vi "TestMain2.vi"(8 "error in (no error)":errorcluster) -> (0 "error in (out)":errorcluster)   [LabVIEW 2024, in "Test_2.lvlib"]
doc: "This template is for the Queued Message Handler design pattern.\n\nThe Event Handling Loop generates messages based on user interface actions.\n\nThe Message Handling Loop processes messages generated by the Event Handling Loop, or by other messages. The messages are string values, so new messages can be added easily to the Message Cases case structure in the Message Handling Loop. Each message cluster can also provide an optional value for Message Data, which is a variant that can be converted to whatever message-specific data is required."
uses:
  Test_2.lvlib
  Launcher/SubVI/Controls/OEE_CTRL.ctl
  controls/Test UI Data.ctl
  Settings/controls/Setting_Screen UI Data.ctl
  Settings/support/ScriptDetails.ctl
  Settings/support/CurrentStep.ctl
  Settings/support/StepType.ctl
  Settings/support/PS_WRITE.ctl
  Settings/support/PS_set.ctl
  Settings/support/DMM_CONFIG.ctl
  Settings/support/READ_DATAS.ctl
  Settings/support/READ_EQP.ctl
  Settings/support/READ_PARA.ctl
  Settings/support/Relay_Channel_Array.ctl
  Settings/support/Common_plc_DOs.ctl
  Settings/support/DAQ_Config.ctl
  PCANusb_DTU/support/CAN_MSGs.ctl
  PCANusb_DTU/support/CAN_Frames_ctrl.ctl
  PCANusb_DTU/support/Framing datas.ctl
  PCANusb_DTU/support/CAN_Read.ctl
  Settings/support/Camera.ctl
  MCU_Flashing/support/MCU_ctrl.ctl
  Settings/support/Neoway ctl.ctl
  Settings/support/SSL.ctl
  ADAM_DI/support/Relay_enum_IN.ctl
  Relay_Module/support/Relay_Enum_OUT.ctl
  <vilib>/Utility/miscctls.llb/LVRowAndColumnTypeDef.ctl
  <vilib>/Utility/miscctls.llb/LVMinMaxIncTypeDef.ctl
  <vilib>/Utility/miscctls.llb/LVRangeTypeDef.ctl
  Relay_Module/support/Relay_Channel_Write.ctl
  PrivateControls/Test_FGV_Queue_Control.ctl
  <vilib>/Utility/file.llb/Write Delimited Spreadsheet (string).vi
  Launcher/SubVI/Global 1.vi
  <vilib>/Utility/error.llb/Error Cluster From Error Code.vi
  <vilib>/regexp/Match Regular Expression.xnode
  <vilib>/ErrorRing/Error Ring.xnode
  support/Message Queue/Test Message Queue.lvlib
  support/User Event - Stop/Test User Event - Stop.lvlib
  Settings/Setting_Screen.lvlib
  Launcher/Launcher_DTU.lvlib
  Relay_Module/Relay_Module.lvlib
  Barcode_Scanner/Barcode_Scanner.lvlib
  PCANusb_DTU/PCANusb_DTU.lvlib
  ADAM_DI/ADAM_DI.lvlib
  MCU_Flashing/MCU_Flashing.lvlib
  Keyence/Keyence_VS150.lvlib
  SSL_Certification/SSL_Certification.lvlib
  FTPClient/FTPS.lvlib
  AWSEXE/AWSEXE.lvlib
panel:
  out "Total Time(s)":i32
  out "RX/RY":string
  in  "New/Old_Slot":bool
  out "result":bool
  in  "Config":string
  out "Barcodetime":u32
  out "Test Started?":bool
  out "DTU Inspection Data":string
  out "Relay":refnum<queue>
  out "PP":bool
  out "EOL/FCT":bool
  out "element":string
  out "Part Count":T1
  in  "Operator":string
  in  "Start Button":bool
  out "STATUS":bool
  out "Test Progress...":u8(slide) max=0 step=1 scale=-1.0..1.0
  out "Barcode":string
  out "Configs":string
  in  "DUT":i32=1
  in  "Table":string[][](table)
  out "queue name 2":string
  out "queue name":string
  in  "Abort":bool
  in  "Exit":bool
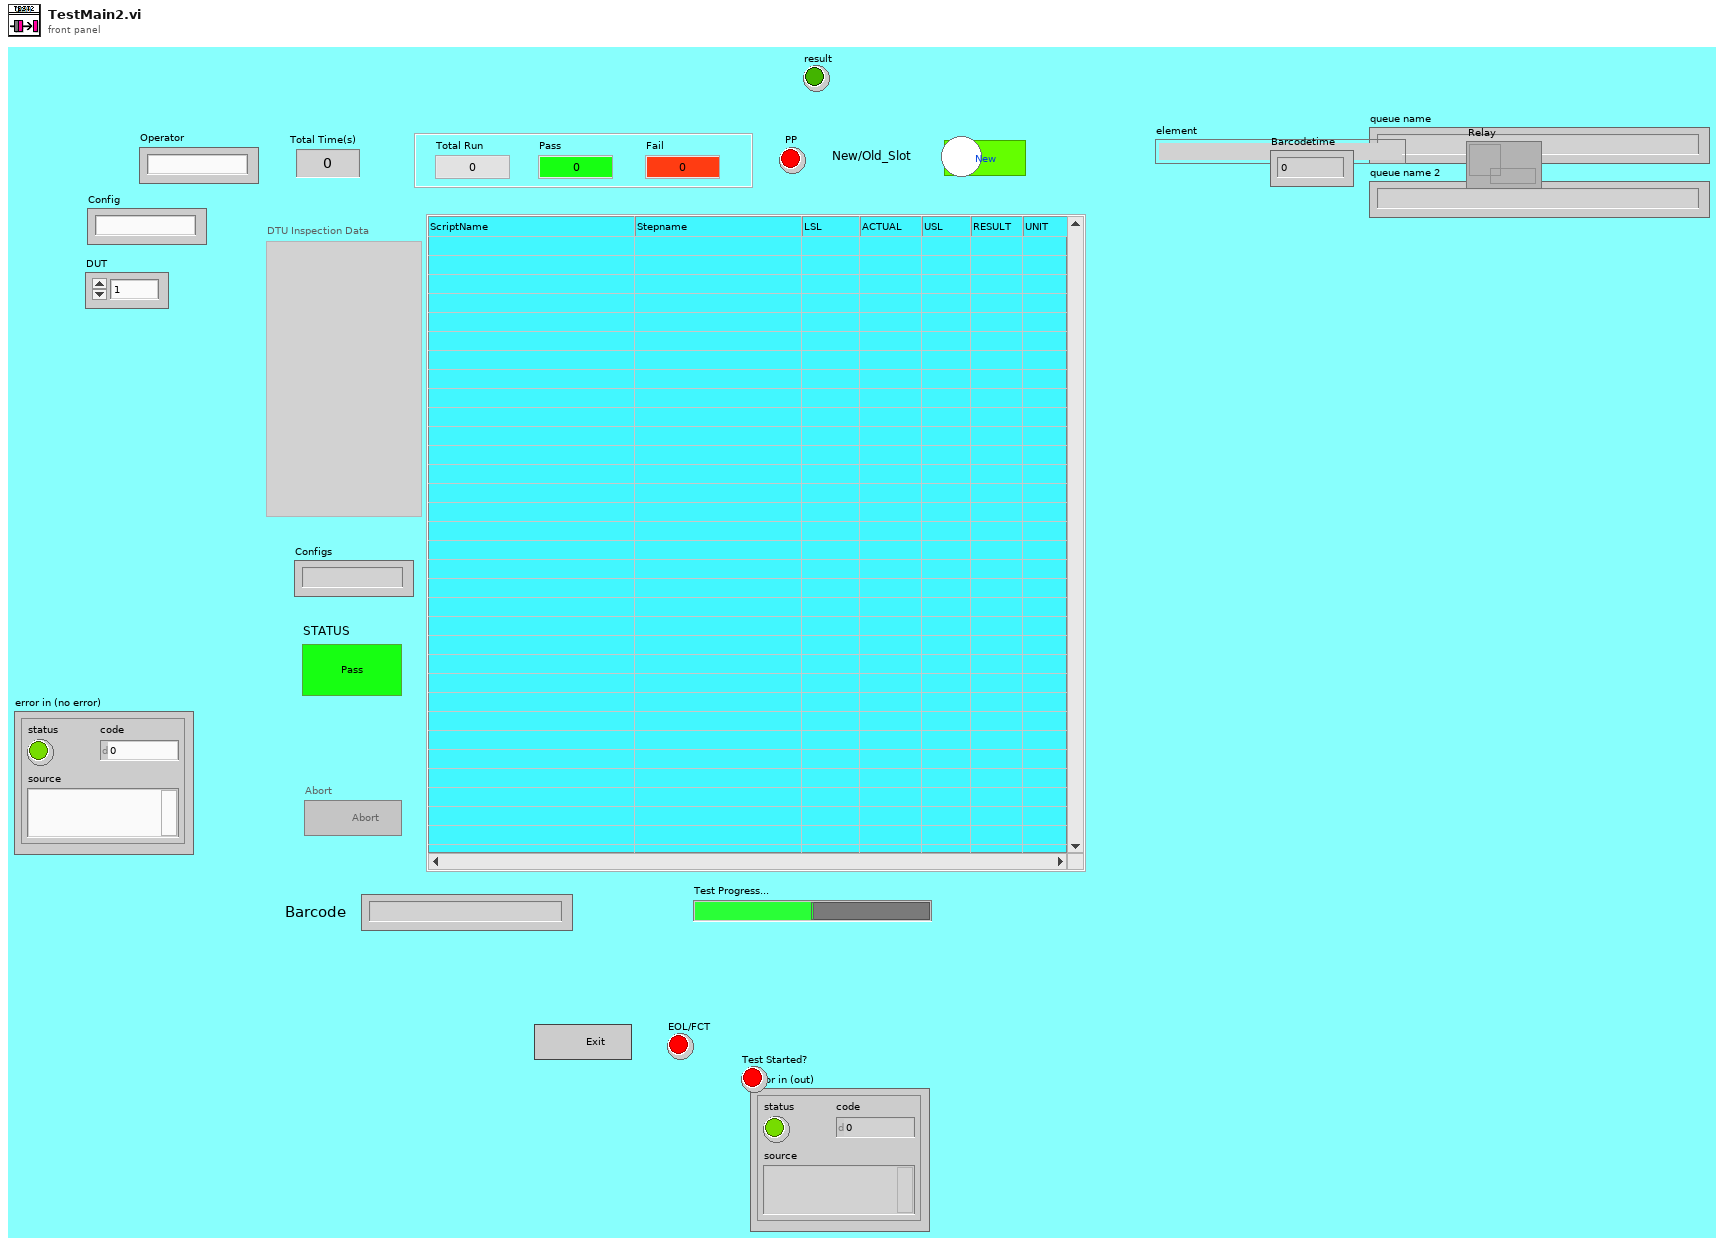
[diagram p1: front panel]
types:
  T1 = typedef "Launcher_DTU.lvlib/OEE_CTRL.ctl" = cluster{"Total Run":i32, "Pass":i32, "Fail":i32}
  T2 = typedef "Test_2.lvlib/Test UI Data.ctl" = cluster{"DUT":i32, "Pass/Fail":string, "Actual":string, "UI Data":T3, "Table":string[][], "Filename":string, "Test Started?":bool, "TotalScripts":u64, "Indexno.":u64, "Stepno.":u64, "TotalSteps":u64, "Scriptno.":u64, "Settings":path, "Data Path":path, "Configuration path":path, "Array_N":refnum<notifier>[], "Message Data":variant, "Stepname":string, "Scriptname":string, "Result":bool, "Header data":string[], "LaunchStep":bool, "Barcode":string, "LSL":string, "Delay":bool, "Delay time":dbl, "Operator":string, "Part Count ":T1, "InitPro":bool, "ResultS":string, "PMC path":path, "Test2_Q":refnum<queue>, "Array_Q":refnum<queue>[], "config":string, "EQUP LIST":string[], "EQUIP Config path":path, "Relay_Module_Q":refnum<queue>, "Barcode Scanned?":bool, "USL":string, "UNIT":string, "Expected_Value":string, "MACID":string, "ICCID":string, "IMEI":string, "Barcodetime":u32, "Seconds":u32, "RX/RY":string, "Selected_Scripts":T4[]}
  T3 = typedef "Setting_Screen.lvlib/Setting_Screen UI Data.ctl" = cluster{"Script_Tree":refnum<vi>, "Scripts":T4[], "ScriptDetails":T4, "Current Step":T5, "ScriptName":string, "StepName":string, "Children Symbols":i32[][], "Parrent Symbol":i32[], "Configurations:":string, "Config":string, "Scriptno.":i32, "PS_Write":T7, "DMM_CONFIG":T9, "READ_DATAS":T10, "Set_Channel_Relay":T13, "DAQ_Config":T15, "CAN_MSGs_Write":T16, "CAN_Read":T19, "Camera":T20, "Tab Control":refnum<vi>, "MCU Flashing":T21, "Noeway_Flashing":T22, "SSL":T23}
  T4 = typedef "Setting_Screen.lvlib/ScriptDetails.ctl" = cluster{"Script Name":string, "Steps":T5[]}
  T5 = typedef "Setting_Screen.lvlib/CurrentStep.ctl" = cluster{"StepName":string, "StepDetails":string, "Type":T6}
  T6 = typedef "Setting_Screen.lvlib/StepType.ctl" = enum16{"RELAY_CHANNEL_WRITE", "PS_WRITE", "READ_DATA", "DMM_CONFIG", "DAQ_CONFIG", "PCAN_Read", "PCAN_Write", "Camera", "MCU_Flashing", "Noeway_Flashing", "SSL_Certification"}
  T7 = typedef "Setting_Screen.lvlib/PS_WRITE.ctl" = cluster{"Set_parameter":T8, "VOLTAGE":string, "CURRENT":string, "OUTPUT":bool, "Delay":bool, "Delay time":dbl}
  T8 = typedef "Setting_Screen.lvlib/PS_set.ctl" = u16
  T9 = typedef "Setting_Screen.lvlib/DMM_CONFIG.ctl" = cluster{"CONFIG PARAMETER":u16, "AUTO RANGE":bool, "RANGE":string, "Delay":bool, "Delay time":dbl}
  T10 = typedef "Setting_Screen.lvlib/READ_DATAS.ctl" = cluster{"EQUIPMENT":T11, "PARAMETER":T12, "LSL":dbl, "USL":dbl, "RESULT":string, "UNIT":string, "Delay":bool, "Delay time":dbl}
  T11 = typedef "Setting_Screen.lvlib/READ_EQP.ctl" = u16
  T12 = typedef "Setting_Screen.lvlib/READ_PARA.ctl" = u16
  T13 = typedef "Setting_Screen.lvlib/Relay_Channel_Array.ctl" = cluster{"Relay_CH_Array":cluster{"OUTPUT_Relay_Channels":T14, "On/Off":bool}[]}
  T14 = typedef "Setting_Screen.lvlib/Common_plc_DOs.ctl" = u16
  T15 = typedef "Setting_Screen.lvlib/DAQ_Config.ctl" = cluster{"AUTO RANGE":bool, "CHANNEL LIST":string, "SELECT Card":u16, "SELECT SLOT":u16, "Function":i32}
  T16 = typedef "PCANusb_DTU.lvlib/CAN_MSGs.ctl" = cluster{"Scaling Factor":u16, "Physical value":dbl, "CAN_Frames":T17, "Offset value":dbl, "Framing datas":T18[], "CAN_Frame Enable":bool, "Add Signal":bool, "Delete Signal":bool, "Signal Values":dbl[], "Time(ms)":dbl, "Repetition":bool, "Delay":bool, "Delay time":dbl}
  T17 = typedef "PCANusb_DTU.lvlib/CAN_Frames_ctrl.ctl" = cluster{"CAN_ID":u32, "MSGTYPE":u8, "Payload":u8[], "Length":u8}
  T18 = typedef "PCANusb_DTU.lvlib/Framing datas.ctl" = cluster{"Signal name":string, "Start Bit":u8, "Length":u8, "Value":u16}
  T19 = typedef "PCANusb_DTU.lvlib/CAN_Read.ctl" = cluster{"Database":refnum<k21>, "Signal":refnum<k21>, "BYTES":u32[], "ReadPayload":u8[], "String_Data":string, "ReadValue":dbl, "CANID":u32, "SERVICE ID":u32, "SUB-SERVICE ID":u32, "DELAY ":bool, "Delay time(ms)":dbl}
  T20 = typedef "Setting_Screen.lvlib/Camera.ctl" = cluster{"Trigger":bool, "Prog No.":string, "Delay":bool, "Delay time":dbl, "Storage":string, "Col no.":string, "Row no.":string}
  T21 = typedef "MCU_Flashing.lvlib/MCU_ctrl.ctl" = cluster{"Result Path":path, "Result":string}
  T22 = typedef "Neoway ctl.ctl" = cluster{"Neoway_Firmware":path, "RESULT STRING":string, "Delay":bool, "Delay time":dbl}
  T23 = typedef "SSL.ctl" = cluster{"SSL_EXE":path, "RESULT STRING":string, "Delay":bool, "Delay time":dbl}
  T24 = typedef "Test_2.lvlib/Test_FGV_Queue_Control.ctl" = enum16{"Release", "Get", "Set", "Flush"}
  T25 = cluster{"Message":string, "Message Data":variant}
  T26 = typedef "Test_2.lvlib/Test Message Queue.lvlib/Test_All Message Queues.ctl" = cluster{"UI":refnum<queue>, "QSM":refnum<queue>}
  T27 = typedef "ADAM_DI.lvlib/Relay_enum_IN.ctl" = enum16{"EMERGENCY", "CONTROL ON", "START DUT 1", "START DUT 2", "STOP DUT 1", "STOP DUT 2", "PPS DUT 1", "PPS DUT 2", "REED CYL UP DUT 1", "REED CYL DOWN DUT 1", "REED CYL UP DUT 2", "REED CYL DOWN DUT 2", "LIGHT CURTAIN"}
  T28 = typedef "Relay_Module.lvlib/Relay_Enum_OUT.ctl" = enum16{"CONN_SUPPLY_%d_FCT", "HB_CONN_%d_FCT", "L_IND_CONN_%d_FCT", "R_IND_CONN_%d_FCT", "SW1_%d_FCT", "SW2_%d_FCT", "CAN_H_%d_FCT", "CAN_L_%d_FCT", "CYLINDER_ON/OFF_%d_FCT", "SPARE_1_%d_FCT", "SPARE_2_%d_FCT", "Tower Red", "Tower Amber", "Tower Green", "Tower Buzzer", "SLIMRELAY_DUT_%d_FCT", "GND_DMM_%d_EOL", "CAN_H_RES_%d_EOL", "CAN_L_RES_%d_EOL", "L_IND_RES_%d_EOL", "R_IND_RES_%d_EOL", "HB_CONN_DMM_%d_EOL", "14V_RES_%d_EOL", "CAN_L_(DMM-)_%d_EOL", "CAN_H_%d_EOL", "CAN_L_%d_EOL", "14V_%d_EOL", "GND_%d_EOL", "HB_CONN_%d_EOL", "L_IND_%d_EOL", "R_IND_%d_EOL", "CYLINDER_DUT_%d_EOL", "CYL_PB_1_%d_EOL", "CYL_PB_2_%d_EOL", "DUT_PASS_%d_EOL", "DUT_FAIL_%d_EOL", "SPARE1_%d_EOL", "Tower Red_EOL", "Tower Amber_EOL", "Tower Green_EOL", "Tower Buzzer_EOL"}
  T29 = enum16{"Read", "Write", "All_sections", "All_values", "Remove key&section"}
  T30 = typedef "LVRowAndColumnTypeDef.ctl" = cluster{"Row":i32, "Column":i32}
  T31 = enum8{"Enabled", "Disabled", "Disabled and Grayed Out"}
  T32 = typedef "LVRangeTypeDef.ctl" = cluster{"Minimum":dbl, "Maximum":dbl, "Increment":dbl, "Minor Increment":dbl, "Start":dbl}
  T33 = typedef "LVMinMaxIncTypeDef.ctl" = cluster{"Minimum":dbl, "Maximum":dbl, "Increment":dbl}
  T34 = cluster{"Status":string, "Free/inuse":bool, "Action":string}
  T35 = cluster{"On/Off":bool, "OUTPUT_Relay_Channels":T28}[]
  T36 = typedef "Relay_Module.lvlib/Relay_Channel_Write.ctl" = cluster{"Relay_CH_Array":cluster{"On/Off":bool, "OUTPUT_Relay_Channels":T28}[]}
  T37 = enum16{"open", "replace", "create", "open or create", "replace or create", "replace or create with confirmation"}
  T38 = cluster{"Result":bool, "DTU_Inspection_Data":string}
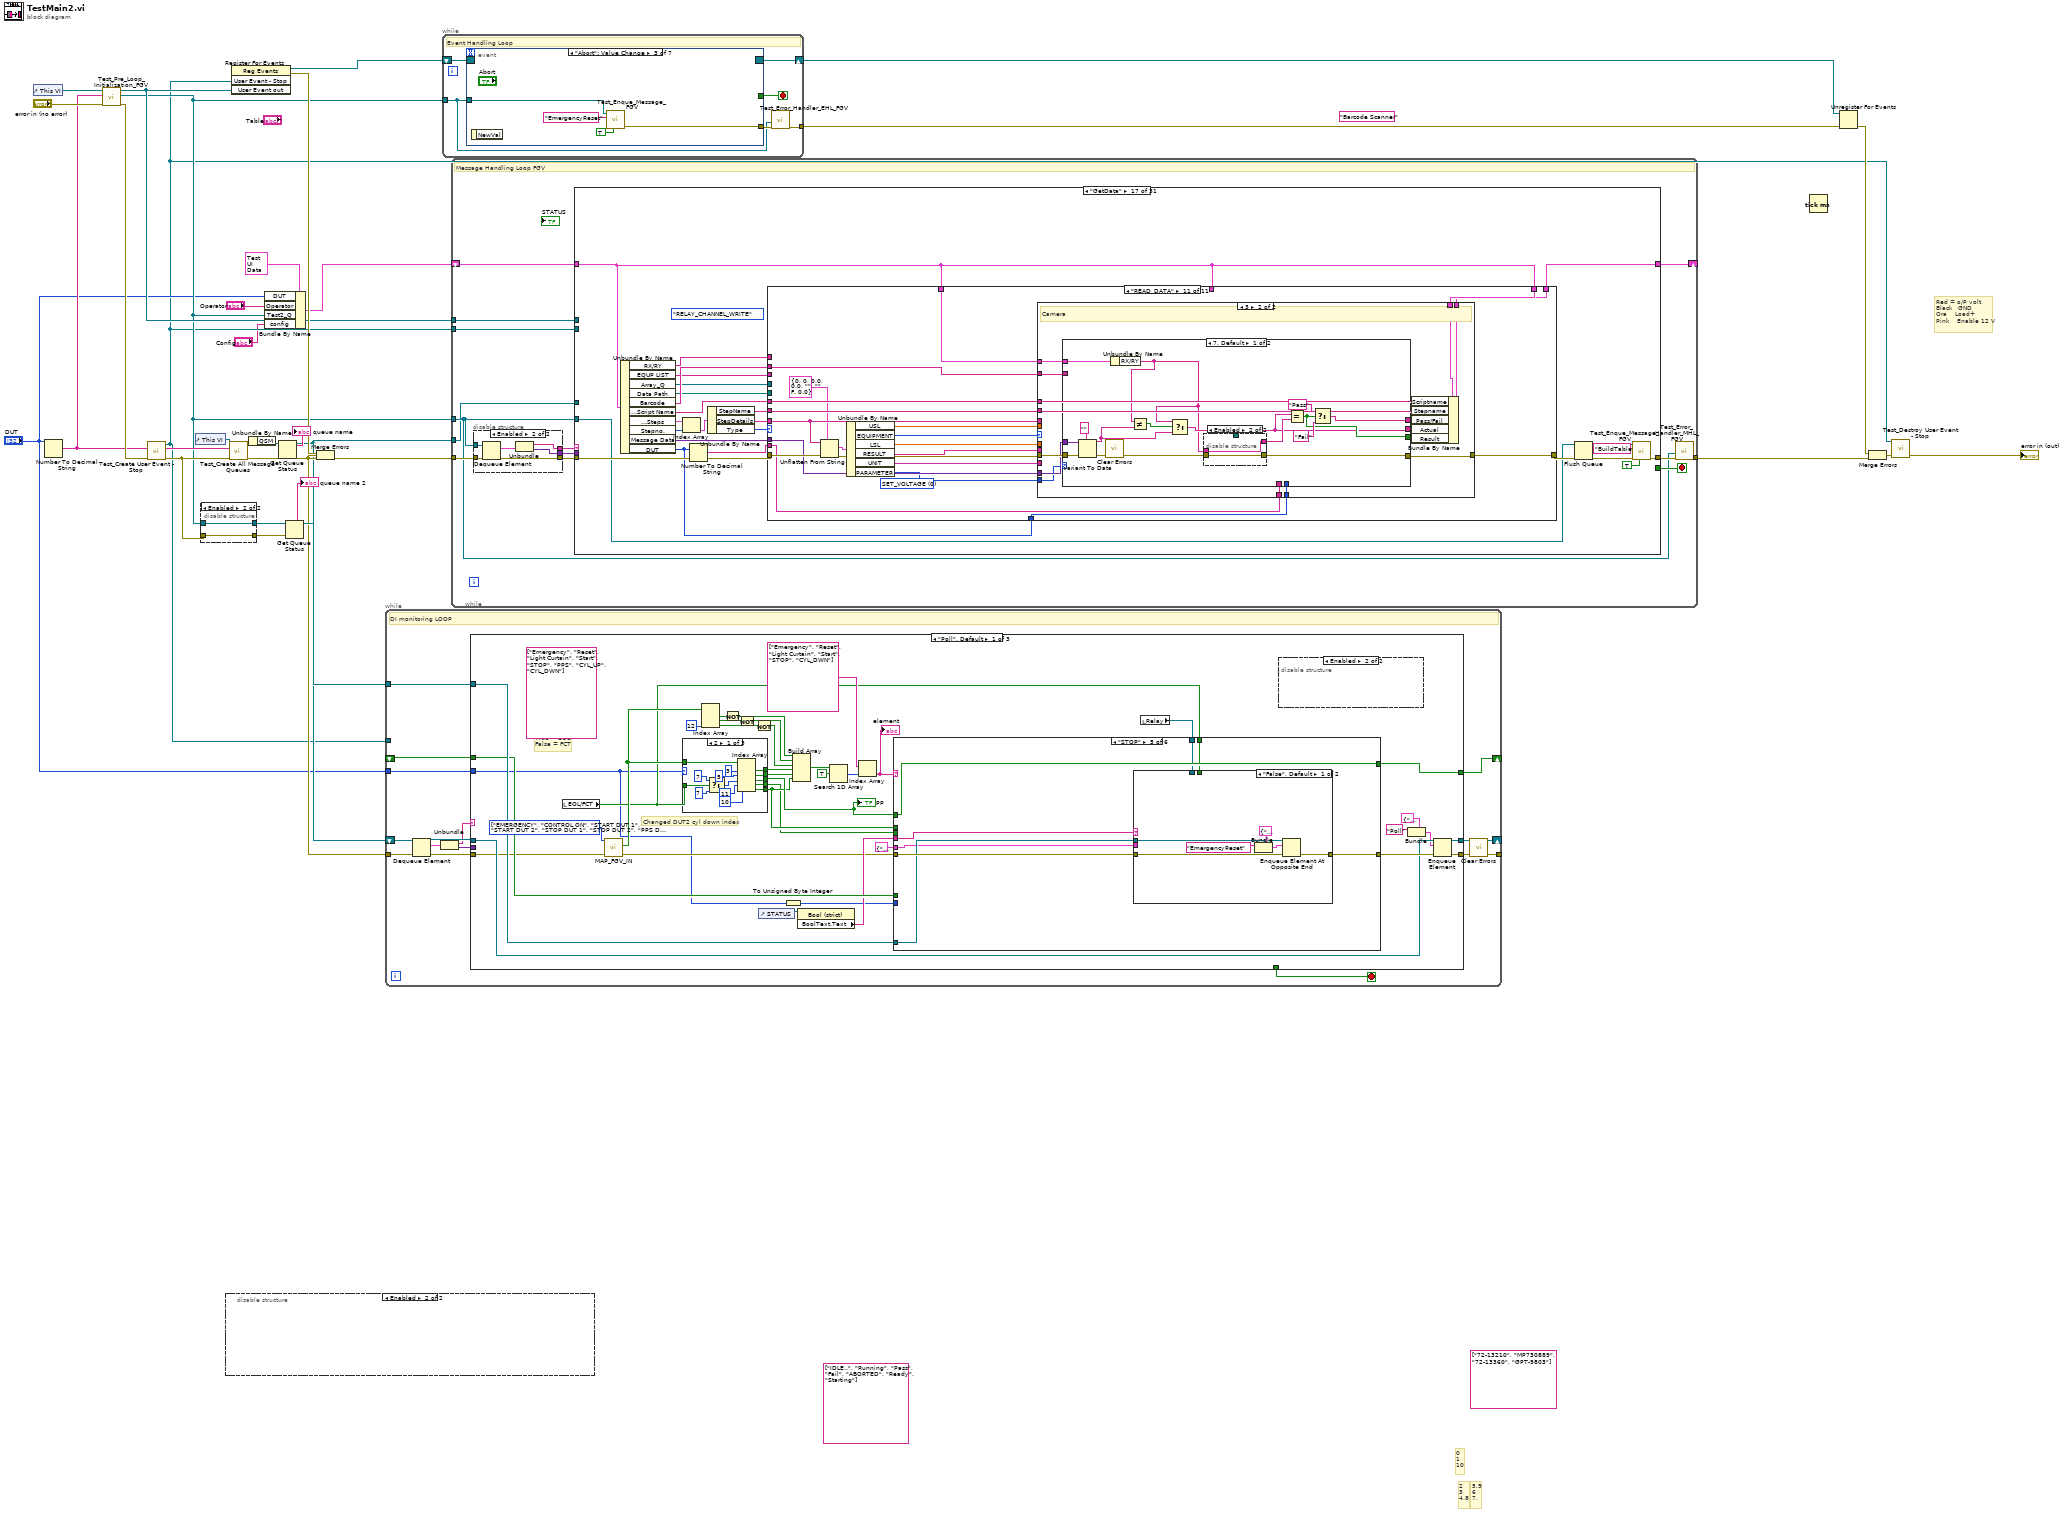
[diagram p0: block diagram]
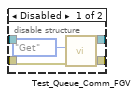
[diagram p2: hidden frame]
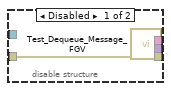
[diagram p3: hidden frame]
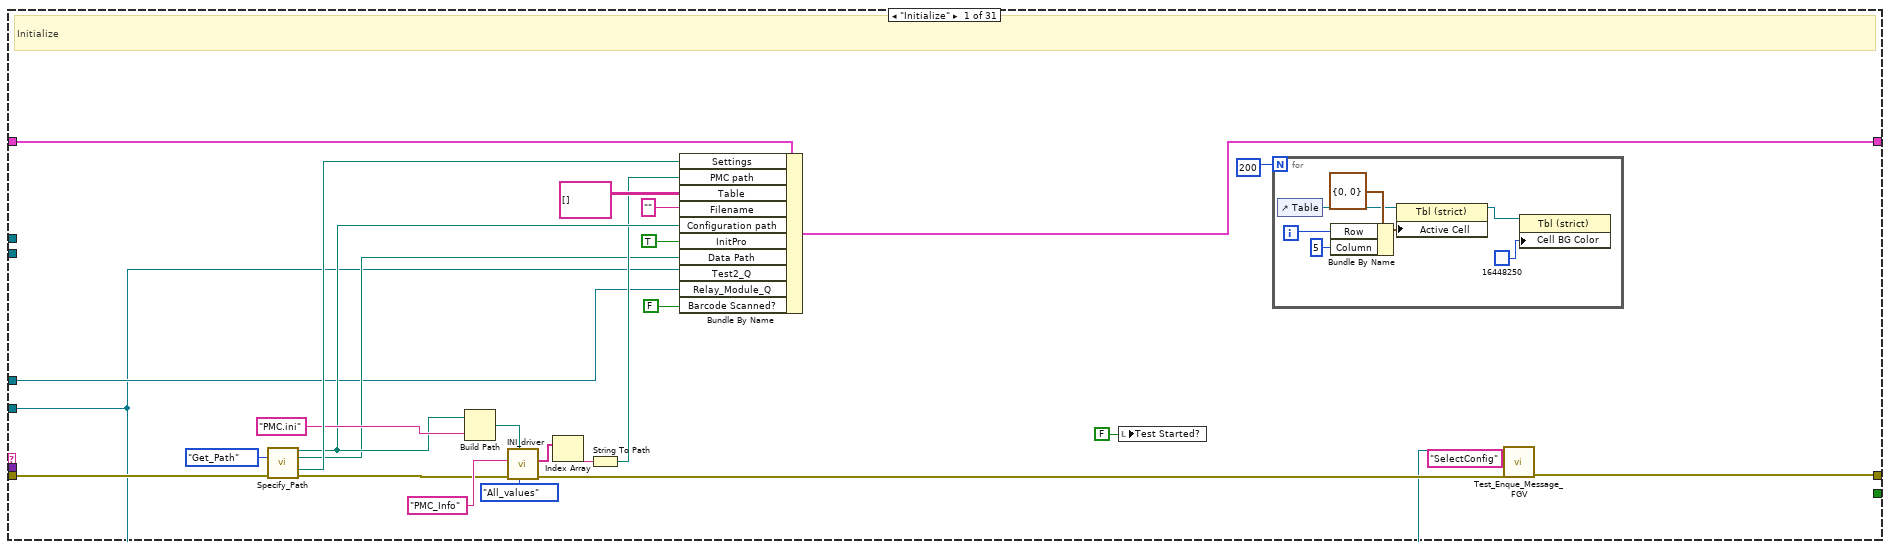
[diagram p4: hidden frame]
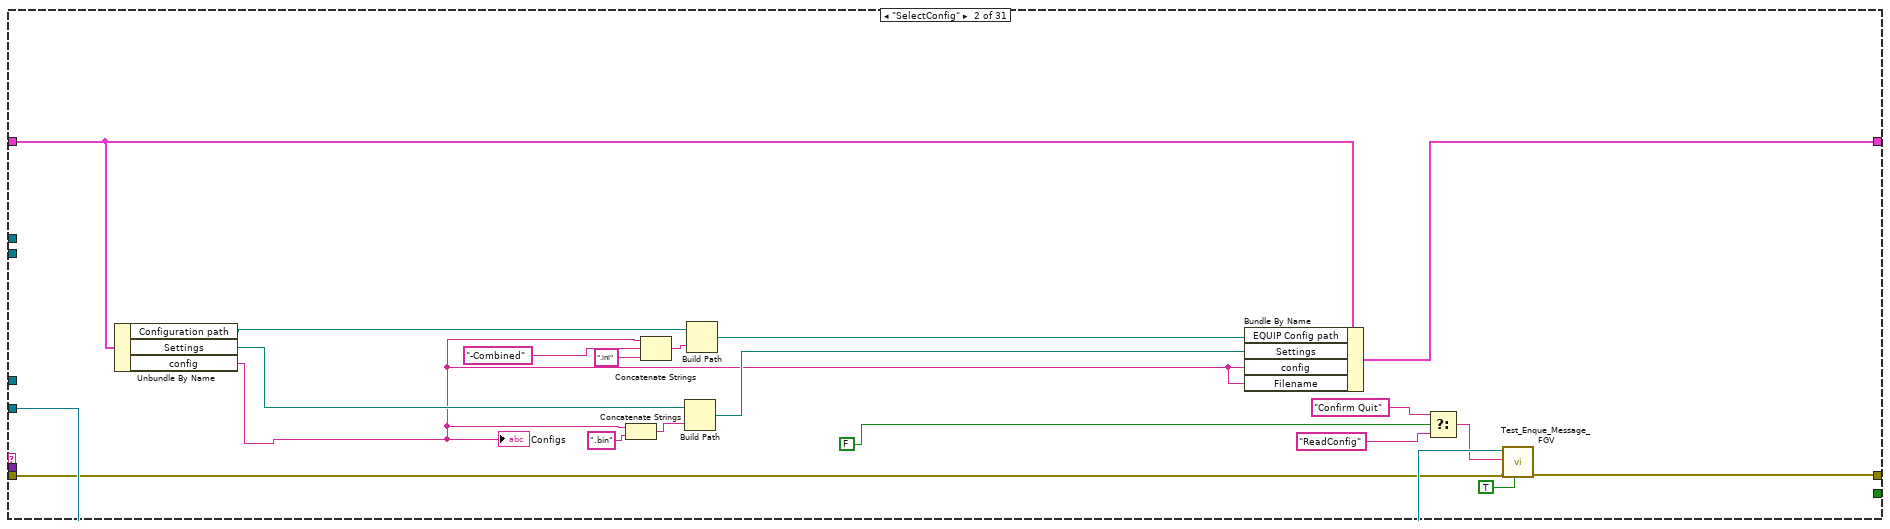
[diagram p5: hidden frame]
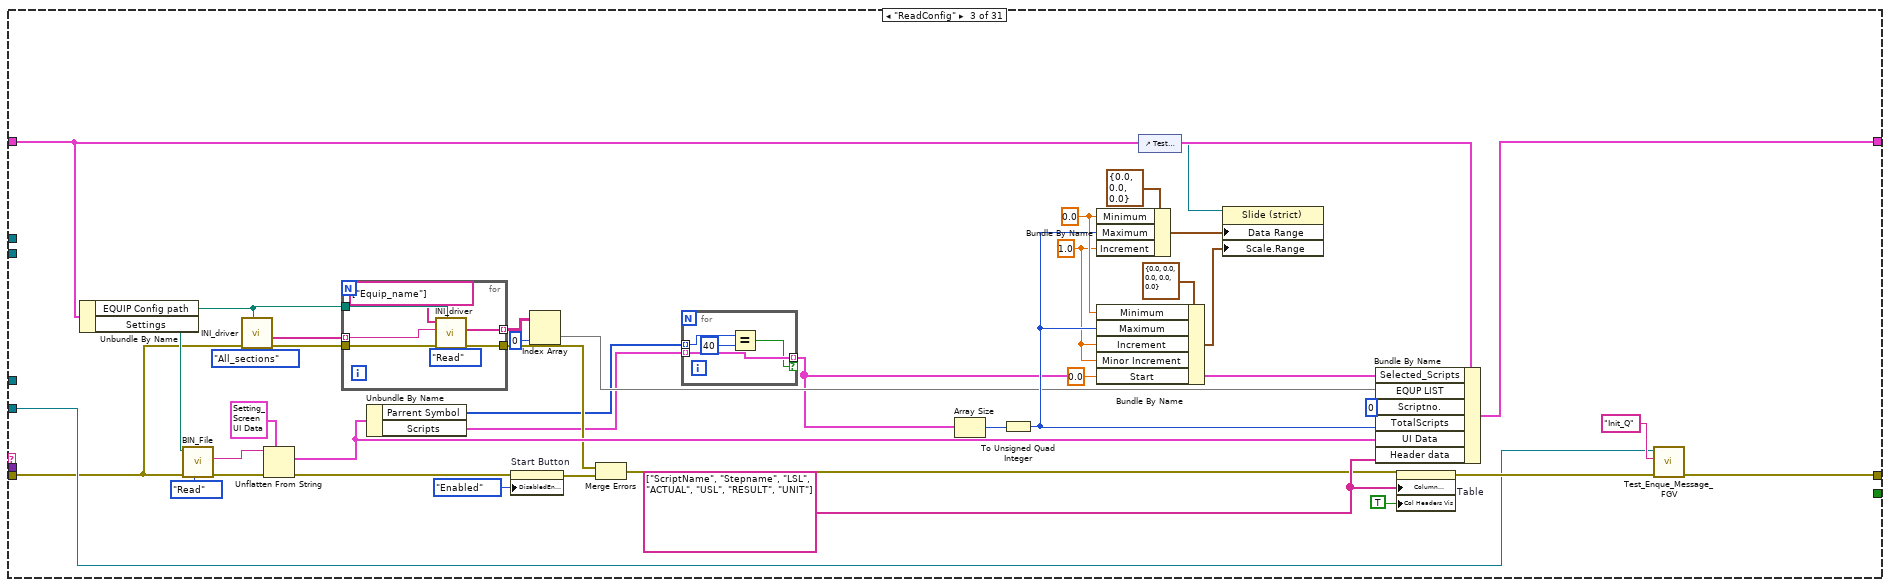
[diagram p6: hidden frame]
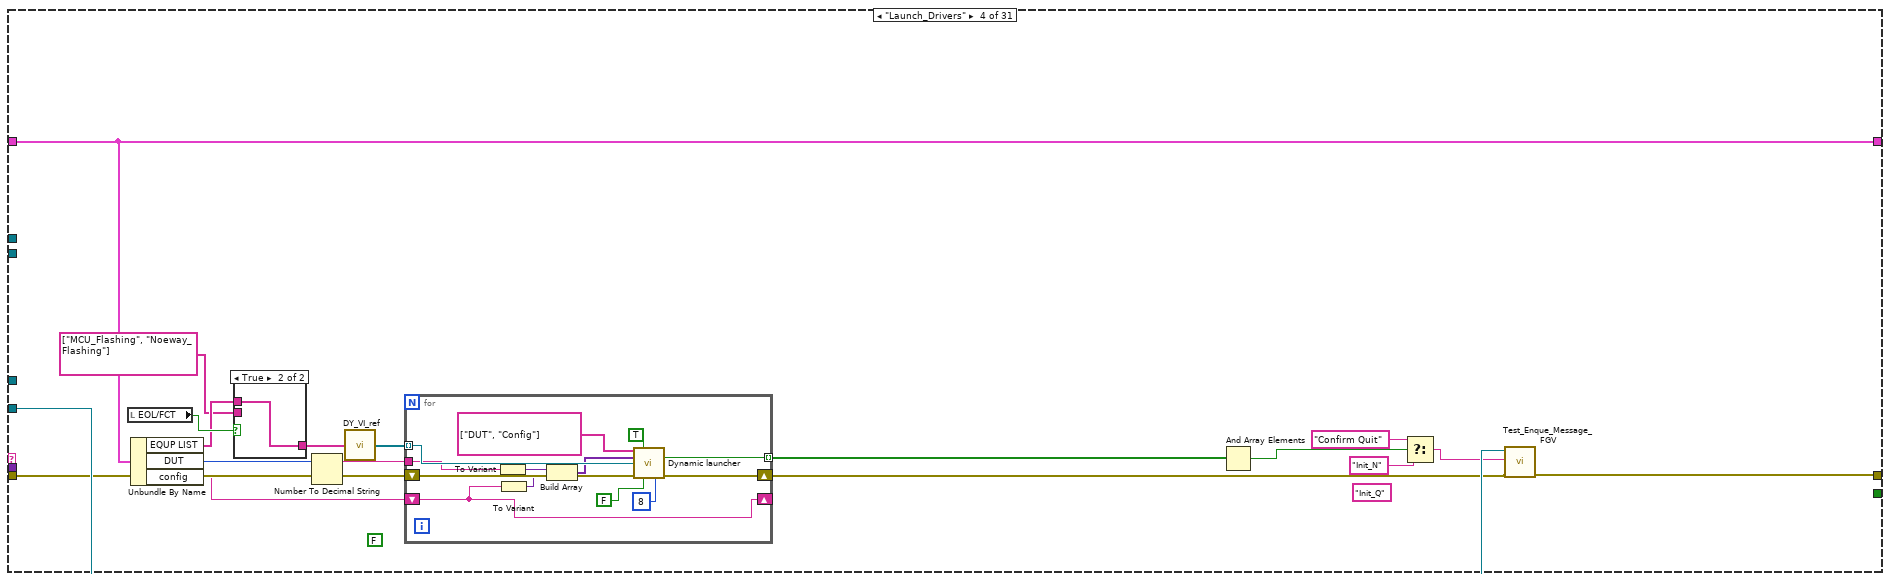
[diagram p7: hidden frame]
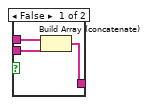
[diagram p8: hidden frame]
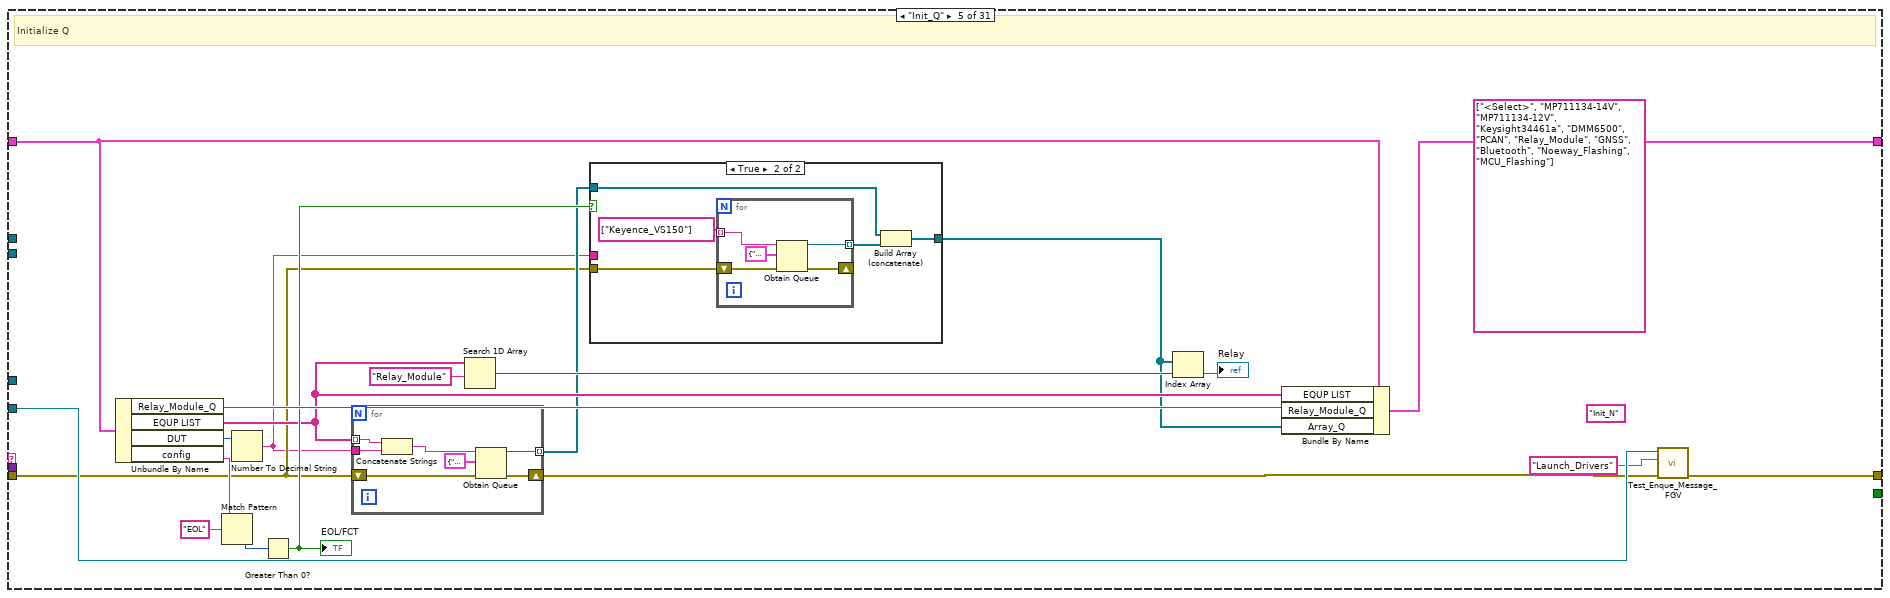
[diagram p9: hidden frame]
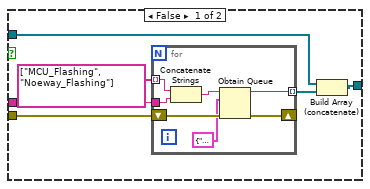
[diagram p10: hidden frame]
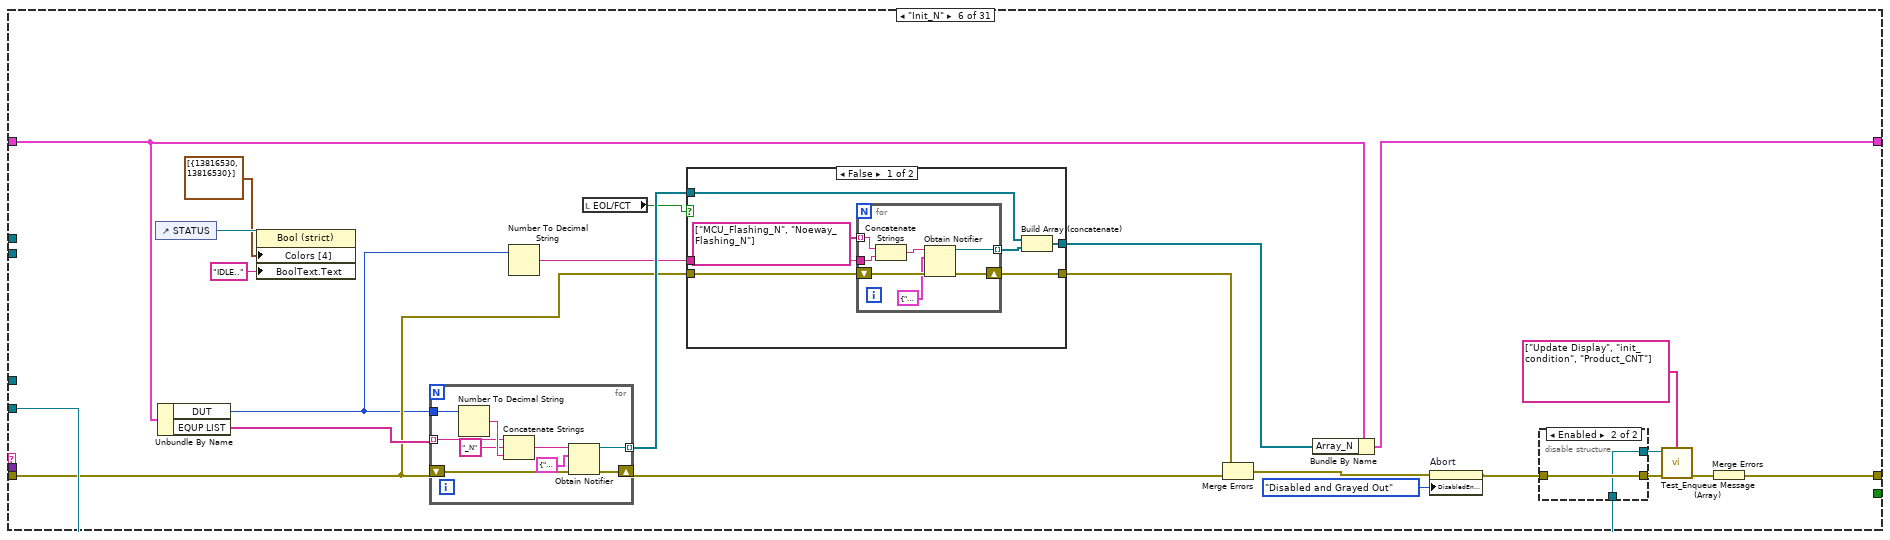
[diagram p11: hidden frame]
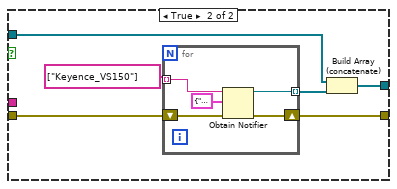
[diagram p12: hidden frame]
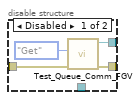
[diagram p13: hidden frame]
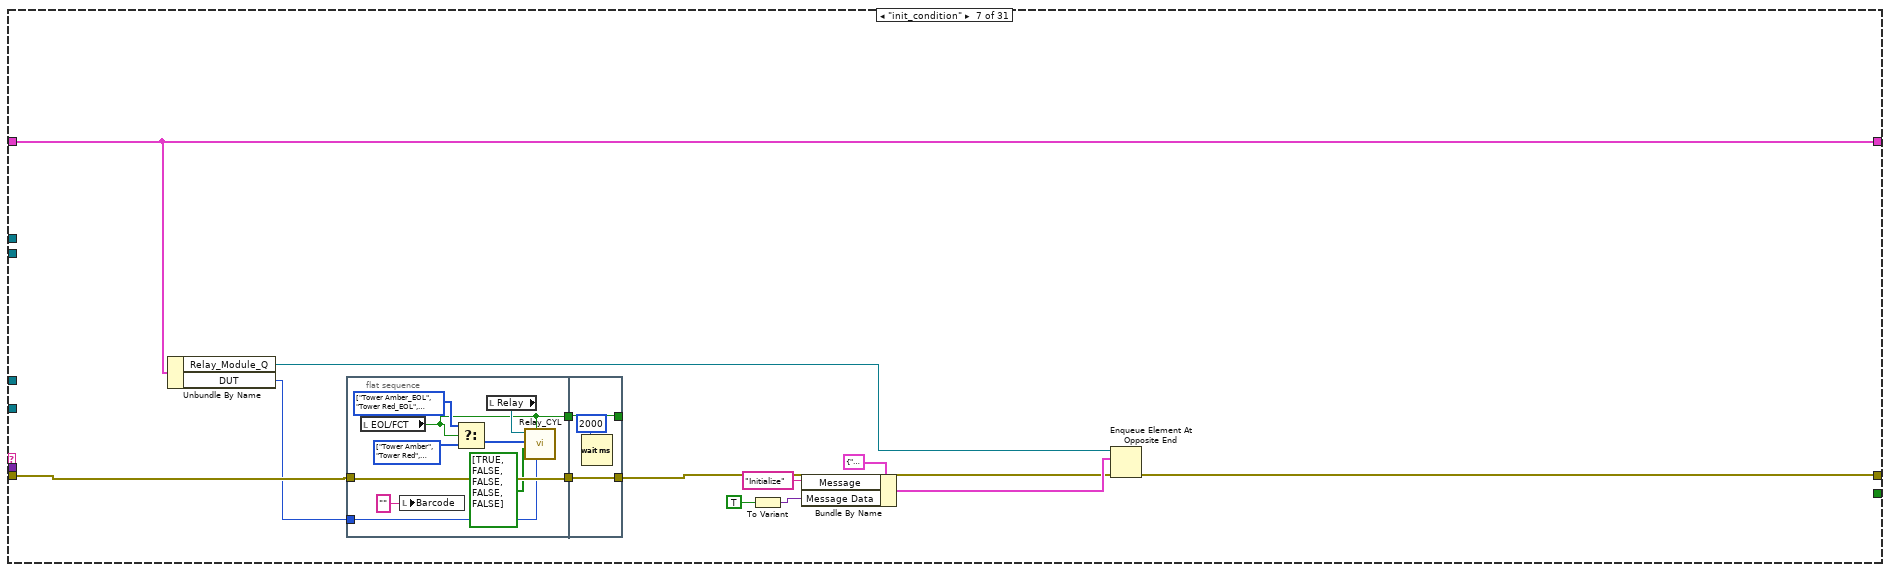
[diagram p14: hidden frame]
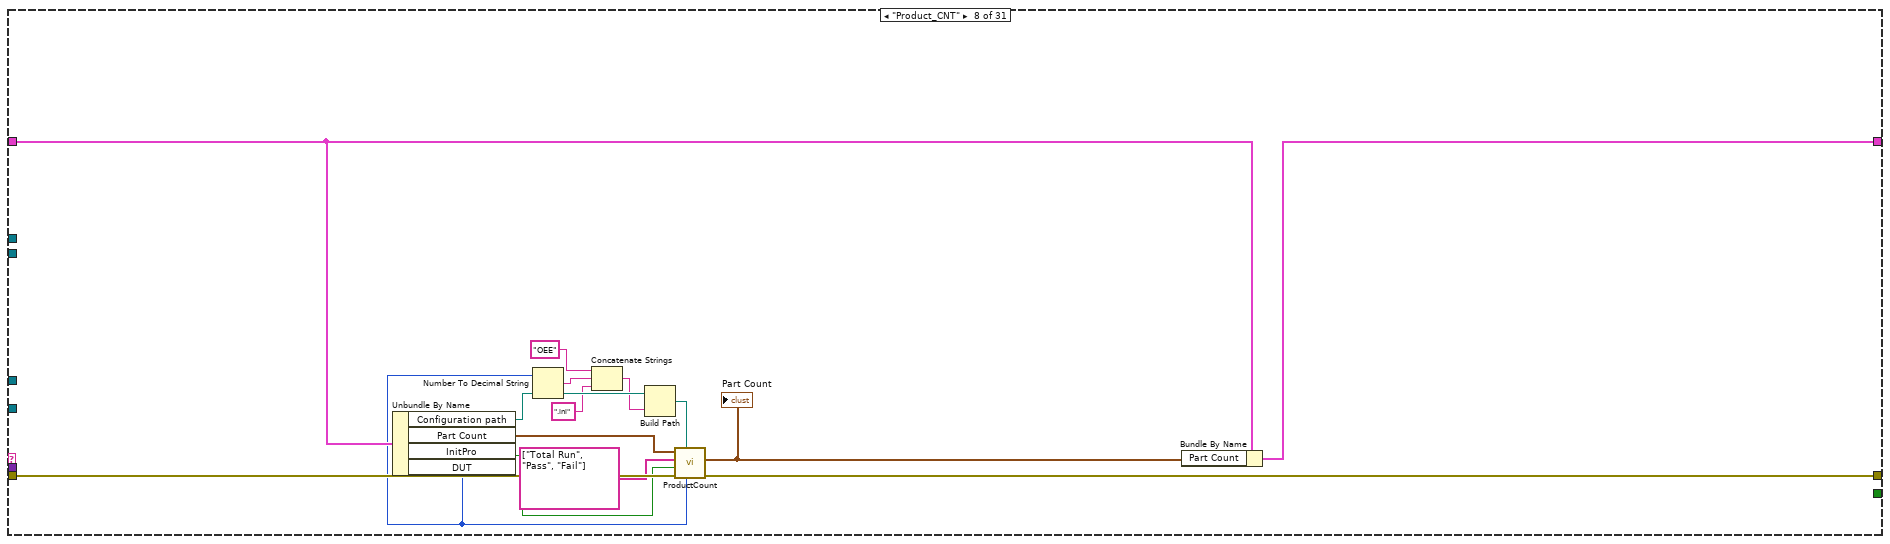
[diagram p15: hidden frame]
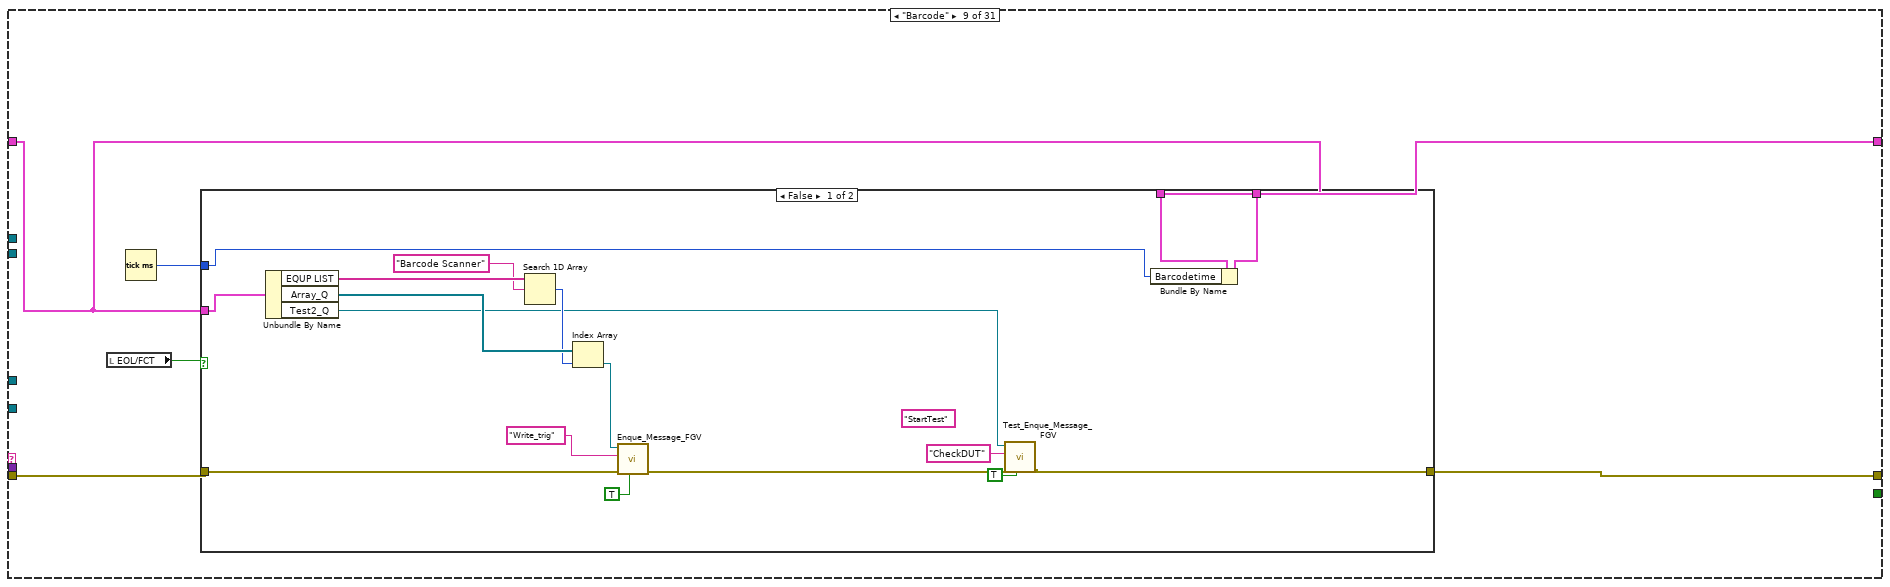
[diagram p16: hidden frame]
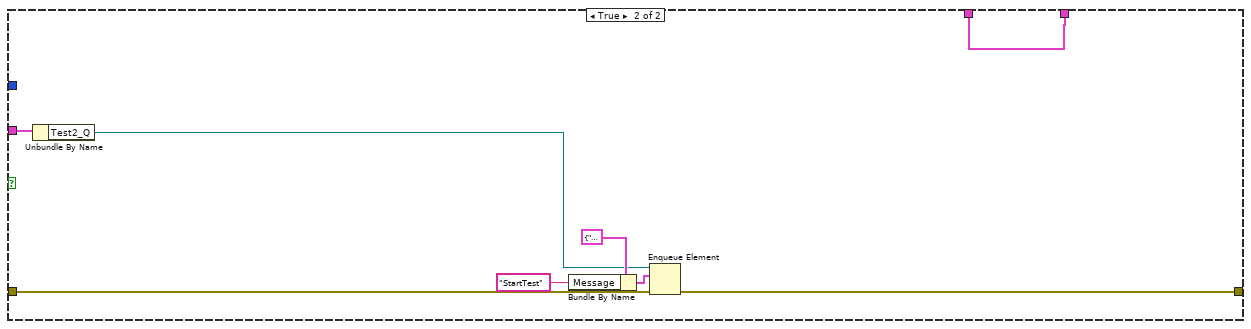
[diagram p17: hidden frame]
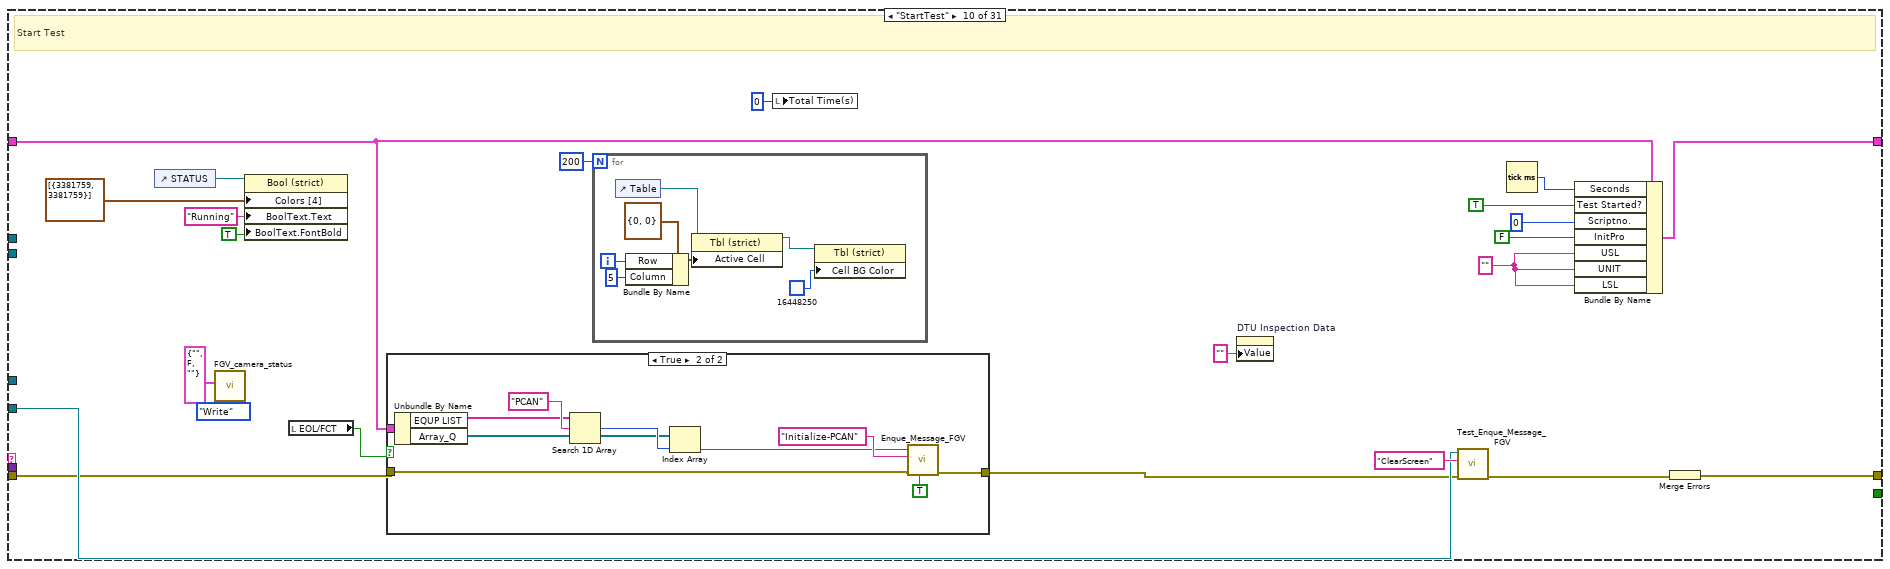
[diagram p18: hidden frame]
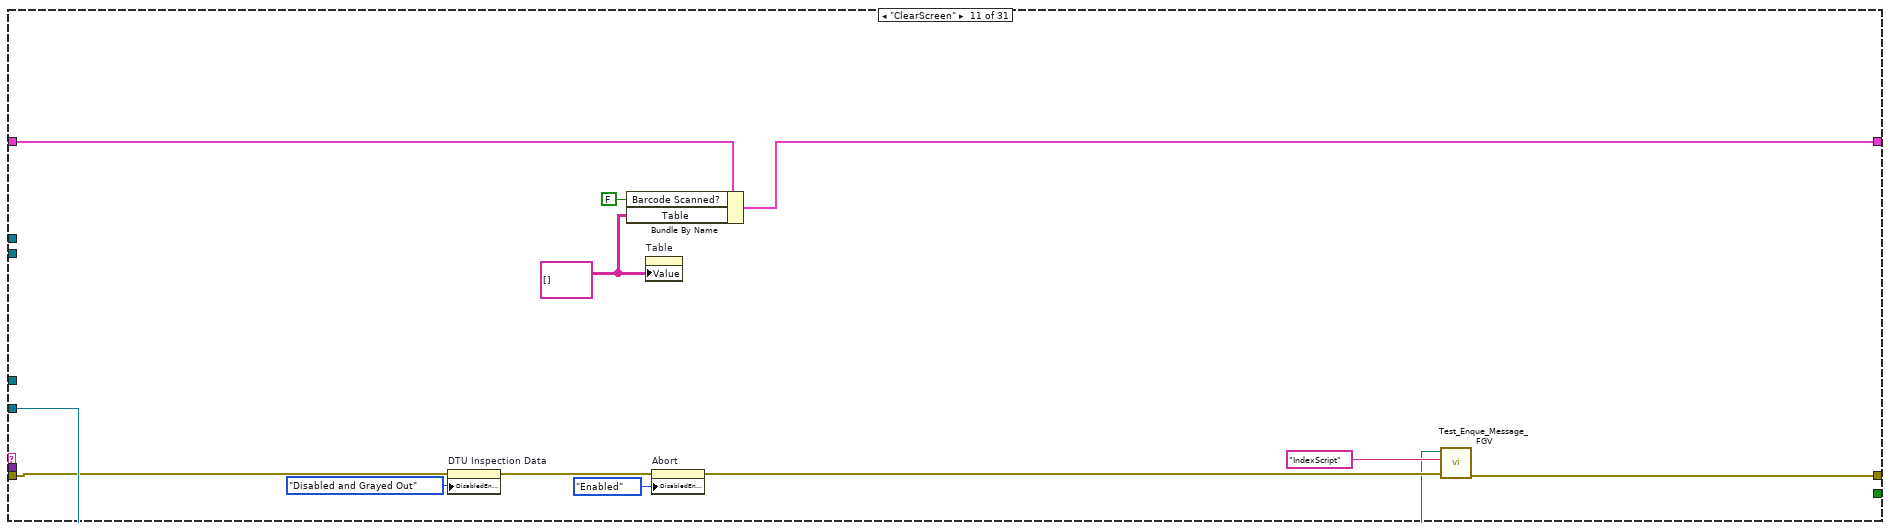
[diagram p20: hidden frame]
diagram:
  (unwired) "Barcode Scanner"
  (unwired) string[] ["IDLE..", "Running", "Pass", "Fail", "ABORTED", "Ready", "Starting"]
  (unwired) string[] ["72-13210", "MP730889", "72-13360", "GPT-9803"]
  # "Red = o/P volt\nBlack   GND\nOra    Load+\nPink    Enable 12 V"
  # "5,9\n6\n7,"
  # "2\n3\n4,8"
  # "0\n1\n10"
  n1 = control-ref of="This VI"() -> (w20:refnum<vi>)
  n2 = Number To Decimal String(number="DUT") -> (decimal integer string=w10:string)  [unwired: 1 in]
  n3 = call "Test_Pre_Loop_Initialization_FGV.vi"("error in (no error)"="error in (no error)", "DUT"=w10, "VI in"=w20) -> ("error out"=w18:errorcluster, "queue out"=w6:refnum<queue>, "User Event out"=w11:refnum<user-event>)  [unwired: 6 in]
  n4 = call "Test_Create User Event - Stop.vi"("error in (no error)"=w18) -> ("error out"=w14:errorcluster, "User Event - Stop"=w2:refnum<user-event>)  [unwired: 9 in]
  n5 = control-ref of="This VI"() -> (w16:refnum<vi>)
  n6 = disable-structure shown="Enabled" {
    disable-tunnel: w14 -> [w36 w38]
    disable-tunnel: [w34 w37] -> w13
    disable-tunnel: [w33 w38] -> w7
    disable-tunnel: w6 -> [_ w37]
    frame Disabled {
      n7 = call "Test_Queue_Comm_FGV.vi"("error in (no error)"=w36, "Enum"=Test_FGV_Queue_Control."Get") -> ("error Out"=w33:errorcluster, "queue Out"=w34:refnum<queue>)  [unwired: 8 in]
    }
    frame Enabled {
    }
  }
  n8 = disable-structure shown="Enabled" {
    frame Disabled {
      n9 = To Variant() -> (Variant=w46:variant)  [unwired: 1 in]
      n10 = Select(t="Error" ("f"), f="Read" ("Message")) -> (s? t:f=w41:string)  [unwired: 1 in]
      n11 = Bundle By Name(cluster=T25 {"Message"="", "Message Data"=variant} ("notification"), "Message"=w41, "Message Data"=w46) -> ()  [unwired: 1 out]
      n12 = Select(t="Error" ("f"), f="Step_Done" ("Message")) -> (s? t:f=w44:string)  [unwired: 1 in]
      n13 = Bundle By Name(cluster=T25 {"Message"="", "Message Data"=variant} ("notification"), "Message"=w44) -> ()  [unwired: 1 out]
    }
    frame Enabled {
    }
  }
  n14 = call "Test_Create All Message Queues.vi"("error in (no error)"=w14, "DUT"=w10, "This VI"=w16) -> ("error out"=w31:errorcluster, "Message Queues out"=w30:T26)  [unwired: 7 in]
  n15 = register-events(w2, w11) -> (reference out=w22:refnum<event-registration>, error out=w21:errorcluster)  [unwired: 2 in]
  n16 = Unbundle By Name(w30) -> ("QSM"=w28:refnum<queue>)
  n17 = Bundle By Name(cluster=T2 {"DUT"=1, "Pass/Fail"="", "Actual"="", "UI Data"={"Script_Tree"=refnum, "Scripts"=[], "ScriptDetails"={"Script Name"="", "Steps"=[]}, "Current Step"={"StepName"="", "StepDetails"="", "Type"=enum."RELAY_CHANNEL_WRITE"}, "ScriptName"="", "StepName"="", "Children Symbols"=[], "Parrent Symbol"=[], "Configurations:"="", "Config"="", "Scriptno."=0, "PS_Write"={"Set_parameter"=0, "VOLTAGE"="", "CURRENT"="", "OUTPUT"=FALSE, "Delay"=FALSE, "Delay time"=0.0}, "DMM_CONFIG"={"CONFIG PARAMETER"=0, "AUTO RANGE"=FALSE, "RANGE"="", "Delay"=FALSE, "Delay time"=0.0}, "READ_DATAS"={"EQUIPMENT"=0, "PARAMETER"=0, "LSL"=0.0, "USL"=0.0, "RESULT"="", "UNIT"="", "Delay"=FALSE, "Delay time"=0.0}, "Set_Channel_Relay"={"Relay_CH_Array"=[]}, "DAQ_Config"={"AUTO RANGE"=FALSE, "CHANNEL LIST"="", "SELECT Card"=0, "SELECT SLOT"=0, "Function"=0}, "CAN_MSGs_Write"={"Scaling Factor"=0, "Physical value"=0.0, "CAN_Frames"={"CAN_ID"=0, "MSGTYPE"=0, "Payload"=[], "Length"=0}, "Offset value"=0.0, "Framing datas"=[], "CAN_Frame Enable"=FALSE, "Add Signal"=FALSE, "Delete Signal"=FALSE, "Signal Values"=[], "Time(ms)"=0.0, "Repetition"=FALSE, "Delay"=FALSE, "Delay time"=0.0}, "CAN_Read"={"Database"="", "Signal"="", "BYTES"=[], "ReadPayload"=[], "String_Data"="", "ReadValue"=0.0, "CANID"=0, "SERVICE ID"=0, "SUB-SERVICE ID"=0, "DELAY "=FALSE, "Delay time(ms)"=0.0}, "Camera"={"Trigger"=FALSE, "Prog No."="", "Delay"=FALSE, "Delay time"=0.0, "Storage"="", "Col no."="", "Row no."=""}, "Tab Control"=refnum, "MCU Flashing"={"Result Path"=path "", "Result"=""}, "Noeway_Flashing"={"Neoway_Firmware"=path "", "RESULT STRING"="", "Delay"=FALSE, "Delay time"=0.0}, "SSL"={"SSL_EXE"=path "", "RESULT STRING"="", "Delay"=FALSE, "Delay time"=0.0}}, "Table"=[], "Filename"="", "Test Started?"=FALSE, "TotalScripts"=0, "Indexno."=0, "Stepno."=0, "TotalSteps"=0, "Scriptno."=0, "Settings"=path "", "Data Path"=path "", "Configuration path"=path "", "Array_N"=[], "Message Data"=variant, "Stepname"="", "Scriptname"="", "Result"=FALSE, "Header data"=[], "LaunchStep"=FALSE, "Barcode"="", "LSL"="", "Delay"=FALSE, "Delay time"=0.0, "Operator"="", "Part Count "={"Total Run"=0, "Pass"=0, "Fail"=0}, "InitPro"=FALSE, "ResultS"="", "PMC path"=path "", "Test2_Q"=refnum, "Array_Q"=[], "config"="", "EQUP LIST"=[], "EQUIP Config path"=path "", "Relay_Module_Q"=refnum, "Barcode Scanned?"=FALSE, "USL"="", "UNIT"="", "Expected_Value"="", "MACID"="", "ICCID"="", "IMEI"="", "Barcodetime"=0, "Seconds"=0, "RX/RY"="", "Selected_Scripts"=[]} ("Data Cluster"), "DUT"="DUT", "Operator"="Operator", "Test2_Q"=w6, "config"="Config") -> (w9:T2)
  n18 = Get Queue Status(queue=w28) -> (queue out=w4:refnum<queue>, queue name=→"queue name":string)  [unwired: 2 in, 6 out]
  n19 = Get Queue Status(queue=w13, error in (no error)=w7) -> (queue out=w32:refnum<queue>, queue name=→"queue name 2":string)  [unwired: 1 in, 6 out]
  n20 = Merge Errors(w21, w31) -> (w5:errorcluster)
  n21 = while {
    shift-right: [w53] -> _
    shift-left: w4 -> [w60]
    tunnel: w32 -> [w52]
    tunnel: "DUT" -> [w51]
    tunnel: w5 -> [w62]
    tunnel: [w50] -> _
    tunnel: w2 -> [_]
    shift-right: [w49] -> _
    shift-left: _ -> [w48]
    stop <- w54 stop-if-true
    # "DI monitoring LOOP"
    n22 = Dequeue Element(queue=w60, error in (no error)=w62) -> (queue out=w58:refnum<queue>, element=w59:T25, error out=w61:errorcluster)  [unwired: 1 in, 1 out]
    n23 = Unbundle(w59) -> ("Message"=w56:string, "Message Data"=w57:variant)
    n24 = case shown="\"Poll\", Default" w56 {
      tunnel: w61 -> [w72 w386 w395]
      tunnel: w58 -> [w84 w384 w393]
      tunnel: w57 -> [_ _ w389]
      tunnel: [w85 w385 w394] -> w55
      tunnel: [_ TRUE _] -> w54
      tunnel: [w83 refnum<queue> refnum ("QSM") w392] -> w53
      tunnel: w52 -> [w88 _ _]
      tunnel: w51 -> [w66 _ _]
      tunnel: [w76 FALSE ("Boolean") _] -> w49
      tunnel: w48 -> [w75 _ _]
      frame "Poll", Default {
        (unwired) string[] ["Emergency", "Reset", "Light Curtain", "Start", "STOP", "PPS", "CYL_UP", "CYL_DWN"]
        w69 = T27[] [enum."EMERGENCY", enum."CONTROL ON", enum."START DUT 1", enum."START DUT 2", enum."STOP DUT 1", enum."STOP DUT 2", enum."PPS DUT 1", enum."PPS DUT 2", enum."REED CYL UP DUT 1", enum."REED CYL DOWN DUT 1", enum."REED CYL UP DUT 2", enum."REED CYL DOWN DUT 2", enum."LIGHT CURTAIN"] items=["EMERGENCY", "CONTROL ON", "START DUT 1", "START DUT 2", "STOP DUT 1", "STOP DUT 2", "PPS DUT 1", "PPS DUT 2", "REED CYL UP DUT 1", "REED CYL DOWN DUT 1", "REED CYL UP DUT 2", "REED CYL DOWN DUT 2", "LIGHT CURTAIN"] ("PLC_BOOL_IN")
        # "Changed DUT2 cyl down index"
        # "True = EOL\nFalse = FCT"
        n25 = local read "EOL/FCT"() -> (w67:bool)
        n26 = call "MAP_FGV_IN.vi"("error in (no error)"=w72, "Relay_ENUM_IN"=w69) -> ("error out"=w71:errorcluster, "DOs_out"=w70:bool[])  [unwired: 7 in, 1 out]
        n27 = case shown="2" w66 {
          tunnel: w70 -> [w366 _ w381]
          tunnel: w67 -> [w363 _ w380]
          tunnel: [w360 w367 w375] -> w96
          tunnel: [w359 w367 w374] -> w95
          tunnel: [w358 w367 w373] -> w74
          tunnel: [w356 w367 w369] -> w63
          tunnel: [w355 w367 w368] -> w64
          frame 2 {
            n28 = Select(t=7 ("index"), s=w363, f=7 ("index")) -> (s? t:f=w357:i32)
            n29 = Index Array(array=w366, index #1=3 ("index"), index #2=5 ("index"), index #3=w357, index #4=11 ("index"), index #5=10 ("index")) -> (element #1=w360:bool, element #2=w359:bool, element #3=w358:bool, element #4=w356:bool, element #5=w355:bool)
          }
          frame Default {
            w367 = FALSE ("Boolean")
          }
          frame 1 {
            n30 = Select(t=6 ("index"), s=w380, f=6 ("index")) -> (s? t:f=w372:i32)
            n31 = Index Array(array=w381, index #1=2 ("index"), index #2=4 ("index"), index #3=w372, index #4=8 ("index"), index #5=9 ("index")) -> (element #1=w375:bool, element #2=w374:bool, element #3=w373:bool, element #4=w369:bool, element #5=w368:bool)
          }
        }
        "PP" <- w74
        n32 = Index Array(array=w70, index #3=12 ("index")) -> (element #1=w99:bool, element #2=w98:bool, element #3=w97:bool)  [unwired: 2 in]
        n33 = Not(x=w99) -> (.not. x?=w94:bool)
        n34 = Not(x=w98) -> (.not. x?=w78:bool)
        n35 = Not(x=w97) -> (.not. x?=w77:bool)
        n36 = control-ref of="STATUS"() -> (w79:refnum<vi>)
        n37 = To Unsigned Byte Integer(number=w66) -> (unsigned 8bit integer=w65:u8)
        n38 = Build Array(w94, w78, w77, w96, w95, w64) -> (w90:bool[])
        n39 = property class="Bool (strict)"(reference=w79) -> ("BoolText.Text"=w73:string)  [unwired: 1 in, 2 out]
        n40 = Search 1D Array(1D array=w90, element=TRUE) -> (index of element=w91:i32)  [unwired: 1 in]
        n41 = Index Array(array=string[] ["Emergency", "Reset", "Light Curtain", "Start", "STOP", "CYL_DWN"], index=w91) -> (element=w87:string)
        "element" <- w87
        n42 = local read "Relay"() -> (w68:refnum<queue>)
        n43 = case shown="\"STOP\"" w87 {
          tunnel: w71 -> [w113 w168 w205 w244 w271 w300]
          tunnel: [w112 w167 w204 w243 w270 w299] -> w89
          tunnel: w88 -> [w111 w166 w203 w242 w269 w298]
          tunnel: T25 {"Message"="", "Message Data"=variant} ("element") -> [w110 w165 w202 w241 w268 w295]
          tunnel: w74 -> [w109 w164 w199 w238 w266 w296]
          tunnel: w73 -> [w108 w163 w201 w240 w267 w297]
          tunnel: [w107 w162 w199 w238 w266 w294] -> w76
          tunnel: w75 -> [_ _ w200 w239 _ _]
          tunnel: w68 -> [w106 w161 w198 w237 w265 w291]
          tunnel: w67 -> [w104 w159 w197 w236 w264 w290]
          tunnel: w64 -> [w105 w160 _ _ _ _]
          tunnel: w65 -> [w103 _ _ _ _ w293]
          tunnel: w63 -> [_ _ _ _ _ w292]
          frame "Start" {
            n44 = case shown="True" w109 {
              selector: w109 -> [w114 w119]
              tunnel: w113 -> [w115 w124]
              tunnel: [w115 w123] -> w112
              tunnel: w111 -> [_ w122]
              tunnel: w110 -> [_ w121]
              tunnel: w108 -> [_ w120]
              tunnel: [w114 w119] -> w107
              tunnel: w106 -> [_ w118]
              tunnel: w105 -> [_ _]
              tunnel: w104 -> [_ w117]
              tunnel: w103 -> [_ w116]
              frame False {
              }
              frame True {
                n45 = case shown="\"IDLE..\", \"Ready\"" w120 {
                  tunnel: w124 -> [w125 w131]
                  tunnel: [w125 w138] -> w123
                  tunnel: w122 -> [_ w127]
                  tunnel: w121 -> [_ _]
                  tunnel: w118 -> [_ w137]
                  tunnel: w117 -> [_ w129]
                  tunnel: w116 -> [_ w136]
                  frame Default {
                  }
                  frame "IDLE..", "Ready" {
                    w133 = T28[] [enum."CYLINDER_ON/OFF_%d_FCT", enum."SPARE_1_%d_FCT", enum."SPARE_2_%d_FCT"] items=["CONN_SUPPLY_%d_FCT", "HB_CONN_%d_FCT", "L_IND_CONN_%d_FCT", "R_IND_CONN_%d_FCT", "SW1_%d_FCT", "SW2_%d_FCT", "CAN_H_%d_FCT", "CAN_L_%d_FCT", "CYLINDER_ON/OFF_%d_FCT", "SPARE_1_%d_FCT", "SPARE_2_%d_FCT", "Tower Red", "Tower Amber", "Tower Green", "Tower Buzzer", "SLIMRELAY_DUT_%d_FCT", "GND_DMM_%d_EOL", "CAN_H_RES_%d_EOL", "CAN_L_RES_%d_EOL", "L_IND_RES_%d_EOL", "R_IND_RES_%d_EOL", "HB_CONN_DMM_%d_EOL", "14V_RES_%d_EOL", "CAN_L_(DMM-)_%d_EOL", "CAN_H_%d_EOL", "CAN_L_%d_EOL", "14V_%d_EOL", "GND_%d_EOL", "HB_CONN_%d_EOL", "L_IND_%d_EOL", "R_IND_%d_EOL", "CYLINDER_DUT_%d_EOL", "CYL_PB_1_%d_EOL", "CYL_PB_2_%d_EOL", "DUT_PASS_%d_EOL", "DUT_FAIL_%d_EOL", "SPARE1_%d_EOL", "Tower Red_EOL", "Tower Amber_EOL", "Tower Green_EOL", "Tower Buzzer_EOL"] ("Relay_Channel_Out")
                    w135 = T28[] [enum."CYLINDER_DUT_%d_EOL", enum."CYL_PB_1_%d_EOL", enum."CYL_PB_2_%d_EOL"] items=["CONN_SUPPLY_%d_FCT", "HB_CONN_%d_FCT", "L_IND_CONN_%d_FCT", "R_IND_CONN_%d_FCT", "SW1_%d_FCT", "SW2_%d_FCT", "CAN_H_%d_FCT", "CAN_L_%d_FCT", "CYLINDER_ON/OFF_%d_FCT", "SPARE_1_%d_FCT", "SPARE_2_%d_FCT", "Tower Red", "Tower Amber", "Tower Green", "Tower Buzzer", "SLIMRELAY_DUT_%d_FCT", "GND_DMM_%d_EOL", "CAN_H_RES_%d_EOL", "CAN_L_RES_%d_EOL", "L_IND_RES_%d_EOL", "R_IND_RES_%d_EOL", "HB_CONN_DMM_%d_EOL", "14V_RES_%d_EOL", "CAN_L_(DMM-)_%d_EOL", "CAN_H_%d_EOL", "CAN_L_%d_EOL", "14V_%d_EOL", "GND_%d_EOL", "HB_CONN_%d_EOL", "L_IND_%d_EOL", "R_IND_%d_EOL", "CYLINDER_DUT_%d_EOL", "CYL_PB_1_%d_EOL", "CYL_PB_2_%d_EOL", "DUT_PASS_%d_EOL", "DUT_FAIL_%d_EOL", "SPARE1_%d_EOL", "Tower Red_EOL", "Tower Amber_EOL", "Tower Green_EOL", "Tower Buzzer_EOL"] ("Relay_Channel_Out")
                    n46 = case shown="False" w129 {
                      selector: w129 -> [w141 w156]
                      tunnel: w131 -> [w145 w157]
                      tunnel: [w144 w157] -> w130
                      tunnel: [w140 w156] -> w128
                      tunnel: w127 -> [w139 _]
                      frame False {
                        n47 = flat-sequence {
                          tunnel: w145 -> [w149]
                          tunnel: [w148] -> w143
                          tunnel: [w147] -> w142
                          tunnel: w141 -> [w147]
                          tunnel: w139 -> [w146]
                          tunnel: [w155] -> w144
                          tunnel: w143 -> [w155]
                          tunnel: w142 -> [w154]
                          tunnel: [w154] -> w140
                          frame #0 {
                            n48 = Bundle(cluster=T25 {"Message"="", "Message Data"=variant} ("element"), "Message"="Barcode") -> (w152:T25)  [unwired: 1 in]
                            n49 = Enqueue Element At Opposite End(queue=w146, element=w152, error in (no error)=w149) -> (error out=w148:errorcluster)  [unwired: 1 in, 2 out]
                          }
                          frame #1 {
                            n50 = Wait (ms)(milliseconds to wait=u32 1000) -> ()  [unwired: 1 out]
                          }
                        }
                      }
                      frame True {
                      }
                    }
                    n51 = Select(t=w135, s=w128, f=w133) -> (s? t:f=w134:T28[])
                    n52 = call "Relay_CYL.vi"("DUT"=w136, "EOL/FCT"=w128, "error out"=w130, "DOs"=bool[] [TRUE, FALSE, FALSE], "Relay_Channel_Out"=w134, "Relay"=w137) -> ("error out 2"=w138:errorcluster)  [unwired: 5 in]
                    "Test Started?" <- TRUE ("Test Started?")
                  }
                }
              }
            }
          }
          frame "CYL_DWN" {
            n53 = local read "Test Started?"() -> (w158:bool)
            n54 = case shown="True" w164 {
              selector: w164 -> [w169 w173]
              tunnel: w168 -> [w170 w178]
              tunnel: [w170 w177] -> w167
              tunnel: w166 -> [_ w176]
              tunnel: w165 -> [_ w175]
              tunnel: w163 -> [_ w174]
              tunnel: [w169 w173] -> w162
              tunnel: w161 -> [_ _]
              tunnel: w160 -> [_ _]
              tunnel: w159 -> [_ w172]
              tunnel: w158 -> [_ w171]
              frame False {
              }
              frame True {
                n55 = case shown="\"IDLE..\", \"Ready\"" w174 {
                  tunnel: w178 -> [w179 w184]
                  tunnel: [w179 w183] -> w177
                  tunnel: w176 -> [_ w182]
                  tunnel: w175 -> [_ _]
                  tunnel: w172 -> [_ w181]
                  tunnel: w171 -> [_ w180]
                  frame Default {
                  }
                  frame "IDLE..", "Ready" {
                    n56 = case shown="True" w180 {
                      tunnel: w184 -> [w185 w196]
                      tunnel: [w185 w195] -> w183
                      tunnel: w182 -> [_ w194]
                      tunnel: w181 -> [_ w186]
                      frame False {
                      }
                      frame True {
                        n57 = control-ref of="STATUS"() -> (w190:refnum<vi>)
                        n58 = Select(t="Barcode" ("Message"), s=w186, f="CheckDUT" ("Message")) -> (s? t:f=w188:string)
                        n59 = property class="Bool (strict)"(reference=w190, "BoolText.Text"="Starting" ("Boolean Text.Text")) -> ()  [unwired: 1 in, 2 out]
                        n60 = Bundle(cluster=T25 {"Message"="", "Message Data"=variant} ("element"), "Message"=w188) -> (w193:T25)  [unwired: 1 in]
                        n61 = Enqueue Element At Opposite End(queue=w194, element=w193, error in (no error)=w196) -> (error out=w195:errorcluster)  [unwired: 1 in, 2 out]
                      }
                    }
                  }
                }
              }
            }
          }
          frame "Emergency" {
            n62 = case shown="\"ABORTED\", \"Fail\", \"Pass\", Default" w201 {
              tunnel: w205 -> [w210 w235]
              tunnel: [w208 w234] -> w204
              tunnel: w203 -> [w207 w233]
              tunnel: w202 -> [_ _]
              tunnel: w200 -> [w209 _]
              tunnel: w199 -> [w206 _]
              tunnel: w198 -> [_ w228]
              tunnel: w197 -> [_ w227]
              frame "ABORTED", "Fail", "Pass", Default {
                n63 = Not Equal?(x=w206, y=w209) -> (x != y?=w211:bool)
                n64 = case shown="True" w211 {
                  tunnel: w210 -> [w212 w216]
                  tunnel: [w212 w215] -> w208
                  tunnel: w207 -> [_ w214]
                  tunnel: w206 -> [_ w213]
                  frame False {
                  }
                  frame True {
                    n65 = case shown="False" w213 {
                      tunnel: w216 -> [w222 w223]
                      tunnel: [w221 w223] -> w215
                      tunnel: w214 -> [w217 _]
                      frame False {
                        n66 = Bundle(cluster=T25 {"Message"="", "Message Data"=variant} ("element"), "Message"="Reset") -> (w218:T25)  [unwired: 1 in]
                        n67 = Enqueue Element At Opposite End(queue=w217, element=w218, error in (no error)=w222) -> (error out=w221:errorcluster)  [unwired: 1 in, 2 out]
                      }
                      frame True {
                      }
                    }
                  }
                }
              }
              frame "Running" {
                w224 = T28[] [enum."Tower Red", enum."Tower Amber", enum."Tower Green", enum."Tower Buzzer"] items=["CONN_SUPPLY_%d_FCT", "HB_CONN_%d_FCT", "L_IND_CONN_%d_FCT", "R_IND_CONN_%d_FCT", "SW1_%d_FCT", "SW2_%d_FCT", "CAN_H_%d_FCT", "CAN_L_%d_FCT", "CYLINDER_ON/OFF_%d_FCT", "SPARE_1_%d_FCT", "SPARE_2_%d_FCT", "Tower Red", "Tower Amber", "Tower Green", "Tower Buzzer", "SLIMRELAY_DUT_%d_FCT", "GND_DMM_%d_EOL", "CAN_H_RES_%d_EOL", "CAN_L_RES_%d_EOL", "L_IND_RES_%d_EOL", "R_IND_RES_%d_EOL", "HB_CONN_DMM_%d_EOL", "14V_RES_%d_EOL", "CAN_L_(DMM-)_%d_EOL", "CAN_H_%d_EOL", "CAN_L_%d_EOL", "14V_%d_EOL", "GND_%d_EOL", "HB_CONN_%d_EOL", "L_IND_%d_EOL", "R_IND_%d_EOL", "CYLINDER_DUT_%d_EOL", "CYL_PB_1_%d_EOL", "CYL_PB_2_%d_EOL", "DUT_PASS_%d_EOL", "DUT_FAIL_%d_EOL", "SPARE1_%d_EOL", "Tower Red_EOL", "Tower Amber_EOL", "Tower Green_EOL", "Tower Buzzer_EOL"] ("Relay_Channel_OUT")
                w226 = T28[] [enum."Tower Red_EOL", enum."Tower Amber_EOL", enum."Tower Green_EOL", enum."Tower Buzzer_EOL"] items=["CONN_SUPPLY_%d_FCT", "HB_CONN_%d_FCT", "L_IND_CONN_%d_FCT", "R_IND_CONN_%d_FCT", "SW1_%d_FCT", "SW2_%d_FCT", "CAN_H_%d_FCT", "CAN_L_%d_FCT", "CYLINDER_ON/OFF_%d_FCT", "SPARE_1_%d_FCT", "SPARE_2_%d_FCT", "Tower Red", "Tower Amber", "Tower Green", "Tower Buzzer", "SLIMRELAY_DUT_%d_FCT", "GND_DMM_%d_EOL", "CAN_H_RES_%d_EOL", "CAN_L_RES_%d_EOL", "L_IND_RES_%d_EOL", "R_IND_RES_%d_EOL", "HB_CONN_DMM_%d_EOL", "14V_RES_%d_EOL", "CAN_L_(DMM-)_%d_EOL", "CAN_H_%d_EOL", "CAN_L_%d_EOL", "14V_%d_EOL", "GND_%d_EOL", "HB_CONN_%d_EOL", "L_IND_%d_EOL", "R_IND_%d_EOL", "CYLINDER_DUT_%d_EOL", "CYL_PB_1_%d_EOL", "CYL_PB_2_%d_EOL", "DUT_PASS_%d_EOL", "DUT_FAIL_%d_EOL", "SPARE1_%d_EOL", "Tower Red_EOL", "Tower Amber_EOL", "Tower Green_EOL", "Tower Buzzer_EOL"] ("Relay_Channel_OUT")
                n68 = Bundle(cluster=T25 {"Message"="", "Message Data"=variant} ("element"), "Message"="Emergency") -> (w231:T25)  [unwired: 1 in]
                n69 = Select(t=w226, s=w227, f=w224) -> (s? t:f=w225:T28[])
                n70 = Enqueue Element At Opposite End(queue=w233, element=w231, error in (no error)=w235) -> (error out=w234:errorcluster)  [unwired: 1 in, 2 out]
                n71 = call "Tower_lamp.vi"("FCT/EOL"=w227, "queue IN"=w228, "DOs"=bool[] [TRUE, FALSE, FALSE, FALSE], "Relay_Channel_OUT"=w225) -> ()  [unwired: 8 in]
              }
            }
          }
          frame "Light Curtain" {
            n72 = case shown="\"ABORTED\", \"Fail\", \"Pass\", \"Starting\"" w240 {
              tunnel: w244 -> [w249 w263]
              tunnel: [w247 w263] -> w243
              tunnel: w242 -> [w246 _]
              tunnel: w241 -> [_ _]
              tunnel: w239 -> [w248 _]
              tunnel: w238 -> [w245 _]
              tunnel: w237 -> [_ _]
              tunnel: w236 -> [_ _]
              frame "ABORTED", "Fail", "Pass", "Starting" {
                n73 = Not Equal?(x=w245, y=w248) -> (x != y?=w250:bool)
                n74 = case shown="True" w250 {
                  tunnel: w249 -> [w251 w255]
                  tunnel: [w251 w254] -> w247
                  tunnel: w246 -> [_ w253]
                  tunnel: w245 -> [_ w252]
                  frame False {
                  }
                  frame True {
                    n75 = case shown="False" w252 {
                      tunnel: w255 -> [w261 w262]
                      tunnel: [w260 w262] -> w254
                      tunnel: w253 -> [w256 _]
                      frame False {
                        n76 = Bundle(cluster=T25 {"Message"="", "Message Data"=variant} ("element"), "Message"="Reset") -> (w257:T25)  [unwired: 1 in]
                        n77 = Enqueue Element At Opposite End(queue=w256, element=w257, error in (no error)=w261) -> (error out=w260:errorcluster)  [unwired: 1 in, 2 out]
                      }
                      frame True {
                      }
                    }
                  }
                }
              }
              frame "Running", Default {
              }
            }
          }
          frame "STOP" {
            n78 = case shown="\"False\", Default" w267 {
              tunnel: w271 -> [w274 w289]
              tunnel: [w273 w288] -> w270
              tunnel: w269 -> [w272 w287]
              tunnel: w268 -> [_ _]
              tunnel: w265 -> [_ w282]
              tunnel: w264 -> [_ w278]
              frame "False", Default {
                n79 = Bundle(cluster=T25 {"Message"="", "Message Data"=variant} ("element"), "Message"="EmergencyReset") -> (w276:T25)  [unwired: 1 in]
                n80 = Enqueue Element At Opposite End(queue=w272, element=w276, error in (no error)=w274) -> (error out=w273:errorcluster)  [unwired: 1 in, 2 out]
              }
              frame "Running", "Starting" {
                w279 = T28[] [enum."Tower Red", enum."Tower Amber", enum."Tower Green", enum."Tower Buzzer"] items=["CONN_SUPPLY_%d_FCT", "HB_CONN_%d_FCT", "L_IND_CONN_%d_FCT", "R_IND_CONN_%d_FCT", "SW1_%d_FCT", "SW2_%d_FCT", "CAN_H_%d_FCT", "CAN_L_%d_FCT", "CYLINDER_ON/OFF_%d_FCT", "SPARE_1_%d_FCT", "SPARE_2_%d_FCT", "Tower Red", "Tower Amber", "Tower Green", "Tower Buzzer", "SLIMRELAY_DUT_%d_FCT", "GND_DMM_%d_EOL", "CAN_H_RES_%d_EOL", "CAN_L_RES_%d_EOL", "L_IND_RES_%d_EOL", "R_IND_RES_%d_EOL", "HB_CONN_DMM_%d_EOL", "14V_RES_%d_EOL", "CAN_L_(DMM-)_%d_EOL", "CAN_H_%d_EOL", "CAN_L_%d_EOL", "14V_%d_EOL", "GND_%d_EOL", "HB_CONN_%d_EOL", "L_IND_%d_EOL", "R_IND_%d_EOL", "CYLINDER_DUT_%d_EOL", "CYL_PB_1_%d_EOL", "CYL_PB_2_%d_EOL", "DUT_PASS_%d_EOL", "DUT_FAIL_%d_EOL", "SPARE1_%d_EOL", "Tower Red_EOL", "Tower Amber_EOL", "Tower Green_EOL", "Tower Buzzer_EOL"] ("Relay_Channel_OUT")
                w280 = T28[] [enum."Tower Red_EOL", enum."Tower Amber_EOL", enum."Tower Green_EOL", enum."Tower Buzzer_EOL"] items=["CONN_SUPPLY_%d_FCT", "HB_CONN_%d_FCT", "L_IND_CONN_%d_FCT", "R_IND_CONN_%d_FCT", "SW1_%d_FCT", "SW2_%d_FCT", "CAN_H_%d_FCT", "CAN_L_%d_FCT", "CYLINDER_ON/OFF_%d_FCT", "SPARE_1_%d_FCT", "SPARE_2_%d_FCT", "Tower Red", "Tower Amber", "Tower Green", "Tower Buzzer", "SLIMRELAY_DUT_%d_FCT", "GND_DMM_%d_EOL", "CAN_H_RES_%d_EOL", "CAN_L_RES_%d_EOL", "L_IND_RES_%d_EOL", "R_IND_RES_%d_EOL", "HB_CONN_DMM_%d_EOL", "14V_RES_%d_EOL", "CAN_L_(DMM-)_%d_EOL", "CAN_H_%d_EOL", "CAN_L_%d_EOL", "14V_%d_EOL", "GND_%d_EOL", "HB_CONN_%d_EOL", "L_IND_%d_EOL", "R_IND_%d_EOL", "CYLINDER_DUT_%d_EOL", "CYL_PB_1_%d_EOL", "CYL_PB_2_%d_EOL", "DUT_PASS_%d_EOL", "DUT_FAIL_%d_EOL", "SPARE1_%d_EOL", "Tower Red_EOL", "Tower Amber_EOL", "Tower Green_EOL", "Tower Buzzer_EOL"] ("Relay_Channel_OUT")
                n81 = Bundle(cluster=T25 {"Message"="", "Message Data"=variant} ("element"), "Message"="EmergencyReset") -> (w285:T25)  [unwired: 1 in]
                n82 = Select(t=w280, s=w278, f=w279) -> (s? t:f=w281:T28[])
                n83 = call "Tower_lamp.vi"("FCT/EOL"=w278, "queue IN"=w282, "DOs"=bool[] [TRUE, FALSE, FALSE, FALSE], "Relay_Channel_OUT"=w281) -> ()  [unwired: 8 in]
                n84 = Enqueue Element At Opposite End(queue=w287, element=w285, error in (no error)=w289) -> (error out=w288:errorcluster)  [unwired: 1 in, 2 out]
              }
            }
          }
          frame Default {
            n85 = case shown="True" w296 {
              selector: w296 -> [w308 w330]
              tunnel: w300 -> [w307 w335]
              tunnel: [w306 w334] -> w299
              tunnel: w298 -> [_ w333]
              tunnel: w297 -> [w301 w332]
              tunnel: w295 -> [_ w331]
              tunnel: [w308 w330] -> w294
              tunnel: w293 -> [w303 w329]
              tunnel: w292 -> [w302 w328]
              tunnel: w291 -> [w305 w327]
              tunnel: w290 -> [w304 w326]
              frame False {
                n86 = case shown="False" w302 {
                  tunnel: w307 -> [w314 w325]
                  tunnel: [w313 w325] -> w306
                  tunnel: w305 -> [w312 _]
                  tunnel: w304 -> [w311 _]
                  tunnel: w303 -> [w310 _]
                  tunnel: w301 -> [w309 _]
                  frame False {
                    n87 = case shown="Default" w309 {
                      tunnel: w314 -> [w319 w324]
                      tunnel: [w318 w324] -> w313
                      tunnel: w312 -> [w317 _]
                      tunnel: w311 -> [w316 _]
                      tunnel: w310 -> [w315 _]
                      frame Default {
                        w321 = T28[] [enum."CYLINDER_ON/OFF_%d_FCT"] items=["CONN_SUPPLY_%d_FCT", "HB_CONN_%d_FCT", "L_IND_CONN_%d_FCT", "R_IND_CONN_%d_FCT", "SW1_%d_FCT", "SW2_%d_FCT", "CAN_H_%d_FCT", "CAN_L_%d_FCT", "CYLINDER_ON/OFF_%d_FCT", "SPARE_1_%d_FCT", "SPARE_2_%d_FCT", "Tower Red", "Tower Amber", "Tower Green", "Tower Buzzer", "SLIMRELAY_DUT_%d_FCT", "GND_DMM_%d_EOL", "CAN_H_RES_%d_EOL", "CAN_L_RES_%d_EOL", "L_IND_RES_%d_EOL", "R_IND_RES_%d_EOL", "HB_CONN_DMM_%d_EOL", "14V_RES_%d_EOL", "CAN_L_(DMM-)_%d_EOL", "CAN_H_%d_EOL", "CAN_L_%d_EOL", "14V_%d_EOL", "GND_%d_EOL", "HB_CONN_%d_EOL", "L_IND_%d_EOL", "R_IND_%d_EOL", "CYLINDER_DUT_%d_EOL", "CYL_PB_1_%d_EOL", "CYL_PB_2_%d_EOL", "DUT_PASS_%d_EOL", "DUT_FAIL_%d_EOL", "SPARE1_%d_EOL", "Tower Red_EOL", "Tower Amber_EOL", "Tower Green_EOL", "Tower Buzzer_EOL"] ("Relay_Channel_Out")
                        w323 = T28[] [enum."CYLINDER_DUT_%d_EOL"] items=["CONN_SUPPLY_%d_FCT", "HB_CONN_%d_FCT", "L_IND_CONN_%d_FCT", "R_IND_CONN_%d_FCT", "SW1_%d_FCT", "SW2_%d_FCT", "CAN_H_%d_FCT", "CAN_L_%d_FCT", "CYLINDER_ON/OFF_%d_FCT", "SPARE_1_%d_FCT", "SPARE_2_%d_FCT", "Tower Red", "Tower Amber", "Tower Green", "Tower Buzzer", "SLIMRELAY_DUT_%d_FCT", "GND_DMM_%d_EOL", "CAN_H_RES_%d_EOL", "CAN_L_RES_%d_EOL", "L_IND_RES_%d_EOL", "R_IND_RES_%d_EOL", "HB_CONN_DMM_%d_EOL", "14V_RES_%d_EOL", "CAN_L_(DMM-)_%d_EOL", "CAN_H_%d_EOL", "CAN_L_%d_EOL", "14V_%d_EOL", "GND_%d_EOL", "HB_CONN_%d_EOL", "L_IND_%d_EOL", "R_IND_%d_EOL", "CYLINDER_DUT_%d_EOL", "CYL_PB_1_%d_EOL", "CYL_PB_2_%d_EOL", "DUT_PASS_%d_EOL", "DUT_FAIL_%d_EOL", "SPARE1_%d_EOL", "Tower Red_EOL", "Tower Amber_EOL", "Tower Green_EOL", "Tower Buzzer_EOL"] ("Relay_Channel_Out")
                        n88 = Select(t=w323, s=w316, f=w321) -> (s? t:f=w322:T28[])
                        n89 = call "Relay_CYL.vi"("DUT"=w315, "EOL/FCT"=w316, "error out"=w319, "DOs"=bool[] [FALSE], "Relay_Channel_Out"=w322, "Relay"=w317) -> ("error out 2"=w318:errorcluster)  [unwired: 5 in]
                      }
                      frame "Running" {
                      }
                    }
                  }
                  frame True {
                  }
                }
              }
              frame True {
                n90 = case shown="\"IDLE..\"" w332 {
                  tunnel: w335 -> [w336 w342]
                  tunnel: [w336 w341] -> w334
                  tunnel: w333 -> [_ _]
                  tunnel: w331 -> [_ _]
                  tunnel: w329 -> [_ w338]
                  tunnel: w328 -> [_ w337]
                  tunnel: w327 -> [_ w340]
                  tunnel: w326 -> [_ w339]
                  frame "Running", Default {
                  }
                  frame "IDLE.." {
                    n91 = case shown="False" w337 {
                      tunnel: w342 -> [w347 w352]
                      tunnel: [w346 w352] -> w341
                      tunnel: w340 -> [w345 _]
                      tunnel: w339 -> [w344 _]
                      tunnel: w338 -> [w343 _]
                      frame False {
                        w349 = T28[] [enum."Tower Amber"] items=["CONN_SUPPLY_%d_FCT", "HB_CONN_%d_FCT", "L_IND_CONN_%d_FCT", "R_IND_CONN_%d_FCT", "SW1_%d_FCT", "SW2_%d_FCT", "CAN_H_%d_FCT", "CAN_L_%d_FCT", "CYLINDER_ON/OFF_%d_FCT", "SPARE_1_%d_FCT", "SPARE_2_%d_FCT", "Tower Red", "Tower Amber", "Tower Green", "Tower Buzzer", "SLIMRELAY_DUT_%d_FCT", "GND_DMM_%d_EOL", "CAN_H_RES_%d_EOL", "CAN_L_RES_%d_EOL", "L_IND_RES_%d_EOL", "R_IND_RES_%d_EOL", "HB_CONN_DMM_%d_EOL", "14V_RES_%d_EOL", "CAN_L_(DMM-)_%d_EOL", "CAN_H_%d_EOL", "CAN_L_%d_EOL", "14V_%d_EOL", "GND_%d_EOL", "HB_CONN_%d_EOL", "L_IND_%d_EOL", "R_IND_%d_EOL", "CYLINDER_DUT_%d_EOL", "CYL_PB_1_%d_EOL", "CYL_PB_2_%d_EOL", "DUT_PASS_%d_EOL", "DUT_FAIL_%d_EOL", "SPARE1_%d_EOL", "Tower Red_EOL", "Tower Amber_EOL", "Tower Green_EOL", "Tower Buzzer_EOL"] ("Relay_Channel_Out")
                        w351 = T28[] [enum."Tower Amber_EOL"] items=["CONN_SUPPLY_%d_FCT", "HB_CONN_%d_FCT", "L_IND_CONN_%d_FCT", "R_IND_CONN_%d_FCT", "SW1_%d_FCT", "SW2_%d_FCT", "CAN_H_%d_FCT", "CAN_L_%d_FCT", "CYLINDER_ON/OFF_%d_FCT", "SPARE_1_%d_FCT", "SPARE_2_%d_FCT", "Tower Red", "Tower Amber", "Tower Green", "Tower Buzzer", "SLIMRELAY_DUT_%d_FCT", "GND_DMM_%d_EOL", "CAN_H_RES_%d_EOL", "CAN_L_RES_%d_EOL", "L_IND_RES_%d_EOL", "R_IND_RES_%d_EOL", "HB_CONN_DMM_%d_EOL", "14V_RES_%d_EOL", "CAN_L_(DMM-)_%d_EOL", "CAN_H_%d_EOL", "CAN_L_%d_EOL", "14V_%d_EOL", "GND_%d_EOL", "HB_CONN_%d_EOL", "L_IND_%d_EOL", "R_IND_%d_EOL", "CYLINDER_DUT_%d_EOL", "CYL_PB_1_%d_EOL", "CYL_PB_2_%d_EOL", "DUT_PASS_%d_EOL", "DUT_FAIL_%d_EOL", "SPARE1_%d_EOL", "Tower Red_EOL", "Tower Amber_EOL", "Tower Green_EOL", "Tower Buzzer_EOL"] ("Relay_Channel_Out")
                        n92 = Select(t=w351, s=w344, f=w349) -> (s? t:f=w350:T28[])
                        n93 = call "Relay_CYL.vi"("DUT"=w343, "EOL/FCT"=w344, "error out"=w347, "DOs"=bool[] [TRUE], "Relay_Channel_Out"=w350, "Relay"=w345) -> ("error out 2"=w346:errorcluster)  [unwired: 5 in]
                      }
                      frame True {
                      }
                    }
                  }
                }
              }
            }
          }
        }
        n94 = disable-structure shown="Enabled" {
          frame Disabled {
            n95 = control-ref of="STATUS"() -> (w102:refnum<vi>)
            n96 = property class="Bool (strict)"(reference=w102, "BoolText.Text"="Starting" ("Boolean Text.Text")) -> ()  [unwired: 1 in, 2 out]
          }
          frame Enabled {
          }
        }
        n97 = Bundle(cluster=T25 {"Message"="", "Message Data"=variant} ("element"), "Message"="Poll") -> (w81:T25)  [unwired: 1 in]
        n98 = Enqueue Element(queue=w84, element=w81, error in (no error)=w89) -> (queue out=w83:refnum<queue>, error out=w85:errorcluster)  [unwired: 1 in, 1 out]
      }
      frame "Exit" {
        n99 = Release Queue(queue=w384, error in (no error)=w386) -> (error out=w385:errorcluster)  [unwired: 1 in, 2 out]
      }
      frame "Initialize" {
        n100 = Variant To Data(error in=w395, type=FALSE, Variant=w389) -> (data=w388:bool, error out=w391:errorcluster)
        n101 = case shown="True" w388 {
          tunnel: w391 -> [w396 w403]
          tunnel: [w396 w402] -> w394
          tunnel: w393 -> [w397 w401]
          tunnel: [w397 w400] -> w392
          frame False {
          }
          frame True {
            n102 = flat-sequence {
              tunnel: w403 -> [w407]
              tunnel: w401 -> [w405]
              tunnel: [w406] -> w399
              tunnel: [w404] -> w398
              tunnel: [w412] -> w400
              tunnel: [w413] -> w402
              tunnel: w399 -> [w413]
              tunnel: w398 -> [w412]
              frame #0 {
                n103 = Bundle By Name(cluster=T25 {"Message"="", "Message Data"=variant} ("element"), "Message"="Poll") -> (w410:T25)
                n104 = Enqueue Element At Opposite End(queue=w405, element=w410, error in (no error)=w407) -> (queue out=w404:refnum<queue>, error out=w406:errorcluster)  [unwired: 1 in, 1 out]
              }
              frame #1 {
                n105 = Wait (ms)(milliseconds to wait=u32 2000) -> ()  [unwired: 1 out]
              }
            }
          }
        }
      }
    }
    n106 = call <vilib>:"Clear Errors.vi"("error in (no error)"=w55) -> ("error out"=w50:errorcluster)  [unwired: 5 in, 1 out]
  }
  n107 = while {
    shift-right: [w418] -> w25
    shift-left: w22 -> [w419]
    tunnel: [w415] -> w23
    tunnel: w6 -> [w414]
    stop <- w417 stop-if-true
    # "Event Handling Loop"
    n108 = event shown="[2] \"Abort\": Value Change" {
      selector: w419 -> [_ _ _ _ _ _ _]
      dyn-events: [_ _ _ _ _ _ _] -> w418
      timeout: _ -> [_ _ _ _ _ _ _]
      tunnel: [_ _ _ _ _ _ TRUE ("Discard?")] -> w417
      tunnel: [w422 w429 w432 w438 _ w443 _] -> w416
      tunnel: w414 -> [w420 w428 w431 w435 _ w440 _]
      event "Start Button": Value Change {
        n109 = event-data() -> ()  [unwired: 1 in, 1 out]
        n110 = call "Test_Enque_Message_FGV.vi"("Priority"=TRUE ("Priority Message? (F)"), "Message"="StartTest", "queue in"=w420) -> ("error out"=w422:errorcluster)  [unwired: 8 in]
      }
      event "PP": Value Change {
        n111 = event-data() -> ("NewVal"=w426:bool)  [unwired: 1 in]
        n112 = Select(t="CheckDUT", s=w426, f="Reset" ("Message")) -> (s? t:f=w425:string)
        n113 = call "Test_Enque_Message_FGV.vi"("Priority"=TRUE ("Priority Message? (F)"), "Message"=w425, "queue in"=w428) -> ("error out"=w429:errorcluster)  [unwired: 8 in]
      }
      event "Abort": Value Change {
        n114 = event-data() -> ()  [unwired: 1 in, 1 out]
        n115 = call "Test_Enque_Message_FGV.vi"("Priority"=TRUE ("Priority Message? (F)"), "Message"="EmergencyReset", "queue in"=w431) -> ("error out"=w432:errorcluster)  [unwired: 8 in]
      }
      event Panel Close? {
        n116 = event-data() -> ()  [unwired: 1 in, 1 out]
        n117 = call "Test_Enque_Message_FGV.vi"("Priority"=TRUE ("Priority Message? (F)"), "Message"="Confirm Quit", "queue in"=w435) -> ("error out"=w438:errorcluster)  [unwired: 8 in]
        n118 = event-data("Discard?"=TRUE) -> ()  [unwired: 1 in, 1 out]
      }
      event Application Instance Close {
        n119 = event-data() -> ()  [unwired: 1 in, 1 out]
      }
      event "Exit": Value Change {
        n120 = event-data() -> ()  [unwired: 1 in, 1 out]
        n121 = call "Test_Enque_Message_FGV.vi"("Priority"=TRUE ("Priority Message? (F)"), "Message"="Confirm Quit", "queue in"=w440) -> ("error out"=w443:errorcluster)  [unwired: 8 in]
      }
      event User Event {
        (unwired) "\"Exit\" button pressed" ("VI Stopped")
        n122 = event-data() -> ()  [unwired: 1 in, 1 out]
      }
    }
    n123 = call "Test_Error_Handler_EHL_FGV.vi"("error in (no error)"=w416, "queue in"=w414) -> ("error Out"=w415:errorcluster)  [unwired: 9 in]
  }
  n124 = while {
    tunnel: w4 -> [w445]
    shift-right: [w456] -> _
    shift-left: w9 -> [w457]
    tunnel: w11 -> [w454]
    tunnel: w5 -> [w453]
    tunnel: [w448] -> w29
    tunnel: w2 -> [w447]
    tunnel: w6 -> [w446]
    stop <- w455 stop-if-true
    # "Message Handling Loop FGV"
    n125 = disable-structure shown="Enabled" {
      disable-tunnel: w453 -> [w461 w467]
      disable-tunnel: [w460 w465] -> w452
      disable-tunnel: [w459 w462] -> w451
      disable-tunnel: [w458 w463] -> w450
      disable-tunnel: w446 -> [_ w466]
      frame Disabled {
        n126 = call "Test_Dequeue_Message_FGV.vi"("error in (no error)"=w461) -> ("error out"=w460:errorcluster, "Message Data"=w459:variant, "Message"=w458:string)  [unwired: 8 in]
      }
      frame Enabled {
        n127 = Dequeue Element(queue=w466, error in (no error)=w467) -> (element=w464:T25, error out=w465:errorcluster)  [unwired: 1 in, 2 out]
        n128 = Unbundle(w464) -> ("Message"=w463:string, "Message Data"=w462:variant)
      }
    }
    n129 = case "Message Cases" shown="\"GetData\"" w450 {
      selector: w450 -> [_ _ _ _ _ _ _ _ _ _ _ _ _ _ _ _ _ _ _ _ _ _ _ _ _ _ _ _ _ _ w3345]
      tunnel: w452 -> [w491 w502 w532 w589 w610 w663 w723 w760 w764 w796 w834 w850 w963 w998 w1043 w1610 w1645 w2443 w2932 w2977 w2994 w3126 w3156 w3169 w3209 w3258 w3287 w3305 w3321 w3334 _]
      tunnel: [w492 w519 w550 w588 w624 w666 w727 w759 w766 w814 w842 w849 w970 w998 w1042 w1609 w1636 w2440 w2924 w2979 w2993 w3053 w3155 w3175 w3219 w3267 w3288 w3300 w3323 w3331 w3346] -> w449
      tunnel: w457 -> [w493 w513 w561 w587 w627 w680 w728 w758 w762 w805 w844 w857 w977 w1002 w1040 w1608 w1627 w2437 w2931 w2973 w3014 w3071 w3154 w3167 w3202 w3249 w3286 w3295 w3311 w3332 w3347]
      tunnel: [w488 w508 w555 w587 w625 w667 w728 w753 w765 w811 w841 w856 w975 w999 w1039 w1608 w1635 w2436 w2926 w2981 w2999 w3071 w3154 w3173 w3206 w3255 w3286 w3291 w3311 w3332 w3347] -> w456
      tunnel: [_ _ _ _ _ _ _ _ _ _ _ _ _ _ _ _ _ _ _ _ _ _ _ _ _ _ _ _ _ TRUE _] -> w455
      tunnel: w451 -> [_ _ _ _ _ _ _ _ _ _ _ _ _ _ _ _ _ _ _ _ _ _ _ _ _ _ _ w3304 _ _ _]
      tunnel: w454 -> [_ _ _ _ _ _ _ _ _ _ _ _ _ _ _ _ _ _ _ _ _ _ _ _ _ _ _ _ _ _ _]
      tunnel: w447 -> [_ _ _ _ _ _ _ _ _ _ _ _ _ _ _ _ _ _ _ _ _ _ _ _ _ _ _ _ _ w3337 _]
      tunnel: w446 -> [w469 w518 w534 w590 w623 w670 _ _ _ w803 w837 w848 w960 w995 _ _ w1630 w2435 w2911 _ _ _ _ w3176 w3204 w3252 _ _ w3318 w3335 _]
      tunnel: w445 -> [w471 _ _ _ _ _ _ _ _ _ _ _ _ _ _ _ _ _ _ _ _ _ _ _ _ _ _ _ _ _ _]
      frame "Initialize" {
        # "Initialize"
        n130 = call "Specify_Path.vi"("Path_Enum"=enum16{"Find_Path", "Get_Path"}."Get_Path", "error in (no error)"=w491) -> ("Configurations"=w475:path, "DATA"=w473:path, "Settings"=w486:path, "error out"=w477:errorcluster)  [unwired: 6 in, 4 out]
        n131 = Build Path(base path=w475, name or relative path="PMC.ini") -> (appended path=w482:path)
        n132 = call "INI_driver.vi"("Enum"=T29."All_values", "instrument file path"=w482, "error in (no error)"=w477, "Section"="PMC_Info") -> ("error out"=w476:errorcluster, "Values out"=w480:string[])  [unwired: 4 in, 2 out]
        n133 = Index Array(array=w480) -> (element=w479:string)  [unwired: 1 in]
        n134 = String To Path(string=w479) -> (path=w474:path)
        n135 = Bundle By Name(cluster=w493, "Settings"=w486, "PMC path"=w474, "Table"=string[][] [], "Filename"="", "Configuration path"=w475, "InitPro"=TRUE, "Data Path"=w473, "Test2_Q"=w469, "Relay_Module_Q"=w471, "Barcode Scanned?"=FALSE) -> (w488:T2)
        n136 = local write "Test Started?"(FALSE ("Test Started?")) -> ()
        n137 = for {
          N: 200 -> [_]
          i -> [w495]
          n138 = control-ref of="Table"() -> (w494:refnum<vi>)
          n139 = Bundle By Name(cluster=T30 {"Row"=0, "Column"=0} ("Active Cell:Active Cell"), "Row"=w495, "Column"=5) -> (w500:T30)
          n140 = property class="Tbl (strict)"(reference=w494, "Active Cell"=w500) -> (reference out=w497:refnum<vi>)  [unwired: 1 in, 1 out]
          n141 = property class="Tbl (strict)"(reference=w497, "Cell BG Color"=u32 16448250 ("Active Cell:Cell Background Color")) -> ()  [unwired: 1 in, 2 out]
        }
        n142 = call "Test_Enque_Message_FGV.vi"("error in (no error)"=w476, "Message"="SelectConfig", "queue in"=w469) -> ("error out"=w492:errorcluster)  [unwired: 8 in]
      }
      frame "SelectConfig" {
        n143 = Unbundle By Name(w513) -> ("Configuration path"=w509:path, "Settings"=w510:path, "config"=w501:string)
        "Configs" <- w501
        n144 = Concatenate Strings(w501, ".bin" ("string")) -> (w512:string)
        n145 = Concatenate Strings(w501, "-Combined" ("string"), ".ini" ("string")) -> (w511:string)
        n146 = Build Path(base path=w510, name or relative path=w512) -> (appended path=w506:path)
        n147 = Build Path(base path=w509, name or relative path=w511) -> (appended path=w507:path)
        n148 = Bundle By Name(cluster=w513, "EQUIP Config path"=w507, "Settings"=w506, "config"=w501, "Filename"=w501) -> (w508:T2)
        n149 = Select(t="Confirm Quit", s=FALSE, f="ReadConfig" ("Message")) -> (s? t:f=w515:string)
        n150 = call "Test_Enque_Message_FGV.vi"("Priority"=TRUE, "error in (no error)"=w502, "Message"=w515, "queue in"=w518) -> ("error out"=w519:errorcluster)  [unwired: 7 in]
      }
      frame "ReadConfig" {
        w539 = 1.0 ("Increment")
        w541 = 0.0 ("Minimum")
        w547 = string[] ["ScriptName", "Stepname", "LSL", "ACTUAL", "USL", "RESULT", "UNIT"] ("Column Header Strings[]")
        n151 = Unbundle By Name(w561) -> ("EQUIP Config path"=w531:path, "Settings"=w559:path)
        n152 = call "BIN_File.vi"("Enum"=enum16{"Read", "Write"}."Read", "error in"=w532, "Path"=w559) -> ("error out"=w560:errorcluster, "data out"=w557:string)  [unwired: 7 in]
        n153 = call "INI_driver.vi"("Enum"=T29."All_sections", "instrument file path"=w531, "error in (no error)"=w532) -> ("error out"=w530:errorcluster, "section names"=w527:string[])  [unwired: 5 in, 2 out]
        n154 = Unflatten From String(type=T3 {"Script_Tree"=refnum, "Scripts"=[], "ScriptDetails"={"Script Name"="", "Steps"=[]}, "Current Step"={"StepName"="", "StepDetails"="", "Type"=enum."RELAY_CHANNEL_WRITE"}, "ScriptName"="", "StepName"="", "Children Symbols"=[], "Parrent Symbol"=[], "Configurations:"="", "Config"="", "Scriptno."=0, "PS_Write"={"Set_parameter"=0, "VOLTAGE"="", "CURRENT"="", "OUTPUT"=FALSE, "Delay"=FALSE, "Delay time"=0.0}, "DMM_CONFIG"={"CONFIG PARAMETER"=0, "AUTO RANGE"=FALSE, "RANGE"="", "Delay"=FALSE, "Delay time"=0.0}, "READ_DATAS"={"EQUIPMENT"=0, "PARAMETER"=0, "LSL"=0.0, "USL"=0.0, "RESULT"="", "UNIT"="", "Delay"=FALSE, "Delay time"=0.0}, "Set_Channel_Relay"={"Relay_CH_Array"=[]}, "DAQ_Config"={"AUTO RANGE"=FALSE, "CHANNEL LIST"="", "SELECT Card"=0, "SELECT SLOT"=0, "Function"=0}, "CAN_MSGs_Write"={"Scaling Factor"=0, "Physical value"=0.0, "CAN_Frames"={"CAN_ID"=0, "MSGTYPE"=0, "Payload"=[], "Length"=0}, "Offset value"=0.0, "Framing datas"=[], "CAN_Frame Enable"=FALSE, "Add Signal"=FALSE, "Delete Signal"=FALSE, "Signal Values"=[], "Time(ms)"=0.0, "Repetition"=FALSE, "Delay"=FALSE, "Delay time"=0.0}, "CAN_Read"={"Database"="", "Signal"="", "BYTES"=[], "ReadPayload"=[], "String_Data"="", "ReadValue"=0.0, "CANID"=0, "SERVICE ID"=0, "SUB-SERVICE ID"=0, "DELAY "=FALSE, "Delay time(ms)"=0.0}, "Camera"={"Trigger"=FALSE, "Prog No."="", "Delay"=FALSE, "Delay time"=0.0, "Storage"="", "Col no."="", "Row no."=""}, "Tab Control"=refnum, "MCU Flashing"={"Result Path"=path "", "Result"=""}, "Noeway_Flashing"={"Neoway_Firmware"=path "", "RESULT STRING"="", "Delay"=FALSE, "Delay time"=0.0}, "SSL"={"SSL_EXE"=path "", "RESULT STRING"="", "Delay"=FALSE, "Delay time"=0.0}} ("UI Data"), binary string=w557, error in (no error)=w560) -> (value=w554:T3, error out=w537:errorcluster)  [unwired: 2 in, 1 out]
        n155 = for {
          tunnel: w531 -> [w572]
          tunnel: w530 -> [w571]
          tunnel: [w569] -> w528
          tunnel: w527 -> [w567] mode=indexing
          tunnel: [w566] -> w526 mode=indexing
          n156 = call "INI_driver.vi"("Enum"=T29."Read", "instrument file path"=w572, "error in (no error)"=w571, "Section"=w567, "Key_name"=string[] ["Equip_name"]) -> ("error out"=w569:errorcluster, "Values out"=w566:string[])  [unwired: 3 in, 2 out]
        }
        n157 = Unbundle By Name(w554) -> ("Parrent Symbol"=w522:i32[], "Scripts"=w523:T4[])
        n158 = property on="Start Button" class="Bool"(error in=w537, "DisabledEnum"=T31."Enabled" ("Disabled")) -> (error out=w536:errorcluster)  [unwired: 1 in, 1 out]
        n159 = Index Array(array=w526, index (col)=0 ("disabled index (col)")) -> (element=w524:string[])  [unwired: 1 in]
        n160 = Merge Errors(w528, w536) -> (w529:errorcluster)
        n161 = for {
          tunnel: w523 -> [w563] mode=indexing
          tunnel: w522 -> [w565] mode=indexing
          tunnel: [w563] -> w521 mode=indexing if=w562
          n162 = Equal?(x=w565, y=40) -> (x = y?=w562:bool)
        }
        n163 = Array Size(array=w521) -> (size(s)=w553:i32)
        n164 = To Unsigned Quad Integer(1:w553) -> (0:w540:u64)
        n165 = Bundle By Name(cluster=T33 {"Minimum"=0.0, "Maximum"=0.0, "Increment"=0.0} ("Data Entry Limits"), "Minimum"=w541, "Maximum"=w540, "Increment"=w539) -> (w545:T33)
        n166 = Bundle By Name(cluster=T32 {"Minimum"=0.0, "Maximum"=0.0, "Increment"=0.0, "Minor Increment"=0.0, "Start"=0.0} ("Scale.Range"), "Minimum"=w541, "Maximum"=w540, "Increment"=w539, "Minor Increment"=w539, "Start"=0.0) -> (w542:T32)
        n167 = control-ref of="Test Progress..."() -> (w546:refnum<vi>)
        n168 = property class="Slide (strict)"(reference=w546, "Data Range"=w545, "Scale.Range"=w542) -> ()  [unwired: 1 in, 2 out]
        n169 = Bundle By Name(cluster=w561, "Selected_Scripts"=w521, "EQUP LIST"=w524, "Scriptno."=u64 0, "TotalScripts"=w540, "UI Data"=w554, "Header data"=w547) -> (w555:T2)
        n170 = property on="Table" class="Tbl (strict)"(error in=w529, "Column Headers[]"=w547, "Col Headers Vis"=TRUE ("Visible Items:Column Headers Visible")) -> (error out=w549:errorcluster)  [unwired: 1 in, 1 out]
        n171 = call "Test_Enque_Message_FGV.vi"("error in (no error)"=w549, "Message"="Init_Q", "queue in"=w534) -> ("error out"=w550:errorcluster)  [unwired: 8 in]
      }
      frame "Launch_Drivers" {
        (unwired) "Init_Q" ("Message")
        (unwired) FALSE
        n172 = local read "EOL/FCT"() -> (w576:bool)
        n173 = Unbundle By Name(w587) -> ("EQUP LIST"=w575:string[], "DUT"=w584:i32, "config"=w579:string)
        n174 = case shown="True" w576 {
          tunnel: w575 -> [w593 w594]
          tunnel: string[] ["MCU_Flashing", "Noeway_Flashing"] -> [w592 _]
          tunnel: [w591 w594] -> w573
          frame False {
            n175 = Build Array (concatenate)(w593, w592) -> (w591:string[])
          }
          frame True {
          }
        }
        n176 = Number To Decimal String(number=w584) -> (decimal integer string=w577:string)  [unwired: 1 in]
        n177 = call "DY_VI_ref.vi"("EQUIP LIST"=w573) -> ("VI_ref"=w585:refnum<vi>[])
        n178 = for {
          shift-right: [w606] -> w586
          shift-left: w589 -> [w607]
          tunnel: w585 -> [w604] mode=indexing
          tunnel: [w603] -> w583 mode=indexing
          tunnel: w577 -> [w596]
          shift-right: [w597] -> _
          shift-left: w579 -> [w597]
          n179 = To Variant(anything=w596) -> (Variant=w601:variant)
          n180 = To Variant(anything=w597) -> (Variant=w598:variant)
          n181 = Build Array(w601, w598) -> (w600:variant[])
          n182 = call "Dynamic launcher.vi"("element"=string[] ["DUT", "Config"], "Clone ?"=TRUE, "Value"=w600, "VI Refnum"=w604, "error in (no error)"=w607, "Open FP"=FALSE, "options"=8) -> ("Failed"=w603:bool, "error out"=w606:errorcluster)  [unwired: 6 in, 1 out]
        }
        n183 = And Array Elements(Boolean array=w583) -> (logical AND=w578:bool)
        n184 = Select(t="Confirm Quit", s=w578, f="Init_N" ("Message")) -> (s? t:f=w580:string)
        n185 = call "Test_Enque_Message_FGV.vi"("error in (no error)"=w586, "Message"=w580, "queue in"=w590) -> ("error out"=w588:errorcluster)  [unwired: 8 in]
      }
      frame "Init_Q" {
        (unwired) "Init_N" ("Message")
        (unwired) string[] ["<Select>", "MP711134-14V", "MP711134-12V", "Keysight34461a", "DMM6500", "PCAN", "Relay_Module", "GNSS", "Bluetooth", "Noeway_Flashing", "MCU_Flashing"] ("Strings []")
        # "Initialize Q"
        n186 = Unbundle By Name(w627) -> ("Relay_Module_Q"=w615:refnum<queue>, "EQUP LIST"=w612:string[], "DUT"=w626:i32, "config"=w621:string)
        n187 = Match Pattern(string=w621, regular expression="EOL") -> (offset past match=w619:i32)  [unwired: 1 in, 3 out]
        n188 = Number To Decimal String(number=w626) -> (decimal integer string=w608:string)  [unwired: 1 in]
        n189 = Greater Than 0?(x=w619) -> (x > 0?=w613:bool)
        "EOL/FCT" <- w613
        n190 = for {
          shift-right: [w656] -> w614
          shift-left: w610 -> [w657]
          tunnel: w608 -> [w654]
          tunnel: w612 -> [w652] mode=indexing
          tunnel: [w651] -> w611 mode=indexing
          n191 = Concatenate Strings(w652, w654) -> (w653:string)
          n192 = Obtain Queue(name (unnamed)=w653, element data type=T25 {"Message"="", "Message Data"=variant} ("element"), error in (no error)=w657) -> (queue out=w651:refnum<queue>, error out=w656:errorcluster)  [unwired: 2 in, 1 out]
        }
        n193 = Search 1D Array(1D array=w612, element="Relay_Module") -> (index of element=w617:i32)  [unwired: 1 in]
        n194 = case shown="True" w613 {
          tunnel: w611 -> [w631 w643]
          tunnel: w610 -> [w633 w645]
          tunnel: [w629 w641] -> w609
          tunnel: w608 -> [w628 _]
          frame False {
            n195 = for {
              shift-right: [w639] -> _
              shift-left: w633 -> [w640]
              tunnel: string[] ["MCU_Flashing", "Noeway_Flashing"] -> [w637] mode=indexing
              tunnel: [w636] -> w630 mode=indexing
              tunnel: w628 -> [w634]
              n196 = Concatenate Strings(w637, w634) -> (w635:string)
              n197 = Obtain Queue(name (unnamed)=w635, element data type=T25 {"Message"="", "Message Data"=variant} ("element"), error in (no error)=w640) -> (queue out=w636:refnum<queue>, error out=w639:errorcluster)  [unwired: 2 in, 1 out]
            }
            n198 = Build Array (concatenate)(w631, w630) -> (w629:refnum<queue>[])
          }
          frame True {
            n199 = for {
              shift-right: [w649] -> _
              shift-left: w645 -> [w650]
              tunnel: string[] ["Keyence_VS150"] -> [w647] mode=indexing
              tunnel: [w646] -> w642 mode=indexing
              n200 = Obtain Queue(name (unnamed)=w647, element data type=T25 {"Message"="", "Message Data"=variant} ("element"), error in (no error)=w650) -> (queue out=w646:refnum<queue>, error out=w649:errorcluster)  [unwired: 2 in, 1 out]
            }
            n201 = Build Array (concatenate)(w643, w642) -> (w641:refnum<queue>[])
          }
        }
        n202 = Index Array(array=w609, index=w617) -> (element=→"Relay":refnum<queue>)
        n203 = Bundle By Name(cluster=w627, "EQUP LIST"=w612, "Relay_Module_Q"=w615, "Array_Q"=w609) -> (w625:T2)
        n204 = call "Test_Enque_Message_FGV.vi"("error in (no error)"=w614, "Message"="Launch_Drivers", "queue in"=w623) -> ("error out"=w624:errorcluster)  [unwired: 8 in]
      }
      frame "Init_N" {
        n205 = control-ref of="STATUS"() -> (w678:refnum<vi>)
        n206 = Unbundle By Name(w680) -> ("DUT"=w662:i32, "EQUP LIST"=w668:string[])
        n207 = property class="Bool (strict)"(reference=w678, "Colors [4]"=cluster{u32, u32}[] [{13816530, 13816530}], "BoolText.Text"="IDLE.." ("Boolean Text.Text")) -> ()  [unwired: 1 in, 2 out]
        n208 = for {
          shift-right: [w719] -> w658
          shift-left: w663 -> [w720]
          tunnel: w668 -> [w713] mode=indexing
          tunnel: w662 -> [w718]
          tunnel: [w715] -> w665 mode=indexing
          n209 = Number To Decimal String(number=w718) -> (decimal integer string=w716:string)  [unwired: 1 in]
          n210 = Concatenate Strings(w713, "_N" ("string"), w716) -> (w717:string)
          n211 = Obtain Notifier(name (unnamed)=w717, notification data type=T25 {"Message"="", "Message Data"=variant} ("notification"), error in (no error)=w720) -> (notifier out=w715:refnum<notifier>, error out=w719:errorcluster)  [unwired: 1 in, 1 out]
        }
        n212 = Number To Decimal String(number=w662) -> (decimal integer string=w661:string)  [unwired: 1 in]
        n213 = local read "EOL/FCT"() -> (w659:bool)
        n214 = case shown="False" w659 {
          tunnel: w665 -> [w685 w698]
          tunnel: w663 -> [w687 w700]
          tunnel: [w683 w696] -> w664
          tunnel: w661 -> [w682 _]
          tunnel: [w681 w695] -> w660
          frame False {
            n215 = for {
              shift-right: [w693] -> w681
              shift-left: w687 -> [w694]
              tunnel: string[] ["MCU_Flashing_N", "Noeway_Flashing_N"] -> [w691] mode=indexing
              tunnel: [w690] -> w684 mode=indexing
              tunnel: w682 -> [w688]
              n216 = Concatenate Strings(w691, w688) -> (w689:string)
              n217 = Obtain Notifier(name (unnamed)=w689, notification data type=T25 {"Message"="", "Message Data"=variant} ("element"), error in (no error)=w694) -> (notifier out=w690:refnum<notifier>, error out=w693:errorcluster)  [unwired: 1 in, 1 out]
            }
            n218 = Build Array (concatenate)(w685, w684) -> (w683:refnum<notifier>[])
          }
          frame True {
            n219 = for {
              shift-right: [w704] -> w695
              shift-left: w700 -> [w705]
              tunnel: string[] ["Keyence_VS150"] -> [w702] mode=indexing
              tunnel: [w701] -> w697 mode=indexing
              n220 = Obtain Notifier(name (unnamed)=w702, notification data type=T25 {"Message"="", "Message Data"=variant} ("element"), error in (no error)=w705) -> (notifier out=w701:refnum<notifier>, error out=w704:errorcluster)  [unwired: 1 in, 1 out]
            }
            n221 = Build Array (concatenate)(w698, w697) -> (w696:refnum<notifier>[])
          }
        }
        n222 = Merge Errors(w660, w658) -> (w669:errorcluster)
        n223 = Bundle By Name(cluster=w680, "Array_N"=w664) -> (w667:T2)
        n224 = property on="Abort" class="Bool"(error in=w669, "DisabledEnum"=T31."Disabled and Grayed Out" ("Disabled")) -> (error out=w672:errorcluster)  [unwired: 1 in, 1 out]
        n225 = disable-structure shown="Enabled" {
          disable-tunnel: [w709 w711] -> w675
          disable-tunnel: [w707 w710] -> w674
          disable-tunnel: w672 -> [w706 w711]
          disable-tunnel: w670 -> [_ w710]
          frame Disabled {
            n226 = call "Test_Queue_Comm_FGV.vi"("error in (no error)"=w706, "Enum"=Test_FGV_Queue_Control."Get") -> ("error Out"=w709:errorcluster, "queue Out"=w707:refnum<queue>)  [unwired: 8 in]
          }
          frame Enabled {
          }
        }
        n227 = call "Test_Enqueue Message (Array).vi"("error in (no error)"=w675, "Message Array"=string[] ["Update Display", "init_condition", "Product_CNT"] ("f"), "Message Queue"=w674) -> ("error out"=w671:errorcluster)  [unwired: 7 in, 1 out]
        n228 = Merge Errors(w671) -> (w666:errorcluster)
      }
      frame "init_condition" {
        n229 = Unbundle By Name(w728) -> ("Relay_Module_Q"=w730:refnum<queue>, "DUT"=w721:i32)
        n230 = flat-sequence {
          tunnel: w723 -> [w742]
          tunnel: [w742] -> w725
          tunnel: [w736] -> w724
          tunnel: w721 -> [w734]
          tunnel: [w744] -> _
          tunnel: [w745] -> w722
          tunnel: w725 -> [w745]
          tunnel: w724 -> [w744]
          frame #0 {
            w737 = T28[] [enum."Tower Amber", enum."Tower Red", enum."Tower Green", enum."Tower Buzzer", enum."CYLINDER_ON/OFF_%d_FCT"] items=["CONN_SUPPLY_%d_FCT", "HB_CONN_%d_FCT", "L_IND_CONN_%d_FCT", "R_IND_CONN_%d_FCT", "SW1_%d_FCT", "SW2_%d_FCT", "CAN_H_%d_FCT", "CAN_L_%d_FCT", "CYLINDER_ON/OFF_%d_FCT", "SPARE_1_%d_FCT", "SPARE_2_%d_FCT", "Tower Red", "Tower Amber", "Tower Green", "Tower Buzzer", "SLIMRELAY_DUT_%d_FCT", "GND_DMM_%d_EOL", "CAN_H_RES_%d_EOL", "CAN_L_RES_%d_EOL", "L_IND_RES_%d_EOL", "R_IND_RES_%d_EOL", "HB_CONN_DMM_%d_EOL", "14V_RES_%d_EOL", "CAN_L_(DMM-)_%d_EOL", "CAN_H_%d_EOL", "CAN_L_%d_EOL", "14V_%d_EOL", "GND_%d_EOL", "HB_CONN_%d_EOL", "L_IND_%d_EOL", "R_IND_%d_EOL", "CYLINDER_DUT_%d_EOL", "CYL_PB_1_%d_EOL", "CYL_PB_2_%d_EOL", "DUT_PASS_%d_EOL", "DUT_FAIL_%d_EOL", "SPARE1_%d_EOL", "Tower Red_EOL", "Tower Amber_EOL", "Tower Green_EOL", "Tower Buzzer_EOL"] ("f")
            w738 = T28[] [enum."Tower Amber_EOL", enum."Tower Red_EOL", enum."Tower Green_EOL", enum."Tower Buzzer_EOL", enum."CYLINDER_DUT_%d_EOL"] items=["CONN_SUPPLY_%d_FCT", "HB_CONN_%d_FCT", "L_IND_CONN_%d_FCT", "R_IND_CONN_%d_FCT", "SW1_%d_FCT", "SW2_%d_FCT", "CAN_H_%d_FCT", "CAN_L_%d_FCT", "CYLINDER_ON/OFF_%d_FCT", "SPARE_1_%d_FCT", "SPARE_2_%d_FCT", "Tower Red", "Tower Amber", "Tower Green", "Tower Buzzer", "SLIMRELAY_DUT_%d_FCT", "GND_DMM_%d_EOL", "CAN_H_RES_%d_EOL", "CAN_L_RES_%d_EOL", "L_IND_RES_%d_EOL", "R_IND_RES_%d_EOL", "HB_CONN_DMM_%d_EOL", "14V_RES_%d_EOL", "CAN_L_(DMM-)_%d_EOL", "CAN_H_%d_EOL", "CAN_L_%d_EOL", "14V_%d_EOL", "GND_%d_EOL", "HB_CONN_%d_EOL", "L_IND_%d_EOL", "R_IND_%d_EOL", "CYLINDER_DUT_%d_EOL", "CYL_PB_1_%d_EOL", "CYL_PB_2_%d_EOL", "DUT_PASS_%d_EOL", "DUT_FAIL_%d_EOL", "SPARE1_%d_EOL", "Tower Red_EOL", "Tower Amber_EOL", "Tower Green_EOL", "Tower Buzzer_EOL"] ("Relay_Channel_OUT")
            n231 = local read "EOL/FCT"() -> (w736:bool)
            n232 = local write "Barcode"("" ("Barcode")) -> ()
            n233 = Select(t=w738, s=w736, f=w737) -> (s? t:f=w739:T28[])
            n234 = local read "Relay"() -> (w740:refnum<queue>)
            n235 = call "Relay_CYL.vi"("DUT"=w734, "EOL/FCT"=w736, "DOs"=bool[] [TRUE, FALSE, FALSE, FALSE, FALSE], "Relay_Channel_Out"=w739, "Relay"=w740) -> ()  [unwired: 6 in, 1 out]
          }
          frame #1 {
            n236 = Wait (ms)(milliseconds to wait=u32 2000) -> ()  [unwired: 1 out]
          }
        }
        n237 = To Variant(anything=TRUE ("EOL/FCT")) -> (Variant=w729:variant)
        n238 = Bundle By Name(cluster=T25 {"Message"="", "Message Data"=variant} ("element"), "Message"="Initialize", "Message Data"=w729) -> (w733:T25)
        n239 = Enqueue Element At Opposite End(queue=w730, element=w733, error in (no error)=w722) -> (error out=w727:errorcluster)  [unwired: 1 in, 2 out]
      }
      frame "Product_CNT" {
        n240 = Unbundle By Name(w758) -> ("Configuration path"=w756:path, "Part Count"=w757:T1, "InitPro"=w751:bool, "DUT"=w748:i32)
        n241 = Number To Decimal String(number=w748) -> (decimal integer string=w749:string)  [unwired: 1 in]
        n242 = Concatenate Strings("OEE", w749, ".ini") -> (w746:string)
        n243 = Build Path(base path=w756, name or relative path=w746) -> (appended path=w755:path)
        n244 = call "ProductCount.vi"("DUT"=w748, "instrument file path"=w755, "error in (no error)"=w760, "Init"=w751, "Key_name"=string[] ["Total Run", "Pass", "Fail"], "Part Count"=w757) -> ("error out"=w759:errorcluster, "Part Count  2"=w752:T1)  [unwired: 4 in]
        "Part Count" <- w752
        n245 = Bundle By Name(cluster=w758, "Part Count"=w752) -> (w753:T2)
      }
      frame "Barcode" {
        n246 = local read "EOL/FCT"() -> (w763:bool)
        n247 = Tick Count (ms)() -> (millisecond timer value=w761:u32)
        n248 = case shown="False" w763 {
          tunnel: [w771 w786] -> w766
          tunnel: w762 -> [w783 w785]
          tunnel: [w768 w791] -> w765
          tunnel: w764 -> [w781 w787]
          tunnel: w762 -> [w770 w791]
          tunnel: w761 -> [w767 _]
          frame False {
            (unwired) "StartTest" ("Message")
            n249 = Unbundle By Name(w783) -> ("EQUP LIST"=w779:string[], "Array_Q"=w780:refnum<queue>[], "Test2_Q"=w769:refnum<queue>)
            n250 = Search 1D Array(1D array=w779, element="Barcode Scanner") -> (index of element=w775:i32)  [unwired: 1 in]
            n251 = Index Array(array=w780, index=w775) -> (element=w778:refnum<queue>)
            n252 = call "Enque_Message_FGV.vi"("Priority"=TRUE ("Priority Message? (F)"), "error in (no error)"=w781, "Message"="Write_trig", "queue Out"=w778) -> ("error out"=w772:errorcluster)  [unwired: 7 in]
            n253 = call "Test_Enque_Message_FGV.vi"("Priority"=TRUE ("Priority Message? (F)"), "error in (no error)"=w772, "Message"="CheckDUT", "queue in"=w769) -> ("error out"=w771:errorcluster)  [unwired: 7 in]
            n254 = Bundle By Name(cluster=w770, "Barcodetime"=w767) -> (w768:T2)
          }
          frame True {
            n255 = Unbundle By Name(w785) -> ("Test2_Q"=w784:refnum<queue>)
            n256 = Bundle By Name(cluster=T25 {"Message"="", "Message Data"=variant} ("element"), "Message"="StartTest") -> (w789:T25)
            n257 = Enqueue Element(queue=w784, element=w789, error in (no error)=w787) -> (error out=w786:errorcluster)  [unwired: 1 in, 2 out]
          }
        }
      }
      frame "StartTest" {
        w802 = ""
        # "Start Test"
        n258 = control-ref of="STATUS"() -> (w809:refnum<vi>)
        n259 = call "FGV_camera_status.vi"("Enum"=enum16{"Init", "Read", "Write"}."Write", "Write"=T34 {"Status"="", "Free/inuse"=FALSE, "Action"=""}) -> ()  [unwired: 9 in, 1 out]
        n260 = property class="Bool (strict)"(reference=w809, "Colors [4]"=cluster{u32, u32}[] [{3381759, 3381759}], "BoolText.Text"="Running" ("Boolean Text.Text"), "BoolText.FontBold"=TRUE ("Boolean Text.Font:Bold")) -> ()  [unwired: 1 in, 2 out]
        n261 = local read "EOL/FCT"() -> (w794:bool)
        n262 = case shown="True" w794 {
          tunnel: w805 -> [_ w825]
          tunnel: w796 -> [w815 w818]
          tunnel: [w815 w817] -> w795
          frame False {
          }
          frame True {
            n263 = Unbundle By Name(w825) -> ("EQUP LIST"=w821:string[], "Array_Q"=w819:refnum<queue>[])
            n264 = Search 1D Array(1D array=w821, element="PCAN") -> (index of element=w820:i32)  [unwired: 1 in]
            n265 = Index Array(array=w819, index=w820) -> (element=w816:refnum<queue>)
            n266 = call "Enque_Message_FGV.vi"("Priority"=TRUE, "error in (no error)"=w818, "Message"="Initialize-PCAN", "queue IN"=w816) -> ("error out"=w817:errorcluster)  [unwired: 7 in]
          }
        }
        n267 = for {
          N: 200 -> [_]
          i -> [w829]
          n268 = control-ref of="Table"() -> (w832:refnum<vi>)
          n269 = Bundle By Name(cluster=T30 {"Row"=0, "Column"=0} ("Active Cell:Active Cell"), "Row"=w829, "Column"=5) -> (w831:T30)
          n270 = property class="Tbl (strict)"(reference=w832, "Active Cell"=w831) -> (reference out=w827:refnum<vi>)  [unwired: 1 in, 1 out]
          n271 = property class="Tbl (strict)"(reference=w827, "Cell BG Color"=u32 16448250 ("Active Cell:Cell Background Color")) -> ()  [unwired: 1 in, 2 out]
        }
        n272 = local write "Total Time(s)"(0 ("Total Time(s)")) -> ()
        n273 = property on="DTU Inspection Data" class="Str"("Value"="" ("Inspection Failed Segments")) -> ()  [unwired: 2 in, 2 out]
        n274 = call "Test_Enque_Message_FGV.vi"("error in (no error)"=w795, "Message"="ClearScreen", "queue in"=w803) -> ("error out"=w813:errorcluster)  [unwired: 8 in]
        n275 = Tick Count (ms)() -> (millisecond timer value=w793:u32)
        n276 = Bundle By Name(cluster=w805, "Seconds"=w793, "Test Started?"=TRUE, "Scriptno."=u64 0, "InitPro"=FALSE, "USL"=w802, "UNIT"=w802, "LSL"=w802) -> (w811:T2)
        n277 = Merge Errors(w813) -> (w814:errorcluster)
      }
      frame "ClearScreen" {
        w840 = string[][] [] ("Table")
        n278 = property on="DTU Inspection Data" class="Str"(error in=w834, "DisabledEnum"=T31."Disabled and Grayed Out" ("Disabled")) -> (error out=w833:errorcluster)  [unwired: 1 in, 1 out]
        n279 = Bundle By Name(cluster=w844, "Barcode Scanned?"=FALSE, "Table"=w840) -> (w841:T2)
        n280 = property on="Table" class="Tbl (strict)"("Value"=w840) -> ()  [unwired: 2 in, 2 out]
        n281 = property on="Abort" class="Bool"(error in=w833, "DisabledEnum"=T31."Enabled" ("Disabled")) -> (error out=w839:errorcluster)  [unwired: 1 in, 1 out]
        n282 = call "Test_Enque_Message_FGV.vi"("error in (no error)"=w839, "Message"="IndexScript", "queue in"=w837) -> ("error out"=w842:errorcluster)  [unwired: 8 in]
      }
      frame "CheckDUT" {
        n283 = Unbundle By Name(w857) -> ("Barcodetime"=w858:u32, "Barcode Scanned?"=w846:bool, "Array_N"=w852:refnum<notifier>[], "EQUP LIST"=w854:string[], "DUT"=w847:i32)
        n284 = Tick Count (ms)() -> (millisecond timer value=w864:u32)
        n285 = Search 1D Array(1D array=w854, element="Barcode Scanner") -> (index of element=w853:i32)  [unwired: 1 in]
        n286 = Subtract(x=w864, y=w858) -> (x-y=w863:u32)
        n287 = Divide(x=w863, y=u32 1000) -> (x/y=w861:dbl)
        n288 = Index Array(array=w852, index=w853) -> (element=w851:refnum<notifier>)
        n289 = To Unsigned Long Integer(number=w861) -> (unsigned 32bit integer=w860:u32)
        "Barcodetime" <- w860
        n290 = Greater Or Equal?(x=w860, y=u32 21) -> (x >= y?=w845:bool)
        n291 = case shown="False" w846 {
          tunnel: w857 -> [w873 w959]
          tunnel: [w872 w959] -> w856
          tunnel: w851 -> [w871 _]
          tunnel: w850 -> [w870 w956]
          tunnel: [w869 w955] -> w849
          tunnel: w848 -> [w868 w954]
          tunnel: w847 -> [w867 _]
          tunnel: w846 -> [w866 _]
          tunnel: w845 -> [w865 _]
          frame False {
            n292 = case shown="False" w865 {
              tunnel: w870 -> [w888 w903]
              tunnel: [w875 w902] -> w869
              tunnel: w871 -> [w886 w898]
              tunnel: w873 -> [w883 w905]
              tunnel: [w882 w904] -> w872
              tunnel: w868 -> [w874 w901]
              tunnel: w866 -> [_ w900]
              tunnel: w867 -> [_ w899]
              frame False {
                n293 = Wait on Notification(notifier=w886, timeout in ms (-1)=200, error in (no error)=w888) -> (notification=w884:T25, error out=w887:errorcluster)  [unwired: 1 in, 2 out]
                n294 = Unbundle(w884) -> ("Message"=w881:string)  [unwired: 1 out]
                n295 = call <vilib>:"Clear Errors.vi"("error in (no error)"=w887) -> ("error out"=w876:errorcluster)  [unwired: 5 in, 1 out]
                n296 = Not Equal?(x=w881, y="") -> (x != y?=w879:bool)
                n297 = case shown="False" w879 {
                  tunnel: w883 -> [w892 w897]
                  tunnel: [w891 w896] -> w882
                  tunnel: w881 -> [w893 w894]
                  frame False {
                    n298 = local write "Barcode"(w893) -> ()
                    n299 = Bundle By Name(cluster=w892, "Barcode"="", "Barcode Scanned?"=FALSE) -> (w891:T2)
                  }
                  frame True {
                    n300 = Bundle By Name(cluster=w897, "Barcode"=w894, "Barcode Scanned?"=TRUE) -> (w896:T2)
                    "Barcode" <- w894
                  }
                }
                n301 = call "Test_Enque_Message_FGV.vi"("Priority"=FALSE ("Priority Message? (F)"), "error in (no error)"=w876, "Message"="CheckDUT", "queue in"=w874) -> ("error out"=w875:errorcluster)  [unwired: 7 in]
              }
              frame True {
                n302 = case shown="False" w900 {
                  tunnel: w903 -> [w916 w947]
                  tunnel: [w915 w946] -> w902
                  tunnel: w901 -> [_ w945]
                  tunnel: w899 -> [w911 _]
                  tunnel: w898 -> [_ _]
                  frame False {
                    n303 = local read "EOL/FCT"() -> (w917:bool)
                    n304 = Select(t=T35 [{"On/Off"=FALSE, "OUTPUT_Relay_Channels"=enum."CYLINDER_DUT_%d_EOL"}] ("Relay_CH_Array"), s=w917, f=T35 [{"On/Off"=FALSE, "OUTPUT_Relay_Channels"=enum."CYLINDER_ON/OFF_%d_FCT"}] ("Relay_CH_Array")) -> (s? t:f=w920:T35)
                    n305 = Bundle(cluster=T36 {"Relay_CH_Array"=[]} ("output cluster"), "Relay_CH_Array"=w920) -> (w922:T36)
                    n306 = case shown="False" w917 {
                      tunnel: [w925 w938] -> w913
                      tunnel: w922 -> [w924 w937]
                      tunnel: w911 -> [w923 w934]
                      frame False {
                        # "FCT"
                        n307 = call "Sep_Bool.vi"("output cluster"=w924) -> ("DO_Bool"=w926:bool[], "Array"=w927:T28[])  [unwired: 1 in]
                        n308 = case shown="1" w923 {
                          tunnel: w927 -> [w930 w933]
                          tunnel: w926 -> [w929 w932]
                          tunnel: ["Digital_Write_FCT_2" ("Message") "Digital_Write_FCT_1" ("Message")] -> w925
                          frame 2, Default {
                            n309 = call "MAP_FGV_2.vi"("DOs"=w929, "Relay_Channel_Out"=w930) -> ()  [unwired: 7 in, 3 out]
                          }
                          frame 1 {
                            n310 = call "MAP_FGV.vi"("DOs"=w932, "Relay_Channel_Out"=w933) -> ()  [unwired: 7 in, 3 out]
                          }
                        }
                      }
                      frame True {
                        # "EOL"
                        n311 = call "Sep_Bool_EOL.vi"("output cluster"=w937) -> ("DO_Bool"=w936:bool[], "Array"=w935:T28[])  [unwired: 1 in]
                        n312 = case shown="1" w934 {
                          tunnel: w935 -> [w941 w944]
                          tunnel: w936 -> [w940 w943]
                          tunnel: ["Digital_Write_EOL_2" ("Message") "Digital_Write_EOL_1" ("Message")] -> w938
                          frame 2, Default {
                            n313 = call "MAP_FGV_EOL_2.vi"("DOs"=w940, "Relay_Channel_Out"=w941) -> ()  [unwired: 7 in, 3 out]
                          }
                          frame 1 {
                            n314 = call "MAP_FGV_EOL_1.vi"("DOs"=w943, "Relay_Channel_Out"=w944) -> ()  [unwired: 7 in, 3 out]
                          }
                        }
                      }
                    }
                    n315 = local read "Relay"() -> (w914:refnum<queue>)
                    n316 = Number To Decimal String(number=w911) -> (decimal integer string=w908:string)  [unwired: 1 in]
                    n317 = call "Enque_Message_FGV.vi"("Priority"=TRUE, "error in (no error)"=w916, "Message"=w913, "queue IN"=w914) -> ("error out"=w915:errorcluster)  [unwired: 7 in]
                    n318 = Concatenate Strings("Barcode not scanned at DUT" ("message"), w908, "Press CYCLE START to Scan again and start" ("string")) -> (w910:string)
                    n319 = One Button Dialog(message=w910, button name ("OK")="OK") -> ()  [unwired: 1 out]
                  }
                  frame True {
                    n320 = call "Test_Enque_Message_FGV.vi"("Priority"=TRUE ("Priority Message? (F)"), "error in (no error)"=w947, "Message"="StartTest", "queue in"=w945) -> ("error out"=w946:errorcluster)  [unwired: 7 in]
                    n321 = control-ref of="STATUS"() -> (w953:refnum<vi>)
                    n322 = property class="Bool (strict)"(reference=w953, "BoolText.Text"="Ready" ("Boolean Text.Text"), "Colors [4]"=cluster{u32, u32}[] [{16777238, 16777238}], "BoolText.FontBold"=TRUE ("Boolean Text.Font:Bold")) -> ()  [unwired: 1 in, 2 out]
                  }
                }
                n323 = Bundle By Name(cluster=w905, "Barcode Scanned?"=w900) -> (w904:T2)
              }
            }
          }
          frame True {
            n324 = call "Test_Enque_Message_FGV.vi"("Priority"=TRUE ("Priority Message? (F)"), "error in (no error)"=w956, "Message"="StartTest", "queue in"=w954) -> ("error out"=w955:errorcluster)  [unwired: 7 in]
          }
        }
      }
      frame "IndexScript" {
        # "Index Script"
        n325 = Unbundle By Name(w977) -> ("Selected_Scripts"=w976:T4[], "Scriptno."=w965:u64, "TotalScripts"=w966:u64)
        n326 = Index Array(array=w976, index=w965) -> (element=w967:T4)
        n327 = To Unsigned Byte Integer(number=w965) -> (unsigned 8bit integer=→"Test Progress...":u8)
        n328 = property on="Start Button" class="Bool"(error in=w963, "DisabledEnum"=T31."Disabled and Grayed Out" ("Disabled")) -> (error out=w962:errorcluster)  [unwired: 1 in, 1 out]
        n329 = Unbundle By Name(w967) -> ("Steps"=w974:T5[])
        n330 = Greater Or Equal?(x=w965, y=w966) -> (x >= y?=w972:bool)
        n331 = Array Size(array=w974) -> (size(s)=w973:i32)
        n332 = case shown="True" w972 {
          tunnel: w977 -> [w990 w993]
          tunnel: [w989 w992] -> w975
          tunnel: w973 -> [w987 _]
          tunnel: [string[] ["IndexStep"] ("Message Array") string[] ["StopTest", "Update Display", "Pass/Fail", "Product_CNT", "Save", "Print"] ("Message Array")] -> w968
          tunnel: w967 -> [w984 w991]
          frame False {
            n333 = To Unsigned Quad Integer(1:w987) -> (0:w985:u64)
            n334 = Bundle By Name(cluster=w990, "UI Data.ScriptDetails"=w984, "Stepno."=u64 0, "TotalSteps"=w985) -> (w989:T2)
          }
          frame True {
            n335 = Bundle By Name(cluster=w993, "UI Data.ScriptDetails"=w991) -> (w992:T2)
          }
        }
        n336 = disable-structure shown="Enabled" {
          disable-tunnel: [w980 w983] -> w971
          disable-tunnel: [w979 w982] -> w969
          disable-tunnel: w962 -> [w978 w983]
          disable-tunnel: w960 -> [_ w982]
          frame Disabled {
            n337 = call "Test_Queue_Comm_FGV.vi"("error in (no error)"=w978, "Enum"=Test_FGV_Queue_Control."Get") -> ("error Out"=w980:errorcluster, "queue Out"=w979:refnum<queue>)  [unwired: 8 in]
          }
          frame Enabled {
          }
        }
        n338 = call "Test_Enqueue Message (Array).vi"("error in (no error)"=w971, "Message Array"=w968, "Message Queue"=w969) -> ("error out"=w970:errorcluster)  [unwired: 7 in, 1 out]
      }
      frame "IndexStep" {
        # "Waittime"
        n339 = Unbundle By Name(w1002) -> ("Scriptno."=w996:u64, "Stepno."=w1001:u64, "TotalSteps"=w1000:u64)
        n340 = Greater Or Equal?(x=w1001, y=w1000) -> (x >= y?=w997:bool)
        n341 = case shown="True" w997 {
          tunnel: w1002 -> [w1012 w1027]
          tunnel: [w1007 w1026] -> w999
          tunnel: w998 -> [w1009 w1022]
          tunnel: [w1008 w1020] -> _
          tunnel: w996 -> [_ w1025]
          tunnel: w995 -> [w1005 w1019]
          frame False {
            (unwired) string[] ["LaunchStep", "Waittime", "StepFeedback"] ("Message")
            n342 = disable-structure shown="Enabled" {
              disable-tunnel: [w1015 w1018] -> w1011
              disable-tunnel: [w1014 w1017] -> w1010
              disable-tunnel: w1009 -> [w1013 w1018]
              disable-tunnel: w1005 -> [_ w1017]
              frame Disabled {
                n343 = call "Test_Queue_Comm_FGV.vi"("error in (no error)"=w1013, "Enum"=Test_FGV_Queue_Control."Get") -> ("error Out"=w1015:errorcluster, "queue Out"=w1014:refnum<queue>)  [unwired: 8 in]
              }
              frame Enabled {
              }
            }
            n344 = Bundle By Name(cluster=w1012, "LaunchStep"=TRUE) -> (w1007:T2)
            n345 = call "Test_Enqueue Message (Array).vi"("Priority Message? Array"=bool[] [TRUE, TRUE, TRUE], "error in (no error)"=w1011, "Message Array"=string[] ["Waittime", "LaunchStep", "StepFeedback"] ("Message"), "Message Queue"=w1010) -> ("error out"=w1008:errorcluster)  [unwired: 6 in, 1 out]
          }
          frame True {
            n346 = Increment(x=w1025) -> (x+1=w1024:u64)
            n347 = call "Test_Enque_Message_FGV.vi"("error in (no error)"=w1022, "Message"="IndexScript", "queue in"=w1019) -> ("error out"=w1021:errorcluster)  [unwired: 8 in]
            n348 = Bundle By Name(cluster=w1027, "Scriptno."=w1024) -> (w1026:T2)
            n349 = flat-sequence {
              tunnel: w1021 -> [w1030]
              tunnel: [w1029] -> w1020
              frame #0 {
                n350 = call "Time Delay"("error in (no error)"=w1030, "Delay Time (s)"=0.7) -> ("error out"=w1029:errorcluster)  [unwired: 9 in]
              }
            }
          }
        }
      }
      frame "LaunchStep" {
        (unwired) T11 0 items=["POWER SUPPLY", "DMM", "DAQ", "CAMERA"] ("EQUIPMENT")
        (unwired) string[] ["<Select>", "MP711134-14V", "MP711134-12V", "Keysight34461a", "DMM6500", "PCAN", "Relay_Module", "GNSS", "Bluetooth", "Noeway_Flashing", "MCU_Flashing"] ("Strings []")
        (unwired) StepType."RELAY_CHANNEL_WRITE" ("Type")
        # "Perform tests"
        n351 = Unbundle By Name(w1040) -> ("Barcode"=w1032:string, "Test2_Q"=w1033:refnum<queue>, "EQUP LIST"=w1034:string[], "config"=w1036:string, "Array_Q"=w1037:refnum<queue>[], "DUT"=w1038:i32, "UI Data.ScriptDetails.Steps"=w1047:T5[], "Stepno."=w1046:u64)
        n352 = Index Array(array=w1047, index=w1046) -> (element=w1045:T5)
        n353 = call "Conf_select.vi"("Config"=w1036) -> ("index of element"=w1035:i32)
        n354 = Unbundle By Name(w1045) -> ("StepDetails"=w1041:string, "Type"=w1044:T6, "StepName"=w1031:string)
        n355 = case shown="\"Camera\"" w1044 {
          tunnel: w1043 -> [w1068 w1112 w1156 w1344 w1394 w1436 w1459 w1494 w1558 w1577 w1590]
          tunnel: [w1061 w1108 w1153 w1343 w1393 w1442 w1460 w1491 w1553 w1569 w1581] -> w1042
          tunnel: w1041 -> [w1067 w1111 w1155 w1342 w1391 w1435 w1453 w1492 w1555 w1574 w1587]
          tunnel: w1040 -> [w1066 w1110 w1150 w1338 w1399 w1443 w1457 w1493 w1557 w1576 w1589]
          tunnel: [w1057 w1100 w1149 w1336 w1387 w1433 w1454 w1490 w1546 w1572 w1585] -> w1039
          tunnel: w1038 -> [w1058 _ _ _ _ _ _ w1484 _ _ _]
          tunnel: w1037 -> [w1050 w1102 w1148 w1341 w1390 w1426 w1448 w1489 w1544 w1561 w1582]
          tunnel: w1035 -> [w1059 _ _ _ _ _ _ _ _ _ _]
          tunnel: w1034 -> [w1051 w1096 w1141 w1334 w1383 w1429 w1449 _ _ _ _]
          tunnel: w1033 -> [_ _ _ _ _ _ _ w1488 _ _ _]
          tunnel: w1032 -> [_ _ _ _ _ _ w1444 _ _ _ _]
          tunnel: w1031 -> [_ _ _ _ _ _ w1447 _ _ _ _]
          frame "RELAY_CHANNEL_WRITE", Default {
            n356 = Unflatten From String(type=T13 {"Relay_CH_Array"=[]} ("Set_Channel_Relay"), binary string=w1067, error in (no error)=w1068) -> (value=w1060:T13, error out=w1065:errorcluster)  [unwired: 2 in, 1 out]
            n357 = Search 1D Array(1D array=w1051, element="Relay_Module") -> (index of element=w1049:i32)  [unwired: 1 in]
            n358 = call "Ring-to-enum.vi"("Set_Channel_Relay"=w1060) -> ("output cluster"=w1054:T36)  [unwired: 10 in]
            n359 = Index Array(array=w1050, index=w1049) -> (element=w1048:refnum<queue>)
            n360 = case shown="1" w1059 {
              tunnel: [w1071 w1084] -> w1064
              tunnel: w1054 -> [w1070 w1083]
              tunnel: w1058 -> [w1069 w1080]
              frame 0, Default {
                # "FCT"
                n361 = call "Sep_Bool.vi"("output cluster"=w1070) -> ("DO_Bool"=w1072:bool[], "Array"=w1073:T28[])  [unwired: 1 in]
                n362 = case shown="1" w1069 {
                  tunnel: w1073 -> [w1076 w1079]
                  tunnel: w1072 -> [w1075 w1078]
                  tunnel: ["Digital_Write_FCT_2" ("Message") "Digital_Write_FCT_1" ("Message")] -> w1071
                  frame 2, Default {
                    n363 = call "MAP_FGV_2.vi"("DOs"=w1075, "Relay_Channel_Out"=w1076) -> ()  [unwired: 7 in, 3 out]
                  }
                  frame 1 {
                    n364 = call "MAP_FGV.vi"("DOs"=w1078, "Relay_Channel_Out"=w1079) -> ()  [unwired: 7 in, 3 out]
                  }
                }
              }
              frame 1 {
                # "EOL"
                n365 = call "Sep_Bool_EOL.vi"("output cluster"=w1083) -> ("DO_Bool"=w1082:bool[], "Array"=w1081:T28[])  [unwired: 1 in]
                n366 = case shown="1" w1080 {
                  tunnel: w1081 -> [w1087 w1090]
                  tunnel: w1082 -> [w1086 w1089]
                  tunnel: ["Digital_Write_EOL_2" ("Message") "Digital_Write_EOL_1" ("Message")] -> w1084
                  frame 2, Default {
                    n367 = call "MAP_FGV_EOL_2.vi"("DOs"=w1086, "Relay_Channel_Out"=w1087) -> ()  [unwired: 7 in, 3 out]
                  }
                  frame 1 {
                    n368 = call "MAP_FGV_EOL_1.vi"("DOs"=w1089, "Relay_Channel_Out"=w1090) -> ()  [unwired: 7 in, 3 out]
                  }
                }
              }
            }
            n369 = Bundle By Name(cluster=w1066, "LaunchStep"=TRUE, "Delay"=FALSE) -> (w1057:T2)
            n370 = To Variant(anything=w1054) -> (Variant=w1063:variant)
            n371 = call "Enque_Message_FGV.vi"("Priority"=TRUE, "error in (no error)"=w1065, "Message Data"=w1063, "Message"=w1064, "queue IN"=w1048) -> ("error out"=w1061:errorcluster)  [unwired: 6 in]
          }
          frame "PS_WRITE" {
            n372 = Unflatten From String(type=T7 {"Set_parameter"=0, "VOLTAGE"="", "CURRENT"="", "OUTPUT"=FALSE, "Delay"=FALSE, "Delay time"=0.0} ("PS_Write"), binary string=w1111, error in (no error)=w1112) -> (value=w1106:T7, error out=w1109:errorcluster)  [unwired: 2 in, 1 out]
            n373 = Unbundle By Name(w1106) -> ("Delay time"=w1099:dbl, "Delay"=w1098:bool, "Set_parameter"=w1105:T8, "VOLTAGE"=w1094:string, "CURRENT"=w1103:string, "OUTPUT"=w1104:bool)
            n374 = Concatenate Strings("MP711134-", w1094, "V") -> (w1092:string)
            n375 = Search 1D Array(1D array=w1096, element=w1092) -> (index of element=w1091:i32)  [unwired: 1 in]
            n376 = Index Array(array=w1102, index=w1091) -> (element=w1101:refnum<queue>)
            n377 = Bundle By Name(cluster=w1110, "Delay time"=w1099, "Delay"=w1098, "LaunchStep"=TRUE) -> (w1100:T2)
            n378 = case shown="2" w1105 {
              tunnel: w1109 -> [w1120 w1128 w1139]
              tunnel: [w1119 w1127 w1138] -> w1108
              tunnel: w1104 -> [_ _ w1131]
              tunnel: w1103 -> [_ w1122 _]
              tunnel: w1094 -> [w1113 _ _]
              tunnel: w1101 -> [w1114 w1121 w1129]
              frame 0, Default {
                # "Set_Voltage"
                n379 = To Variant(anything=w1113) -> (Variant=w1115:variant)
                n380 = Bundle(cluster=T25 {"Message"="", "Message Data"=variant} ("element"), "Message"="Set_Voltage", "Message Data"=w1115) -> (w1118:T25)
                n381 = Enqueue Element At Opposite End(queue=w1114, element=w1118, error in (no error)=w1120) -> (error out=w1119:errorcluster)  [unwired: 1 in, 2 out]
              }
              frame 1 {
                # "Set_current"
                n382 = To Variant(anything=w1122) -> (Variant=w1123:variant)
                n383 = Bundle(cluster=T25 {"Message"="", "Message Data"=variant} ("element"), "Message"="Set_Current", "Message Data"=w1123) -> (w1126:T25)
                n384 = Enqueue Element At Opposite End(queue=w1121, element=w1126, error in (no error)=w1128) -> (error out=w1127:errorcluster)  [unwired: 1 in, 2 out]
              }
              frame 2 {
                # "Output"
                n385 = Select(t="ON", s=w1131, f="OFF") -> (s? t:f=w1130:string)
                n386 = To Variant(anything=w1130) -> (Variant=w1134:variant)
                n387 = Bundle(cluster=T25 {"Message"="", "Message Data"=variant} ("element"), "Message"="Output_ONOFF", "Message Data"=w1134) -> (w1137:T25)
                n388 = Enqueue Element At Opposite End(queue=w1129, element=w1137, error in (no error)=w1139) -> (error out=w1138:errorcluster)  [unwired: 1 in, 2 out]
              }
            }
          }
          frame "READ_DATA" {
            n389 = Unflatten From String(type=T10 {"EQUIPMENT"=1, "PARAMETER"=0, "LSL"=0.0, "USL"=0.0, "RESULT"="", "UNIT"="", "Delay"=FALSE, "Delay time"=0.0} ("READ_DATA"), binary string=w1155, error in (no error)=w1156) -> (value=w1147:T10, error out=w1154:errorcluster)  [unwired: 2 in, 1 out]
            n390 = Unbundle By Name(w1147) -> ("Delay"=w1144:bool, "Delay time"=w1143:dbl, "EQUIPMENT"=w1152:T11, "PARAMETER"=w1151:T12, "RESULT"=w1140:string)
            n391 = Bundle By Name(cluster=w1150, "Delay"=w1144, "Delay time"=w1143, "LaunchStep"=TRUE) -> (w1145:T2)
            n392 = case shown="1" w1152 {
              tunnel: w1154 -> [w1169 w1217 w1233 w1287]
              tunnel: [w1168 w1216 w1232 w1286] -> w1153
              tunnel: w1151 -> [w1167 _ w1231 w1285]
              tunnel: w1145 -> [w1166 w1223 w1230 w1284]
              tunnel: [w1165 w1223 w1229 w1283] -> w1149
              tunnel: w1148 -> [w1164 w1215 w1228 w1282]
              tunnel: w1141 -> [w1162 _ w1226 w1279]
              tunnel: w1140 -> [w1159 _ _ _]
              frame 0 {
                (unwired) T12 0 items=["SET_VOLTAGE", "SET_CURRENT", "OUTPUT VOLTAGE", "OUTPUT CURRENT", "RESISTANCE", "OUTPUT POWER", "CAMERA", "SSL_Check"] ("PARAMETER")
                # "PS"
                n393 = Concatenate Strings("MP711134-", w1159, "V") -> (w1158:string)
                n394 = Search 1D Array(1D array=w1162, element=w1158) -> (index of element=w1157:i32)  [unwired: 1 in]
                n395 = Index Array(array=w1164, index=w1157) -> (element=w1163:refnum<queue>)
                n396 = case shown="3" w1167 {
                  tunnel: w1169 -> [w1173 w1182 w1191 w1200 w1209]
                  tunnel: [w1174 w1181 w1190 w1199 w1208] -> w1168
                  tunnel: w1166 -> [w1172 w1180 w1189 w1198 w1207]
                  tunnel: [w1172 w1180 w1189 w1198 w1207] -> w1165
                  tunnel: w1163 -> [w1171 w1179 w1188 w1197 w1206]
                  frame 0, Default {
                    w1170 = "Read_Voltage" ("Message")
                    # "Read_VOLTAGE"
                    n397 = To Variant(anything=w1170) -> (Variant=w1175:variant)
                    n398 = Bundle(cluster=T25 {"Message"="", "Message Data"=variant} ("element"), "Message"=w1170, "Message Data"=w1175) -> (w1177:T25)
                    n399 = Enqueue Element At Opposite End(queue=w1171, element=w1177, error in (no error)=w1173) -> (error out=w1174:errorcluster)  [unwired: 1 in, 2 out]
                  }
                  frame 1 {
                    # "Read_CURRENT"
                    n400 = To Variant(anything="") -> (Variant=w1183:variant)
                    n401 = Bundle(cluster=T25 {"Message"="", "Message Data"=variant} ("element"), "Message"="Read_Current", "Message Data"=w1183) -> (w1185:T25)
                    n402 = Enqueue Element At Opposite End(queue=w1179, element=w1185, error in (no error)=w1182) -> (error out=w1181:errorcluster)  [unwired: 1 in, 2 out]
                  }
                  frame 2 {
                    # "OUTPUT VOLTAGE"
                    n403 = To Variant(anything="") -> (Variant=w1192:variant)
                    n404 = Bundle(cluster=T25 {"Message"="", "Message Data"=variant} ("element"), "Message"="Read_Voltage", "Message Data"=w1192) -> (w1194:T25)
                    n405 = Enqueue Element At Opposite End(queue=w1188, element=w1194, error in (no error)=w1191) -> (error out=w1190:errorcluster)  [unwired: 1 in, 2 out]
                  }
                  frame 3 {
                    # "OUTPUT CURRENT"
                    n406 = To Variant(anything="") -> (Variant=w1201:variant)
                    n407 = Bundle(cluster=T25 {"Message"="", "Message Data"=variant} ("element"), "Message"="Read_Current", "Message Data"=w1201) -> (w1203:T25)
                    n408 = Enqueue Element At Opposite End(queue=w1197, element=w1203, error in (no error)=w1200) -> (error out=w1199:errorcluster)  [unwired: 1 in, 2 out]
                  }
                  frame 4 {
                    # "RESISTANCE"
                    n409 = To Variant(anything="") -> (Variant=w1210:variant)
                    n410 = Bundle(cluster=T25 {"Message"="", "Message Data"=variant} ("element"), "Message"="Read_Resistance", "Message Data"=w1210) -> (w1212:T25)
                    n411 = Enqueue Element At Opposite End(queue=w1206, element=w1212, error in (no error)=w1209) -> (error out=w1208:errorcluster)  [unwired: 1 in, 2 out]
                  }
                }
              }
              frame 3, Default {
                # "CAMERA"
                n412 = Array Size(array=w1215) -> (size(s)=w1222:i32)
                n413 = Decrement(x=w1222) -> (x-1=w1221:i32)
                n414 = Index Array(array=w1215, index=w1221) -> (element=w1214:refnum<queue>)
                n415 = Bundle(cluster=T25 {"Message"="", "Message Data"=variant} ("element"), "Message"="Trigger") -> (w1219:T25)  [unwired: 1 in]
                n416 = Enqueue Element At Opposite End(queue=w1214, element=w1219, error in (no error)=w1217) -> (error out=w1216:errorcluster)  [unwired: 1 in, 2 out]
              }
              frame 1 {
                # "DMM"
                n417 = Search 1D Array(1D array=w1226, element="Keysight34461a") -> (index of element=w1224:i32)  [unwired: 1 in]
                n418 = Index Array(array=w1228, index=w1224) -> (element=w1227:refnum<queue>)
                n419 = case shown="4" w1231 {
                  tunnel: w1233 -> [w1237 w1246 w1255 w1264 w1273]
                  tunnel: [w1238 w1245 w1254 w1263 w1272] -> w1232
                  tunnel: w1230 -> [w1236 w1244 w1253 w1262 w1271]
                  tunnel: [w1236 w1244 w1253 w1262 w1271] -> w1229
                  tunnel: w1227 -> [w1235 w1243 w1252 w1261 w1270]
                  frame 0, Default {
                    w1234 = "Read" ("Message")
                    # "Read_VOLTAGE"
                    n420 = To Variant(anything=w1234) -> (Variant=w1239:variant)
                    n421 = Bundle(cluster=T25 {"Message"="", "Message Data"=variant} ("element"), "Message"=w1234, "Message Data"=w1239) -> (w1241:T25)
                    n422 = Enqueue Element At Opposite End(queue=w1235, element=w1241, error in (no error)=w1237) -> (error out=w1238:errorcluster)  [unwired: 1 in, 2 out]
                  }
                  frame 1 {
                    # "Read_CURRENT"
                    n423 = To Variant(anything="") -> (Variant=w1247:variant)
                    n424 = Bundle(cluster=T25 {"Message"="", "Message Data"=variant} ("element"), "Message"="Read", "Message Data"=w1247) -> (w1249:T25)
                    n425 = Enqueue Element At Opposite End(queue=w1243, element=w1249, error in (no error)=w1246) -> (error out=w1245:errorcluster)  [unwired: 1 in, 2 out]
                  }
                  frame 2 {
                    # "OUTPUT VOLTAGE"
                    n426 = To Variant(anything="") -> (Variant=w1256:variant)
                    n427 = Bundle(cluster=T25 {"Message"="", "Message Data"=variant} ("element"), "Message"="Read", "Message Data"=w1256) -> (w1258:T25)
                    n428 = Enqueue Element At Opposite End(queue=w1252, element=w1258, error in (no error)=w1255) -> (error out=w1254:errorcluster)  [unwired: 1 in, 2 out]
                  }
                  frame 3 {
                    # "OUTPUT CURRENT"
                    n429 = To Variant(anything="") -> (Variant=w1265:variant)
                    n430 = Bundle(cluster=T25 {"Message"="", "Message Data"=variant} ("element"), "Message"="Read", "Message Data"=w1265) -> (w1267:T25)
                    n431 = Enqueue Element At Opposite End(queue=w1261, element=w1267, error in (no error)=w1264) -> (error out=w1263:errorcluster)  [unwired: 1 in, 2 out]
                  }
                  frame 4 {
                    # "RESISTANCE"
                    n432 = To Variant(anything="") -> (Variant=w1274:variant)
                    n433 = Bundle(cluster=T25 {"Message"="", "Message Data"=variant} ("element"), "Message"="Read", "Message Data"=w1274) -> (w1276:T25)
                    n434 = Enqueue Element At Opposite End(queue=w1270, element=w1276, error in (no error)=w1273) -> (error out=w1272:errorcluster)  [unwired: 1 in, 2 out]
                  }
                }
              }
              frame 2 {
                # "DAQ"
                n435 = Search 1D Array(1D array=w1279, element="DMM6500") -> (index of element=w1278:i32)  [unwired: 1 in]
                n436 = Index Array(array=w1282, index=w1278) -> (element=w1281:refnum<queue>)
                n437 = case shown="0, Default" w1285 {
                  tunnel: w1287 -> [w1291 w1300 w1309 w1318 w1327]
                  tunnel: [w1292 w1299 w1308 w1317 w1326] -> w1286
                  tunnel: w1284 -> [w1290 w1298 w1307 w1316 w1325]
                  tunnel: [w1290 w1298 w1307 w1316 w1325] -> w1283
                  tunnel: w1281 -> [w1289 w1297 w1306 w1315 w1324]
                  frame 0, Default {
                    w1288 = "Measure" ("Message")
                    # "Read_VOLTAGE"
                    n438 = To Variant(anything=w1288) -> (Variant=w1293:variant)
                    n439 = Bundle(cluster=T25 {"Message"="", "Message Data"=variant} ("element"), "Message"=w1288, "Message Data"=w1293) -> (w1295:T25)
                    n440 = Enqueue Element At Opposite End(queue=w1289, element=w1295, error in (no error)=w1291) -> (error out=w1292:errorcluster)  [unwired: 1 in, 2 out]
                  }
                  frame 1 {
                    # "Read_CURRENT"
                    n441 = To Variant(anything="") -> (Variant=w1301:variant)
                    n442 = Bundle(cluster=T25 {"Message"="", "Message Data"=variant} ("element"), "Message"="Measure", "Message Data"=w1301) -> (w1303:T25)
                    n443 = Enqueue Element At Opposite End(queue=w1297, element=w1303, error in (no error)=w1300) -> (error out=w1299:errorcluster)  [unwired: 1 in, 2 out]
                  }
                  frame 2 {
                    # "OUTPUT VOLTAGE"
                    n444 = To Variant(anything="") -> (Variant=w1310:variant)
                    n445 = Bundle(cluster=T25 {"Message"="", "Message Data"=variant} ("element"), "Message"="Measure", "Message Data"=w1310) -> (w1312:T25)
                    n446 = Enqueue Element At Opposite End(queue=w1306, element=w1312, error in (no error)=w1309) -> (error out=w1308:errorcluster)  [unwired: 1 in, 2 out]
                  }
                  frame 3 {
                    # "OUTPUT CURRENT"
                    n447 = To Variant(anything="") -> (Variant=w1319:variant)
                    n448 = Bundle(cluster=T25 {"Message"="", "Message Data"=variant} ("element"), "Message"="Measure", "Message Data"=w1319) -> (w1321:T25)
                    n449 = Enqueue Element At Opposite End(queue=w1315, element=w1321, error in (no error)=w1318) -> (error out=w1317:errorcluster)  [unwired: 1 in, 2 out]
                  }
                  frame 4 {
                    # "RESISTANCE"
                    n450 = To Variant(anything="") -> (Variant=w1328:variant)
                    n451 = Bundle(cluster=T25 {"Message"="", "Message Data"=variant} ("element"), "Message"="Measure", "Message Data"=w1328) -> (w1330:T25)
                    n452 = Enqueue Element At Opposite End(queue=w1324, element=w1330, error in (no error)=w1327) -> (error out=w1326:errorcluster)  [unwired: 1 in, 2 out]
                  }
                }
              }
            }
          }
          frame "DAQ_CONFIG" {
            n453 = Search 1D Array(1D array=w1334, element="DMM6500") -> (index of element=w1332:i32)  [unwired: 1 in]
            n454 = Unflatten From String(type=T15 {"AUTO RANGE"=FALSE, "CHANNEL LIST"="", "SELECT Card"=0, "SELECT SLOT"=0, "Function"=0} ("DAQ_Config"), binary string=w1342, error in (no error)=w1344) -> (value=w1339:T15, error out=w1348:errorcluster)  [unwired: 2 in, 1 out]
            n455 = Index Array(array=w1341, index=w1332) -> (element=w1340:refnum<queue>)
            n456 = Unbundle By Name(w1339) -> ("Function"=w1347:i32, "AUTO RANGE"=w1345:bool, "CHANNEL LIST"=w1346:string)
            n457 = Bundle By Name(cluster=w1338, "LaunchStep"=TRUE) -> (w1336:T2)
            n458 = case shown="0, Default" w1347 {
              tunnel: w1348 -> [w1356 w1364 w1372 w1380]
              tunnel: [w1355 w1363 w1371 w1379] -> w1343
              tunnel: w1346 -> [_ _ _ _]
              tunnel: w1345 -> [_ _ _ _]
              tunnel: w1340 -> [w1350 w1358 w1366 w1374]
              tunnel: w1339 -> [w1349 w1357 w1365 w1373]
              frame 0, Default {
                # "Voltage"
                n459 = To Variant(anything=w1349) -> (Variant=w1351:variant)
                n460 = Bundle(cluster=T25 {"Message"="", "Message Data"=variant} ("element"), "Message"="Configure", "Message Data"=w1351) -> (w1354:T25)
                n461 = Enqueue Element At Opposite End(queue=w1350, element=w1354, error in (no error)=w1356) -> (error out=w1355:errorcluster)  [unwired: 1 in, 2 out]
              }
              frame 1 {
                # "current"
                n462 = To Variant(anything=w1357) -> (Variant=w1359:variant)
                n463 = Bundle(cluster=T25 {"Message"="", "Message Data"=variant} ("element"), "Message"="Configure", "Message Data"=w1359) -> (w1362:T25)
                n464 = Enqueue Element At Opposite End(queue=w1358, element=w1362, error in (no error)=w1364) -> (error out=w1363:errorcluster)  [unwired: 1 in, 2 out]
              }
              frame 2 {
                # "Resistance"
                n465 = To Variant(anything=w1365) -> (Variant=w1367:variant)
                n466 = Bundle(cluster=T25 {"Message"="", "Message Data"=variant} ("element"), "Message"="Configure", "Message Data"=w1367) -> (w1370:T25)
                n467 = Enqueue Element At Opposite End(queue=w1366, element=w1370, error in (no error)=w1372) -> (error out=w1371:errorcluster)  [unwired: 1 in, 2 out]
              }
              frame 3 {
                # "Power"
                n468 = To Variant(anything=w1373) -> (Variant=w1375:variant)
                n469 = Bundle(cluster=T25 {"Message"="", "Message Data"=variant} ("element"), "Message"="Configure", "Message Data"=w1375) -> (w1378:T25)
                n470 = Enqueue Element At Opposite End(queue=w1374, element=w1378, error in (no error)=w1380) -> (error out=w1379:errorcluster)  [unwired: 1 in, 2 out]
              }
            }
          }
          frame "DMM_CONFIG" {
            n471 = Search 1D Array(1D array=w1383, element="Keysight34461a") -> (index of element=w1381:i32)  [unwired: 1 in]
            n472 = Unflatten From String(type=T9 {"CONFIG PARAMETER"=0, "AUTO RANGE"=FALSE, "RANGE"="", "Delay"=FALSE, "Delay time"=0.0} ("DMM_CONFIG"), binary string=w1391, error in (no error)=w1394) -> (value=w1388:T9, error out=w1398:errorcluster)  [unwired: 2 in, 1 out]
            n473 = Index Array(array=w1390, index=w1381) -> (element=w1389:refnum<queue>)
            n474 = Unbundle By Name(w1388) -> ("Delay"=w1385:bool, "Delay time"=w1384:dbl, "CONFIG PARAMETER"=w1397:u16, "AUTO RANGE"=w1395:bool, "RANGE"=w1396:string)
            n475 = Bundle By Name(cluster=w1399, "LaunchStep"=TRUE, "Delay"=w1385, "Delay time"=w1384) -> (w1387:T2)
            n476 = case shown="1, 2" w1397 {
              tunnel: w1398 -> [w1400 w1408 w1416 w1424]
              tunnel: [w1400 w1407 w1415 w1423] -> w1393
              tunnel: w1396 -> [_ _ _ _]
              tunnel: w1395 -> [_ _ _ _]
              tunnel: w1389 -> [_ w1402 w1410 w1418]
              tunnel: w1388 -> [_ w1401 w1409 w1417]
              frame 3, Default {
              }
              frame 1, 2 {
                # "Current"
                n477 = To Variant(anything=w1401) -> (Variant=w1403:variant)
                n478 = Bundle(cluster=T25 {"Message"="", "Message Data"=variant} ("element"), "Message"="Configure", "Message Data"=w1403) -> (w1406:T25)
                n479 = Enqueue Element At Opposite End(queue=w1402, element=w1406, error in (no error)=w1408) -> (error out=w1407:errorcluster)  [unwired: 1 in, 2 out]
              }
              frame 5, 7 {
                # "Resistance"
                n480 = To Variant(anything=w1409) -> (Variant=w1411:variant)
                n481 = Bundle(cluster=T25 {"Message"="", "Message Data"=variant} ("element"), "Message"="Configure", "Message Data"=w1411) -> (w1414:T25)
                n482 = Enqueue Element At Opposite End(queue=w1410, element=w1414, error in (no error)=w1416) -> (error out=w1415:errorcluster)  [unwired: 1 in, 2 out]
              }
              frame 9, 10 {
                # "Voltage"
                n483 = To Variant(anything=w1417) -> (Variant=w1419:variant)
                n484 = Bundle(cluster=T25 {"Message"="", "Message Data"=variant} ("element"), "Message"="Configure", "Message Data"=w1419) -> (w1422:T25)
                n485 = Enqueue Element At Opposite End(queue=w1418, element=w1422, error in (no error)=w1424) -> (error out=w1423:errorcluster)  [unwired: 1 in, 2 out]
              }
            }
          }
          frame "PCAN_Read" {
            n486 = Search 1D Array(1D array=w1429, element="PCAN") -> (index of element=w1427:i32)  [unwired: 1 in]
            n487 = Unflatten From String(type=T19 {"Database"="", "Signal"="", "BYTES"=[], "ReadPayload"=[], "String_Data"="", "ReadValue"=0.0, "CANID"=0, "SERVICE ID"=0, "SUB-SERVICE ID"=0, "DELAY "=FALSE, "Delay time(ms)"=0.0} ("CAN_Read"), binary string=w1435, error in (no error)=w1436) -> (value=w1434:T19, error out=w1439:errorcluster)  [unwired: 2 in, 1 out]
            n488 = Index Array(array=w1426, index=w1427) -> (element=w1425:refnum<queue>)
            n489 = Unbundle By Name(w1434) -> ("DELAY"=w1432:bool, "Delay time(ms)"=w1431:dbl)
            n490 = To Variant(anything=w1434) -> (Variant=w1440:variant)
            n491 = Bundle By Name(cluster=w1443, "LaunchStep"=TRUE, "Delay"=w1432, "Delay time"=w1431) -> (w1433:T2)
            n492 = call "Enque_Message_FGV.vi"("Priority"=TRUE, "error in (no error)"=w1439, "Message Data"=w1440, "Message"="ConfigRead", "queue IN"=w1425) -> ("error out"=w1442:errorcluster)  [unwired: 6 in]
          }
          frame "PCAN_Write" {
            n493 = Equal?(x=w1447, y="Write_Barcode") -> (x = y?=w1445:bool)
            n494 = Search 1D Array(1D array=w1449, element="PCAN") -> (index of element=w1450:i32)  [unwired: 1 in]
            n495 = case shown="True" w1445 {
              tunnel: [w1472 w1475] -> w1460
              tunnel: w1459 -> [w1466 w1482]
              tunnel: [w1465 w1474] -> w1458
              tunnel: w1453 -> [w1464 w1481]
              tunnel: w1450 -> [w1463 w1479]
              tunnel: w1448 -> [w1462 w1480]
              tunnel: w1444 -> [_ w1478]
              frame False {
                n496 = Unflatten From String(type=T16 {"Scaling Factor"=1, "Physical value"=0.0, "CAN_Frames"={"CAN_ID"=0, "MSGTYPE"=128, "Payload"=[], "Length"=0}, "Offset value"=0.0, "Framing datas"=[], "CAN_Frame Enable"=FALSE, "Add Signal"=FALSE, "Delete Signal"=FALSE, "Signal Values"=[], "Time(ms)"=0.0, "Repetition"=FALSE, "Delay"=FALSE, "Delay time"=0.0} ("CAN_MSGs_Write"), binary string=w1464, error in (no error)=w1466) -> (value=w1465:T16, error out=w1468:errorcluster)  [unwired: 2 in, 1 out]
                n497 = Index Array(array=w1462, index=w1463) -> (element=w1461:refnum<queue>)
                n498 = To Variant(anything=w1465) -> (Variant=w1470:variant)
                n499 = call "Enque_Message_FGV.vi"("Priority"=TRUE, "error in (no error)"=w1468, "Message Data"=w1470, "Message"="ConfigWrite", "queue IN"=w1461) -> ("error out"=w1472:errorcluster)  [unwired: 6 in]
              }
              frame True {
                n500 = Unflatten From String(type=T16 {"Scaling Factor"=1, "Physical value"=0.0, "CAN_Frames"={"CAN_ID"=0, "MSGTYPE"=128, "Payload"=[], "Length"=0}, "Offset value"=0.0, "Framing datas"=[], "CAN_Frame Enable"=FALSE, "Add Signal"=FALSE, "Delete Signal"=FALSE, "Signal Values"=[], "Time(ms)"=0.0, "Repetition"=FALSE, "Delay"=FALSE, "Delay time"=0.0} ("CAN_MSGs_Write"), binary string=w1481, error in (no error)=w1482) -> (value=w1474:T16, error out=w1476:errorcluster)  [unwired: 2 in, 1 out]
                n501 = Index Array(array=w1480, index=w1479) -> (element=w1477:refnum<queue>)
                n502 = Unbundle By Name(w1474) -> ("CAN_Frames.CAN_ID"=w1473:u32)
                n503 = call "Barcode_Write_DTU.vi"("queue IN"=w1477, "error in (no error)"=w1476, "CAN_Frames.CAN_ID"=w1473, "Barcode"=w1478) -> ("error out"=w1475:errorcluster)  [unwired: 7 in]
              }
            }
            n504 = Unbundle By Name(w1458) -> ("Delay"=w1456:bool, "Delay time"=w1455:dbl)
            n505 = Bundle By Name(cluster=w1457, "LaunchStep"=TRUE, "Delay"=w1456, "Delay time"=w1455) -> (w1454:T2)
          }
          frame "Camera" {
            n506 = call "FGV_camera_status.vi"("Enum"=enum16{"Init", "Read", "Write"}."Read") -> ("Read"=w1486:T34)  [unwired: 10 in]
            n507 = Unbundle By Name(w1486) -> ("Free/inuse"=w1485:bool)
            n508 = case shown="False" w1485 {
              tunnel: w1494 -> [w1514 w1537]
              tunnel: w1493 -> [w1513 w1540]
              tunnel: w1492 -> [w1511 _]
              tunnel: [w1509 w1536] -> w1491
              tunnel: [w1506 w1540] -> w1490
              tunnel: w1489 -> [w1502 _]
              tunnel: w1488 -> [_ w1535]
              tunnel: w1484 -> [w1499 _]
              frame False {
                n509 = local read "RX/RY"() -> (w1496:string)
                n510 = Array Size(array=w1502) -> (size(s)=w1501:i32)
                n511 = Unflatten From String(type=T20 {"Trigger"=FALSE, "Prog No."="", "Delay"=FALSE, "Delay time"=0.0, "Storage"="", "Col no."="", "Row no."=""} ("Camera"), binary string=w1511, error in (no error)=w1514) -> (value=w1495:T20, error out=w1512:errorcluster)  [unwired: 2 in, 1 out]
                n512 = Decrement(x=w1501) -> (x-1=w1500:i32)
                n513 = Index Array(array=w1502, index=w1500) -> (element=w1508:refnum<queue>)
                n514 = Unbundle By Name(w1495) -> ("Delay time"=w1505:dbl, "Delay"=w1504:bool, "Trigger"=w1507:bool, "Prog No."=w1497:string)
                n515 = call "RX_RY.vi"("RX/RY"=w1496, "Prg.no"=w1497) -> ()  [unwired: 1 out]
                n516 = Number To Decimal String(number=w1499) -> (decimal integer string=w1498:string)  [unwired: 1 in]
                n517 = case shown="True" w1507 {
                  tunnel: w1512 -> [w1522 w1532]
                  tunnel: [w1524 w1534] -> w1509
                  tunnel: w1508 -> [w1523 w1533]
                  tunnel: w1495 -> [w1519 w1529]
                  tunnel: w1498 -> [w1515 w1526]
                  frame True {
                    n518 = Concatenate Strings("Get_Mode" ("Message"), w1515) -> (w1516:string)
                    n519 = To Variant(anything=w1519) -> (Variant=w1518:variant)
                    n520 = Bundle(cluster=T25 {"Message"="", "Message Data"=variant} ("element"), "Message"=w1516, "Message Data"=w1518) -> (w1520:T25)
                    n521 = Enqueue Element At Opposite End(queue=w1523, element=w1520, error in (no error)=w1522) -> (error out=w1524:errorcluster)  [unwired: 1 in, 2 out]
                  }
                  frame False {
                    n522 = To Variant(anything=w1529) -> (Variant=w1528:variant)
                    n523 = Concatenate Strings("Get_Mode" ("Message"), w1526) -> (w1525:string)
                    n524 = Bundle(cluster=T25 {"Message"="", "Message Data"=variant} ("element"), "Message"=w1525, "Message Data"=w1528) -> (w1530:T25)
                    n525 = Enqueue Element At Opposite End(queue=w1533, element=w1530, error in (no error)=w1532) -> (error out=w1534:errorcluster)  [unwired: 1 in, 2 out]
                  }
                }
                n526 = Bundle By Name(cluster=w1513, "LaunchStep"=TRUE, "Delay"=w1504, "Delay time"=w1505) -> (w1506:T2)
              }
              frame True {
                n527 = call "Test_Enque_Message_FGV.vi"("Priority"=TRUE ("Priority Message? (F)"), "error in (no error)"=w1537, "Message"="LaunchStep", "queue in"=w1535) -> ("error out"=w1536:errorcluster)  [unwired: 7 in]
              }
            }
          }
          frame "MCU_Flashing" {
            n528 = Array Size(array=w1544) -> (size(s)=w1542:i32)
            n529 = Subtract(x=w1542, y=2) -> (x-y=w1541:i32)
            n530 = Index Array(array=w1544, index=w1541) -> (element=w1552:refnum<queue>)
            n531 = Unflatten From String(type=T21 {"Result Path"=path "", "Result"=""} ("MCU Flashing"), binary string=w1555, error in (no error)=w1558) -> (value=w1547:T21, error out=w1556:errorcluster)  [unwired: 2 in, 1 out]
            n532 = Bundle By Name(cluster=w1557, "LaunchStep"=TRUE) -> (w1546:T2)
            n533 = To Variant(anything=w1547) -> (Variant=w1548:variant)
            n534 = Bundle(cluster=T25 {"Message"="", "Message Data"=variant} ("element"), "Message"="Flash", "Message Data"=w1548) -> (w1550:T25)
            n535 = Enqueue Element At Opposite End(queue=w1552, element=w1550, error in (no error)=w1556) -> (error out=w1553:errorcluster)  [unwired: 1 in, 2 out]
          }
          frame "Noeway_Flashing" {
            n536 = Array Size(array=w1561) -> (size(s)=w1559:i32)
            n537 = Unflatten From String(type=T22 {"Neoway_Firmware"=path "", "RESULT STRING"="", "Delay"=FALSE, "Delay time"=0.0} ("Noeway_Flashing"), binary string=w1574, error in (no error)=w1577) -> (value=w1564:T22, error out=w1575:errorcluster)  [unwired: 2 in, 1 out]
            n538 = Decrement(x=w1559) -> (x-1=w1560:i32)
            n539 = Index Array(array=w1561, index=w1560) -> (element=w1568:refnum<queue>)
            n540 = To Variant(anything=w1564) -> (Variant=w1563:variant)
            n541 = Unbundle By Name(w1564) -> ("Delay"=w1571:bool, "Delay time"=w1570:dbl)
            n542 = Bundle(cluster=T25 {"Message"="", "Message Data"=variant} ("element"), "Message"="Flash_replacing", "Message Data"=w1563) -> (w1566:T25)
            n543 = Enqueue Element At Opposite End(queue=w1568, element=w1566, error in (no error)=w1575) -> (error out=w1569:errorcluster)  [unwired: 1 in, 2 out]
            n544 = Bundle By Name(cluster=w1576, "Delay"=w1571, "Delay time"=w1570, "LaunchStep"=TRUE) -> (w1572:T2)
          }
          frame "SSL_Certification" {
            (unwired) "SSL_Certification"
            n545 = Unflatten From String(type=T23 {"SSL_EXE"=path "", "RESULT STRING"="", "Delay"=FALSE, "Delay time"=0.0} ("SSL"), binary string=w1587, error in (no error)=w1590) -> (value=w1580:T23, error out=w1588:errorcluster)  [unwired: 2 in, 1 out]
            n546 = Unbundle By Name(w1580) -> ("Delay"=w1584:bool, "Delay time"=w1583:dbl)
            n547 = To Variant(anything=w1580) -> (Variant=w1579:variant)
            n548 = disable-structure shown="Enabled" {
              disable-tunnel: w1588 -> [w1598 w1599]
              disable-tunnel: w1582 -> [w1597 _]
              disable-tunnel: [w1596 w1599] -> w1581
              disable-tunnel: w1579 -> [w1591 _]
              frame Disabled {
                n549 = Index Array(array=w1597) -> (element=w1595:refnum<queue>)  [unwired: 1 in]
                n550 = Bundle(cluster=T25 {"Message"="", "Message Data"=variant} ("element"), "Message"="", "Message Data"=w1591) -> (w1593:T25)
                n551 = Enqueue Element At Opposite End(queue=w1595, element=w1593, error in (no error)=w1598) -> (error out=w1596:errorcluster)  [unwired: 1 in, 2 out]
              }
              frame Enabled {
              }
            }
            n552 = Bundle By Name(cluster=w1589, "LaunchStep"=TRUE, "Delay"=w1584, "Delay time"=w1583) -> (w1585:T2)
          }
        }
      }
      frame "Waittime" {
        n553 = Unbundle By Name(w1608) -> ("Delay time"=w1604:dbl, "Delay"=w1602:bool, "LaunchStep"=w1603:bool)
        n554 = case shown="True" w1602 {
          tunnel: [u32 1000 ("milliseconds to wait") w1613] -> w1606
          tunnel: w1604 -> [_ w1612]
          frame False {
          }
          frame True {
            n555 = To Unsigned Long Integer(number=w1612) -> (unsigned 32bit integer=w1613:u32)
          }
        }
        n556 = Select(t=w1606, s=w1603, f=u32 10) -> (s? t:f=w1607:u32)
        n557 = flat-sequence {
          tunnel: w1610 -> [w1615]
          tunnel: w1607 -> [w1614]
          tunnel: [w1615] -> w1601
          tunnel: [w1614] -> w1600
          tunnel: [w1619] -> w1609
          tunnel: w1601 -> [w1620]
          tunnel: w1600 -> [w1617]
          frame #0 {
          }
          frame #1 {
            n558 = Divide(x=w1617, y=u32 1000) -> (x/y=w1618:dbl)
            n559 = call "Time Delay2"("error in (no error)"=w1620, "Delay Time (s)"=w1618) -> ("error out"=w1619:errorcluster)  [unwired: 9 in]
          }
        }
      }
      frame "GetData" {
        (unwired) StepType."RELAY_CHANNEL_WRITE" ("Type")
        n560 = Unbundle By Name(w1627) -> ("RX/RY"=w1621:string, "EQUP LIST"=w1622:string[], "Array_Q"=w1623:refnum<queue>[], "Data Path"=w1624:path, "Barcode"=w1628:string, "UI Data.ScriptDetails.Script Name"=w1634:string, "UI Data.ScriptDetails.Steps"=w1643:T5[], "Stepno."=w1644:u64, "Message Data"=w1640:variant, "DUT"=w1625:i32)
        n561 = Index Array(array=w1643, index=w1644) -> (element=w1642:T5)
        n562 = Number To Decimal String(number=w1625) -> (decimal integer string=w1626:string)  [unwired: 1 in]
        n563 = Unbundle By Name(w1642) -> ("StepName"=w1633:string, "StepDetails"=w1639:string, "Type"=w1641:T6)
        n564 = case shown="\"READ_DATA\"" w1641 {
          tunnel: w1645 -> [w1651 w1670 w1689 w1699 w1828 w1834 w1840 w1846 w1852 w2306 w2318]
          tunnel: [w1651 w1661 w1681 w1696 w1828 w1834 w1840 w1846 w1851 w2306 w2327] -> w1637
          tunnel: w1640 -> [_ w1664 w1682 _ _ _ _ _ w1853 _ w2315]
          tunnel: w1639 -> [_ w1660 w1680 w1701 _ _ _ _ w1855 _ w2314]
          tunnel: w1627 -> [w1650 w1669 w1687 w1706 w1827 w1833 w1839 w1845 w1849 w2304 w2325]
          tunnel: [w1649 w1668 w1686 w1705 w1826 w1832 w1838 w1844 w1854 w2303 w2324] -> w1635
          tunnel: w1634 -> [w1648 w1667 w1685 w1704 w1825 w1831 w1837 w1843 w1857 w2302 w2323]
          tunnel: w1633 -> [w1647 w1666 w1684 w1703 w1824 w1830 w1836 w1842 w1856 w2301 w2322]
          tunnel: w1627 -> [_ _ _ _ _ _ _ _ w1850 _ _]
          tunnel: w1628 -> [_ _ _ w1695 _ _ _ _ _ _ w2310]
          tunnel: w1627 -> [_ _ _ _ _ _ _ _ _ _ w2309]
          tunnel: w1626 -> [_ _ _ w1698 _ _ _ _ _ _ w2308]
          tunnel: w1625 -> [_ _ _ _ _ _ _ _ w1848 _ w2307]
          tunnel: w1624 -> [_ _ _ w1693 _ _ _ _ _ _ _]
          tunnel: w1623 -> [_ _ _ w1691 _ _ _ _ _ _ _]
          tunnel: w1622 -> [_ _ _ w1690 _ _ _ _ _ _ _]
          tunnel: w1621 -> [_ _ _ _ _ _ _ _ w1847 _ _]
          frame "PS_WRITE", Default {
            w1646 = ""
            n565 = Bundle By Name(cluster=w1650, "UNIT"=w1646, "USL"=w1646, "LSL"=w1646, "Pass/Fail"=w1646, "Actual"=w1646, "Scriptname"=w1648, "Stepname"=w1647) -> (w1649:T2)
          }
          frame "MCU_Flashing" {
            w1662 = ""
            n566 = Variant To Data(error in=w1670, type="", Variant=w1664) -> (data=w1656:string, error out=w1665:errorcluster)
            n567 = Unflatten From String(type=T21 {"Result Path"=path "", "Result"=""} ("MCU Flashing"), binary string=w1660, error in (no error)=w1665) -> (value=w1658:T21, error out=w1661:errorcluster)  [unwired: 2 in, 1 out]
            n568 = Unbundle By Name(w1658) -> ("Result"=w1657:string)
            n569 = Equal?(x=w1657, y=w1656) -> (x = y?=w1652:bool)
            n570 = Select(t="Pass", s=w1652, f="Fail") -> (s? t:f=w1653:string)
            n571 = Bundle By Name(cluster=w1669, "UNIT"=w1662, "USL"=w1662, "LSL"=w1662, "Pass/Fail"=w1653, "Actual"=w1656, "Scriptname"=w1667, "Stepname"=w1666, "Result"=w1652) -> (w1668:T2)
          }
          frame "Noeway_Flashing" {
            w1688 = ""
            n572 = Variant To Data(error in=w1689, type="", Variant=w1682) -> (data=w1675:string, error out=w1683:errorcluster)
            n573 = Unflatten From String(type=T22 {"Neoway_Firmware"=path "", "RESULT STRING"="", "Delay"=FALSE, "Delay time"=0.0} ("Noeway_Flashing"), binary string=w1680, error in (no error)=w1683) -> (value=w1677:T22, error out=w1681:errorcluster)  [unwired: 2 in, 1 out]
            n574 = Unbundle By Name(w1677) -> ("RESULT STRING"=w1676:string)
            n575 = Equal?(x=w1676, y=w1675) -> (x = y?=w1671:bool)
            n576 = Select(t="Pass", s=w1671, f="Fail") -> (s? t:f=w1672:string)
            n577 = Bundle By Name(cluster=w1687, "UNIT"=w1688, "USL"=w1688, "LSL"=w1688, "Pass/Fail"=w1672, "Actual"=w1675, "Scriptname"=w1685, "Stepname"=w1684, "Result"=w1671) -> (w1686:T2)
          }
          frame "SSL_Certification" {
            w1702 = ""
            n578 = local read "EOL/FCT"() -> (w1692:bool)
            n579 = case shown="True" w1692 {
              tunnel: w1701 -> [w1731 _]
              tunnel: [w1728 w1782] -> w1700
              tunnel: w1699 -> [w1727 w1789]
              tunnel: w1698 -> [w1725 w1786]
              tunnel: [w1718 w1780] -> w1697
              tunnel: [w1711 w1783] -> w1696
              tunnel: w1695 -> [w1709 w1779]
              tunnel: [w1708 w1781] -> w1694
              tunnel: w1693 -> [w1707 _]
              tunnel: w1691 -> [_ w1791]
              tunnel: w1690 -> [_ w1792]
              frame False {
                # "OKAY,River"
                n580 = call "SSL_Certification.vi"("error in (no error)"=w1727, "DUT"=w1725) -> ("error in (out)"=w1726:errorcluster, "Result"=w1724:string)  [unwired: 8 in]
                n581 = Spreadsheet String To Array(delimiter (Tab)=",", format string="%s", spreadsheet string=w1724, array type (2D Dbl)=string[] []) -> (array=w1720:string[])
                n582 = Index Array(array=w1720) -> (element #1=w1718:string, element #2=w1716:string)  [unwired: 2 in]
                n583 = Unflatten From String(type=T23 {"SSL_EXE"=path "", "RESULT STRING"="", "Delay"=FALSE, "Delay time"=0.0} ("SSL"), binary string=w1731, error in (no error)=w1726) -> (value=w1732:T23, error out=w1712:errorcluster)  [unwired: 2 in, 1 out]
                n584 = Equal?(x=w1716, y="River") -> (x = y?=w1715:bool)
                n585 = Unbundle By Name(w1732) -> ("RESULT STRING"=w1719:string)
                n586 = Select(t="RX", s=w1715, f="RY") -> (s? t:f=w1710:string)
                n587 = Equal?(x=w1718, y=w1719) -> (x = y?=w1708:bool)
                n588 = Select(t="Pass", s=w1708, f="Fail") -> (s? t:f=w1728:string)
                n589 = case shown="True" w1708 {
                  tunnel: w1712 -> [w1734 w1755]
                  tunnel: [w1734 w1749] -> w1711
                  tunnel: w1710 -> [_ w1738]
                  tunnel: w1709 -> [_ w1739]
                  tunnel: w1707 -> [_ w1746]
                  frame False {
                  }
                  frame True {
                    n590 = Build Path(base path=w1746, name or relative path="SSL_log.csv") -> (appended path=w1741:path)
                    n591 = Open/Create/Replace File(file path (use dialog)=w1741, error in=w1755, operation (0:open)=T37."open or create") -> (error out=w1744:errorcluster)  [unwired: 3 in, 2 out]
                    n592 = Build Array(w1739, w1738) -> (w1737:string[])
                    n593 = call-poly <vilib>:"Write Delimited Spreadsheet.vi"("file path (dialog if empty)"=w1741, "format (%s)"="%s" ("format (%.3f)"), "1D data"=w1737, "append to file? (new file:F)"=TRUE, "error in (no error)"=w1744, "delimiter (\\t)"="," ("delimiter (\\t)")) -> ("error out"=w1742:errorcluster)  [unwired: 8 in, 1 out]
                    n594 = call "Get_filelist.vi"("error in (no error)"=w1742) -> ("error out"=w1754:errorcluster, "Files"=w1752:string[])  [unwired: 9 in]
                    n595 = Concatenate Strings("SSL_Check" ("string"), ".csv" ("string")) -> (w1751:string)
                    n596 = Search 1D Array(1D array=w1752, element=w1751) -> (index of element=w1750:i32)  [unwired: 1 in]
                    n597 = Less Than 0?(x=w1750) -> (x < 0?=w1748:bool)
                    n598 = case shown="True" w1748 {
                      tunnel: w1754 -> [w1759 w1767]
                      tunnel: [w1758 w1765] -> w1749
                      tunnel: w1738 -> [w1756 w1762]
                      tunnel: w1739 -> [w1757 w1763]
                      frame False {
                        n599 = call "ReadBuffer.vi"("error in (no error)"=w1759, "Combo Box"="append", "ServerConfig"=w1756, "Barcode"=w1757) -> ("error out"=w1758:errorcluster)  [unwired: 7 in]
                      }
                      frame True {
                        n600 = call "PutFile.vi"("error in (no error)"=w1767) -> ("error out"=w1766:errorcluster)  [unwired: 9 in, 1 out]
                        n601 = call <vilib>:"Clear Errors.vi"("error in (no error)"=w1766) -> ("error out"=w1761:errorcluster)  [unwired: 5 in, 1 out]
                        n602 = call "ReadBuffer.vi"("error in (no error)"=w1761, "Combo Box"="append", "ServerConfig"=w1762, "Barcode"=w1763) -> ("error out"=w1765:errorcluster)  [unwired: 7 in]
                      }
                    }
                  }
                }
              }
              frame True {
                n603 = String Subset(string=w1779, offset (0)=5, length (rest)=1 ("length (rest)")) -> (substring=w1776:string)
                n604 = Equal?(x=w1776, y="Y") -> (x = y?=w1774:bool)
                n605 = Search 1D Array(1D array=w1792, element="PCAN") -> (index of element=w1790:i32)  [unwired: 1 in]
                n606 = Select(t="RY", s=w1774, f="RX") -> (s? t:f=w1771:string)
                n607 = flat-sequence {
                  tunnel: w1791 -> [w1799]
                  tunnel: w1790 -> [w1798]
                  tunnel: w1789 -> [w1797]
                  tunnel: [w1796] -> w1788
                  tunnel: w1786 -> [w1795]
                  tunnel: [w1795] -> w1785
                  tunnel: w1771 -> [w1794]
                  tunnel: [w1794] -> w1769
                  tunnel: w1788 -> [w1807]
                  tunnel: [w1806] -> w1787
                  tunnel: w1785 -> [w1805]
                  tunnel: [w1805] -> w1784
                  tunnel: [w1804] -> w1770
                  tunnel: w1769 -> [w1804]
                  tunnel: ["New/Old_Slot"] -> w1768
                  tunnel: [w1820] -> w1783
                  tunnel: w1787 -> [w1821]
                  tunnel: w1784 -> [w1822]
                  tunnel: [w1814] -> w1782
                  tunnel: [w1813] -> w1781
                  tunnel: [w1810] -> w1780
                  tunnel: w1770 -> [w1809]
                  tunnel: w1768 -> [w1808]
                  frame #0 {
                    n608 = Index Array(array=w1799, index=w1798) -> (element=w1800:refnum<queue>)
                    n609 = call "Enque_Message_FGV.vi"("Priority"=TRUE, "error in (no error)"=w1797, "Message"="Uninit_PCAN", "queue IN"=w1800) -> ("error out"=w1796:errorcluster)  [unwired: 7 in]
                  }
                  frame #1 {
                    n610 = call "Time Delay3"("error in (no error)"=w1807) -> ("error out"=w1806:errorcluster)  [unwired: 10 in]
                  }
                  frame #2 {
                    n611 = call "AWSEXE.vi"("error in (no error)"=w1821, "New/Old(T)"=w1808, "RX/RY"=w1809, "DUT"=w1822) -> ("error in (out)"=w1820:errorcluster, "Result"=w1819:string)  [unwired: 6 in]
                    n612 = To Lower Case(string=w1819) -> (all lower case string=w1812:string)
                    n613 = Match Pattern(string=w1812, regular expression="success") -> (offset past match=w1815:i32)  [unwired: 1 in, 3 out]
                    n614 = Greater Or Equal To 0?(x=w1815) -> (x >= 0?=w1813:bool)
                    n615 = Match Pattern(string=w1812, regular expression=": ") -> (after substring=w1810:string)  [unwired: 1 in, 3 out]
                    n616 = Select(t="Pass", s=w1813, f="Fail") -> (s? t:f=w1814:string)
                  }
                }
              }
            }
            n617 = Bundle By Name(cluster=w1706, "UNIT"=w1702, "USL"=w1702, "LSL"=w1702, "Pass/Fail"=w1700, "Actual"=w1697, "Scriptname"=w1704, "Stepname"=w1703, "Result"=w1694) -> (w1705:T2)
          }
          frame "RELAY_CHANNEL_WRITE" {
            w1823 = ""
            n618 = Bundle By Name(cluster=w1827, "UNIT"=w1823, "USL"=w1823, "LSL"=w1823, "Pass/Fail"=w1823, "Actual"=w1823, "Scriptname"=w1825, "Stepname"=w1824) -> (w1826:T2)
          }
          frame "DMM_CONFIG" {
            w1829 = ""
            n619 = Bundle By Name(cluster=w1833, "USL"=w1829, "UNIT"=w1829, "LSL"=w1829, "Pass/Fail"=w1829, "Actual"=w1829, "Scriptname"=w1831, "Stepname"=w1830) -> (w1832:T2)
          }
          frame "DAQ_CONFIG" {
            w1835 = ""
            n620 = Bundle By Name(cluster=w1839, "USL"=w1835, "UNIT"=w1835, "LSL"=w1835, "Pass/Fail"=w1835, "Actual"=w1835, "Scriptname"=w1837, "Stepname"=w1836) -> (w1838:T2)
          }
          frame "PCAN_Write" {
            w1841 = ""
            n621 = Bundle By Name(cluster=w1845, "USL"=w1841, "UNIT"=w1841, "LSL"=w1841, "Pass/Fail"=w1841, "Actual"=w1841, "Scriptname"=w1843, "Stepname"=w1842) -> (w1844:T2)
          }
          frame "PCAN_Read" {
            # "BDDKSC003895"
            n622 = Variant To Data(error in=w1852, type=T19 {"Database"="", "Signal"="", "BYTES"=[], "ReadPayload"=[], "String_Data"="", "ReadValue"=0.0, "CANID"=0, "SERVICE ID"=0, "SUB-SERVICE ID"=0, "DELAY "=FALSE, "Delay time(ms)"=0.0} ("CAN_Read"), Variant=w1853) -> (data=w1863:T19, error out=w1862:errorcluster)
            n623 = Unbundle By Name(w1863) -> ("ReadValue"=w1859:dbl, "ReadPayload"=w1860:u8[], "String_Data"=w1861:string)
            n624 = case shown="\"\"" w1861 {
              tunnel: w1862 -> [w1884 w1919 w2064 w2216 w2241 w2252]
              tunnel: [w1881 w1919 w2063 w2213 w2238 w2249] -> w1851
              tunnel: w1860 -> [w1875 w1893 w2056 _ w2228 w2246]
              tunnel: w1849 -> [w1883 w1923 _ w2215 w2240 w2251]
              tunnel: [w1882 w1922 w2066 w2214 w2239 w2250] -> w1854
              tunnel: w1855 -> [w1880 _ w2062 w2212 w2237 w2248]
              tunnel: w1857 -> [w1878 w1920 w2060 w2210 w2235 w2247]
              tunnel: w1856 -> [w1877 w1921 w2061 w2209 w2234 w2245]
              tunnel: w1859 -> [_ _ _ w2204 _ _]
              tunnel: w1850 -> [_ _ w2047 _ _ _]
              tunnel: w1848 -> [_ _ w2043 _ _ w2242]
              tunnel: w1847 -> [_ _ w2041 _ _ _]
              frame "Version", Default {
                w1864 = "" ("Expected_Vlu")
                n625 = Unflatten From String(type=T19 {"Database"="", "Signal"="", "BYTES"=[], "ReadPayload"=[], "String_Data"="", "ReadValue"=0.0, "CANID"=0, "SERVICE ID"=0, "SUB-SERVICE ID"=0, "DELAY "=FALSE, "Delay time(ms)"=0.0} ("CAN_Read"), binary string=w1880, error in (no error)=w1884) -> (value=w1879:T19, error out=w1881:errorcluster)  [unwired: 2 in, 1 out]
                n626 = Unbundle By Name(w1879) -> ("ReadPayload"=w1867:u8[], "BYTES"=w1876:u32[])
                n627 = call "Payload_Define.vi"("Hex(T)"=FALSE, "Payload"=w1875, "Bytes"=w1876) -> ("Payload String"=w1870:string, "Read payload"=w1874:u8[])  [unwired: 7 in]
                n628 = Equal?(x=w1867, y=w1874) -> (x = y?=w1873:bool[])
                n629 = And Array Elements(Boolean array=w1873) -> (logical AND=w1868:bool)
                n630 = Select(t="Pass", s=w1868, f="Fail") -> (s? t:f=w1871:string)
                n631 = Bundle By Name(cluster=w1883, "LSL"=w1864, "USL"=w1864, "UNIT"=w1864, "Expected_Value"=w1864, "Scriptname"=w1878, "Stepname"=w1877, "Pass/Fail"=w1871, "Actual"=w1870, "Result"=w1868) -> (w1882:T2)
              }
              frame "Barcode" {
                w1894 = 6 ("offset (0)")
                w1913 = "" ("LSL")
                n632 = Byte Array To String(unsigned byte array=w1893) -> (string=w1918:string)
                n633 = String Subset(string=w1918, offset (0)=0, length (rest)=12 ("length (rest)")) -> (substring=w1890:string)
                n634 = String Length(string=w1890) -> (length=w1907:i32)
                n635 = Empty String/Path?(string/path=w1890) -> (empty?=w1908:bool)
                n636 = String Subset(string=w1890, offset (0)=0, length (rest)=6 ("length (rest)")) -> (substring=w1901:string)
                n637 = String Subset(string=w1890, offset (0)=w1894, length (rest)=w1894) -> (substring=w1896:string)
                n638 = Index Array(array=w1893, index=0) -> (element=w1909:u8)
                n639 = Equal?(x=w1907, y=12) -> (x = y?=w1899:bool)
                n640 = Not Equal To 0?(x=w1909) -> (x != 0?=w1891:bool)
                n641 = String Length(string=w1901) -> (length=w1902:i32)
                n642 = String Length(string=w1896) -> (length=w1897:i32)
                n643 = Not(x=w1908) -> (.not. x?=w1892:bool)
                n644 = Equal?(x=w1902, y=6) -> (x = y?=w1900:bool)
                n645 = Equal?(x=w1897, y=6) -> (x = y?=w1895:bool)
                n646 = Compound Arithmetic op=AND(w1899, w1891, w1892, w1900, w1895) -> (w1886:bool)
                "result" <- w1886
                n647 = xnode "Match Regular Expression"("input string"=w1890, "regular expression"="[^a-zA-Z0-9]") -> ("offset past match"=w1888:i32)  [unwired: 4 in, 4 out]
                n648 = Less Than 0?(x=w1888) -> (x < 0?=w1887:bool)
                n649 = And(x=w1886, y=w1887) -> (x .and. y?=w1885:bool)
                n650 = Select(t="Pass" ("f"), s=w1885, f="Fail") -> (s? t:f=w1915:string)
                n651 = Bundle By Name(cluster=w1923, "LSL"=w1913, "USL"=w1913, "UNIT"=w1913, "Pass/Fail"=w1915, "Expected_Value"="" ("Expected_Vlu"), "Stepname"=w1921, "Scriptname"=w1920, "Actual"=w1890, "Barcode"=w1890) -> (w1922:T2)
              }
              frame "" {
                w2045 = "" ("Expected_Value")
                n652 = Unflatten From String(type=T19 {"Database"="", "Signal"="", "BYTES"=[], "ReadPayload"=[], "String_Data"="", "ReadValue"=0.0, "CANID"=0, "SERVICE ID"=0, "SUB-SERVICE ID"=0, "DELAY "=FALSE, "Delay time(ms)"=0.0} ("CAN_Read"), binary string=w2062, error in (no error)=w2064) -> (value=w2065:T19, error out=w2063:errorcluster)  [unwired: 2 in, 1 out]
                n653 = Unbundle By Name(w2065) -> ("CANID"=w2044:u32, "ReadValue"=w2049:dbl, "SERVICE ID"=w2058:u32, "SUB-SERVICE ID"=w2057:u32, "ReadPayload"=w2055:u8[], "BYTES"=w2054:u32[])
                n654 = case shown="26D" w2044 {
                  tunnel: w2058 -> [_ _ w2102]
                  tunnel: w2057 -> [_ _ w2101]
                  tunnel: w2056 -> [w2075 w2083 w2100]
                  tunnel: w2055 -> [_ _ w2099]
                  tunnel: w2054 -> [w2074 _ w2098]
                  tunnel: [w2071 w2079 w2097] -> w2050
                  tunnel: w2049 -> [_ _ w2096]
                  tunnel: [w2069 w2078 w2095] -> w2048
                  tunnel: w2047 -> [w2077 w2084 w2094]
                  tunnel: [w2077 w2084 w2093] -> w2046
                  tunnel: w2043 -> [_ _ w2092]
                  tunnel: [w2067 w2078 w2091] -> w2042
                  tunnel: w2041 -> [w2067 _ w2091]
                  frame 621 {
                    n655 = call "Payload_Define.vi"("Hex(T)"=FALSE, "Payload"=w2075, "Bytes"=w2074) -> ("Read payload"=w2073:u8[])  [unwired: 7 in, 1 out]
                    n656 = Reverse 1D Array(array=w2073) -> (reversed array=w2068:u8[])
                    n657 = Type Cast(type=u32 0, x=w2068) -> (*(type *) &x=w2070:u32)
                    n658 = Greater Than 0?(x=w2070) -> (x > 0?=w2071:bool)
                    n659 = Number To Decimal String(number=w2070) -> (decimal integer string=w2069:string)  [unwired: 1 in]
                  }
                  frame 1833 {
                    n660 = Index Array(array=w2083, index=3) -> (element=w2081:u8)
                    n661 = Number To Hexadecimal String(2:w2081) -> (0:w2080:string)  [unwired: 1 in]
                    n662 = case shown="\"AA\"" w2080 {
                      tunnel: ["" "RX" "RY"] -> w2078
                      tunnel: [FALSE ("PASS(T)") TRUE ("PASS(T)") TRUE ("PASS(T)")] -> w2079
                      frame "False", Default {
                      }
                      frame "AA" {
                      }
                      frame "55" {
                      }
                    }
                    "RX/RY" <- w2078
                  }
                  frame 1, Default {
                    n663 = case shown="62" w2102 {
                      tunnel: w2101 -> [w2110 w2134 _ _]
                      tunnel: w2100 -> [w2109 w2133 w2188 w2197]
                      tunnel: w2099 -> [w2108 w2131 _ w2194]
                      tunnel: w2098 -> [w2107 w2132 _ w2196]
                      tunnel: [w2106 w2129 w2186 w2192] -> w2097
                      tunnel: w2096 -> [w2105 _ _ _]
                      tunnel: [w2104 w2130 w2187 w2191] -> w2095
                      tunnel: w2094 -> [w2103 w2128 w2189 w2198]
                      tunnel: [w2103 w2127 w2189 w2198] -> w2093
                      tunnel: w2092 -> [_ w2126 _ _]
                      frame 111, Default {
                        n664 = case shown="0, Default" w2110 {
                          tunnel: w2109 -> [w2117 w2124]
                          tunnel: w2108 -> [w2115 _]
                          tunnel: w2107 -> [w2118 _]
                          tunnel: [w2113 w2125] -> w2106
                          tunnel: w2105 -> [_ w2123]
                          tunnel: [w2112 w2121] -> w2104
                          frame 0, Default {
                            n665 = call "Payload_Define.vi"("Hex(T)"=TRUE, "Payload"=w2117, "Bytes"=w2118) -> ("Payload String"=w2112:string, "Read payload"=w2116:u8[])  [unwired: 7 in]
                            n666 = Equal?(x=w2115, y=w2116) -> (x = y?=w2114:bool[])
                            n667 = And Array Elements(Boolean array=w2114) -> (logical AND=w2113:bool)
                          }
                          frame 2 {
                            n668 = To Unsigned Byte Integer(number=w2123) -> (unsigned 8bit integer=w2122:u8)
                            n669 = Array Subset(array=w2124, index=2) -> (w2120:u8[])  [unwired: 1 in]
                            n670 = call "CSQ_Check.vi"("y"=w2122, "CSQ"=w2120) -> ("P/F"=w2125:bool, "Fail count"=w2121:string)  [unwired: 8 in]
                          }
                        }
                      }
                      frame 98 {
                        n671 = case shown="5" w2134 {
                          tunnel: w2133 -> [w2140 w2146 w2157 w2179 w2183]
                          tunnel: w2132 -> [w2141 _ _ _ _]
                          tunnel: w2131 -> [w2139 _ _ _ _]
                          tunnel: [w2138 w2144 w2160 w2176 w2182] -> w2130
                          tunnel: [w2137 w2145 w2158 TRUE ("PASS(T)") w2180] -> w2129
                          tunnel: w2128 -> [w2136 w2147 w2162 w2178 w2185]
                          tunnel: [w2136 w2147 w2161 w2177 w2184] -> w2127
                          tunnel: w2126 -> [_ _ w2159 _ _]
                          frame 1, Default {
                            n672 = call "Payload_Define.vi"("Hex(T)"=TRUE, "Payload"=w2140, "Bytes"=w2141) -> ("Payload String"=w2138:string, "Read payload"=w2143:u8[])  [unwired: 7 in]
                            n673 = Equal?(x=w2139, y=w2143) -> (x = y?=w2142:bool[])
                            n674 = And Array Elements(Boolean array=w2142) -> (logical AND=w2137:bool)
                          }
                          frame 4 {
                            # "GPS"
                            n675 = disable-structure shown="Enabled" {
                              disable-tunnel: w2146 -> [w2150 _]
                              disable-tunnel: [w2149 TRUE ("PASS(T)")] -> w2145
                              disable-tunnel: [w2148 _] -> w2144
                              frame Enabled {
                                n676 = call "GPS_parse.vi"("GPS_Payload"=w2150) -> ("PASS(T)"=w2149:bool, "Result"=w2148:string)  [unwired: 8 in, 1 out]
                              }
                              frame Disabled {
                              }
                            }
                          }
                          frame 3 {
                            # "MACID"
                            n677 = for {
                              tunnel: w2157 -> [w2173] mode=indexing
                              shift-right: [w2170] -> w2154
                              shift-left: _ -> [w2169]
                              n678 = Number To Hexadecimal String(2:w2173) -> (0:w2172:string)  [unwired: 1 in]
                              n679 = Concatenate Strings(w2169, w2172, ":" ("string")) -> (w2170:string)
                            }
                            n680 = String Subset(string=w2154, length (rest)=17 ("length (rest)")) -> (substring=w2152:string)  [unwired: 1 in]
                            n681 = disable-structure shown="Enabled" {
                              disable-tunnel: w2159 -> [w2165 _]
                              disable-tunnel: [w2164 w2166] -> w2158
                              disable-tunnel: w2152 -> [w2163 w2168]
                              frame Disabled {
                                n682 = call "BLE_Module_EOL.vi"("DUT"=w2165, "DUTBLEMACAddress"=w2163) -> ("PASS"=w2164:bool)  [unwired: 5 in, 3 out]
                              }
                              frame Enabled {
                                n683 = Empty String/Path?(string/path=w2168) -> (empty?=w2167:bool)
                                n684 = Not(x=w2167) -> (.not. x?=w2166:bool)
                              }
                            }
                            n685 = Bundle By Name(cluster=w2162, "MACID"=w2152) -> (w2161:T2)
                            n686 = Select(t="CONNECTED", s=w2158, f="NOT_CONNECTED") -> (s? t:f=w2160:string)
                          }
                          frame 5 {
                            # "IMEI"
                            n687 = Byte Array To String(unsigned byte array=w2179) -> (string=w2176:string)
                            n688 = Empty String/Path?(string/path=w2176) -> (empty?=w2175:bool)
                            n689 = Bundle By Name(cluster=w2178, "IMEI"=w2176) -> (w2177:T2)
                            n690 = Not(x=w2175) -> ()  [unwired: 1 out]
                          }
                          frame 6 {
                            # "ICCID"
                            n691 = Byte Array To String(unsigned byte array=w2183) -> (string=w2182:string)
                            n692 = Empty String/Path?(string/path=w2182) -> (empty?=w2181:bool)
                            n693 = Bundle By Name(cluster=w2185, "ICCID"=w2182) -> (w2184:T2)
                            n694 = Not(x=w2181) -> (.not. x?=w2180:bool)
                          }
                        }
                      }
                      frame 99 {
                        n695 = Byte Array To String(unsigned byte array=w2188) -> (string=w2187:string)
                        n696 = Empty String/Path?(string/path=w2187) -> (empty?=w2186:bool)
                      }
                      frame 191 {
                        n697 = call "Payload_Define.vi"("Hex(T)"=TRUE, "Payload"=w2197, "Bytes"=w2196) -> ("Payload String"=w2191:string, "Read payload"=w2195:u8[])  [unwired: 7 in]
                        n698 = Equal?(x=w2194, y=w2195) -> (x = y?=w2193:bool[])
                        n699 = And Array Elements(Boolean array=w2193) -> (logical AND=w2192:bool)
                      }
                    }
                  }
                }
                n700 = Select(t="Pass", s=w2050, f="Fail") -> (s? t:f=w2051:string)
                n701 = Bundle By Name(cluster=w2046, "RX/RY"=w2042, "LSL"=w2045, "USL"=w2045, "UNIT"=w2045, "Expected_Value"=w2045, "Stepname"=w2061, "Scriptname"=w2060, "Pass/Fail"=w2051, "Result"=w2050, "Actual"=w2048) -> (w2066:T2)
              }
              frame "Value" {
                w2199 = ""
                n702 = Unflatten From String(type=T19 {"Database"="", "Signal"="", "BYTES"=[], "ReadPayload"=[], "String_Data"="", "ReadValue"=0.0, "CANID"=0, "SERVICE ID"=0, "SUB-SERVICE ID"=0, "DELAY "=FALSE, "Delay time(ms)"=0.0} ("CAN_Read"), binary string=w2212, error in (no error)=w2216) -> (value=w2211:T19, error out=w2213:errorcluster)  [unwired: 2 in, 1 out]
                n703 = Unbundle By Name(w2211) -> ("ReadValue"=w2202:dbl)
                n704 = Equal?(x=w2202, y=w2204) -> (x = y?=w2205:bool)
                n705 = Number To Decimal String(number=w2202) -> (decimal integer string=w2201:string)  [unwired: 1 in]
                n706 = Number To Decimal String(number=w2204) -> (decimal integer string=w2203:string)  [unwired: 1 in]
                n707 = Select(t="Pass", s=w2205, f="Fail") -> (s? t:f=w2207:string)
                n708 = Bundle By Name(cluster=w2215, "LSL"=w2199, "USL"=w2199, "UNIT"=w2199, "Expected_Value"=w2201, "Scriptname"=w2210, "Stepname"=w2209, "Pass/Fail"=w2207, "Actual"=w2203, "Result"=w2205) -> (w2214:T2)
              }
              frame "Temp" {
                w2222 = TRUE ("s")
                w2217 = "" ("Expected_Value")
                n709 = Unflatten From String(type=T19 {"Database"="", "Signal"="", "BYTES"=[], "ReadPayload"=[], "String_Data"="", "ReadValue"=0.0, "CANID"=0, "SERVICE ID"=0, "SUB-SERVICE ID"=0, "DELAY "=FALSE, "Delay time(ms)"=0.0} ("CAN_Read"), binary string=w2237, error in (no error)=w2241) -> (value=w2236:T19, error out=w2238:errorcluster)  [unwired: 2 in, 1 out]
                n710 = Unbundle By Name(w2236) -> ("BYTES"=w2229:u32[])
                n711 = call "Payload_Define.vi"("Hex(T)"=FALSE, "Payload"=w2228, "Bytes"=w2229) -> ("Read payload"=w2223:u8[])  [unwired: 7 in, 1 out]
                n712 = Index Array(array=w2223) -> (element #1=w2226:u8, element #2=w2227:u8)  [unwired: 2 in]
                n713 = Join Numbers(hi=w2227, lo=w2226) -> ((hi.lo)=w2225:u16)
                n714 = Divide(x=w2225, y=u16 100) -> (x/y=w2221:dbl)
                n715 = Number To Fractional String(number=w2221, precision (6)=i16 2) -> (F-format string=w2219:string)  [unwired: 2 in]
                n716 = Select(t="Pass", s=w2222, f="Fail") -> (s? t:f=w2232:string)
                n717 = Bundle By Name(cluster=w2240, "LSL"=w2217, "USL"=w2217, "UNIT"=w2217, "Expected_Value"=w2217, "Scriptname"=w2235, "Stepname"=w2234, "Pass/Fail"=w2232, "Actual"=w2219, "Result"=w2222) -> (w2239:T2)
              }
              frame "Byte" {
                n718 = Match Pattern(string=w2245, regular expression="_SW_") -> (offset past match=w2243:i32)  [unwired: 1 in, 3 out]
                n719 = case shown="0, Default" w2243 {
                  tunnel: w2252 -> [w2265 w2300]
                  tunnel: w2251 -> [w2270 w2299]
                  tunnel: [w2269 w2298] -> w2250
                  tunnel: [w2264 w2297] -> w2249
                  tunnel: w2248 -> [_ w2296]
                  tunnel: w2247 -> [w2267 w2294]
                  tunnel: w2245 -> [w2266 w2293]
                  tunnel: w2246 -> [_ w2284]
                  tunnel: w2242 -> [w2258 _]
                  frame 0, Default {
                    w2268 = "" ("LSL")
                    n720 = Equal?(x=w2258, y=1) -> (x = y?=w2262:bool)
                    n721 = Select(t=cluster{"Top":i16, "Left":i16} {"Top"=404, "Left"=150} ("Position"), s=w2262, f=cluster{"Top":i16, "Left":i16} {"Top"=404, "Left"=1300} ("Position")) -> (s? t:f=w2259:cluster{"Top":i16, "Left":i16})
                    n722 = To Variant(anything=w2258) -> (Variant=w2257:variant)
                    n723 = Build Array(w2257) -> (w2256:variant[])
                    n724 = call "Dynamic_Switch_EOL.vi"("error in (no error)"=w2265, "Value"=w2256, "Position"=w2259) -> ("error out"=w2264:errorcluster, "Pass/Fail"=w2254:string)  [unwired: 7 in]
                    n725 = Equal?(x=w2254, y="Pass") -> (x = y?=w2253:bool)
                    n726 = Bundle By Name(cluster=w2270, "LSL"=w2268, "USL"=w2268, "UNIT"=w2268, "Expected_Value"=w2268, "Scriptname"=w2267, "Stepname"=w2266, "Pass/Fail"=w2254, "Actual"=w2254, "Result"=w2253) -> (w2269:T2)
                  }
                  frame -1 {
                    w2271 = "" ("LSL")
                    w2276 = 0 ("index")
                    n727 = Unflatten From String(type=T19 {"Database"="", "Signal"="", "BYTES"=[], "ReadPayload"=[], "String_Data"="", "ReadValue"=0.0, "CANID"=0, "SERVICE ID"=0, "SUB-SERVICE ID"=0, "DELAY "=FALSE, "Delay time(ms)"=0.0} ("CAN_Read"), binary string=w2296, error in (no error)=w2300) -> (value=w2295:T19, error out=w2297:errorcluster)  [unwired: 2 in, 1 out]
                    n728 = Unbundle By Name(w2295) -> ("BYTES"=w2286:u32[], "ReadPayload"=w2280:u8[], "ReadValue"=w2275:dbl)
                    n729 = Index Array(array=w2286, index=w2276) -> (element=w2285:u32)
                    n730 = Index Array(array=w2280, index=w2276) -> (element=w2277:u8)
                    n731 = Index Array(array=w2284, index=w2285) -> (element=w2283:u8)
                    n732 = To Unsigned Byte Integer(number=w2283) -> (unsigned 8bit integer=w2282:u8)
                    n733 = To Long Integer(number=w2277) -> (32bit integer=w2279:i32)
                    n734 = Number To Boolean Array(number=w2282) -> (Boolean array=w2281:bool[])
                    n735 = Index Array(array=w2281, index=w2279) -> (element=w2278:bool)
                    n736 = To Word Integer(number=w2275) -> (16bit integer=w2274:i16)
                    n737 = Boolean To (0,1)(Boolean=w2278) -> (0, 1=w2273:i16)
                    n738 = Equal?(x=w2273, y=w2274) -> (x = y?=w2272:bool)
                    n739 = Select(t="Pass", s=w2272, f="Fail") -> (s? t:f=w2291:string)
                    n740 = Number To Decimal String(number=w2273) -> (decimal integer string=w2289:string)  [unwired: 1 in]
                    n741 = Bundle By Name(cluster=w2299, "LSL"=w2271, "USL"=w2271, "UNIT"=w2271, "Expected_Value"="1", "Scriptname"=w2294, "Stepname"=w2293, "Pass/Fail"=w2291, "Actual"=w2289, "Result"=w2278) -> (w2298:T2)
                  }
                }
              }
            }
          }
          frame "Camera" {
            w2305 = ""
            n742 = Bundle By Name(cluster=w2304, "UNIT"=w2305, "USL"=w2305, "LSL"=w2305, "Pass/Fail"=w2305, "Actual"=w2305, "Scriptname"=w2302, "Stepname"=w2301) -> (w2303:T2)
          }
          frame "READ_DATA" {
            (unwired) T12 0 items=["SET_VOLTAGE", "SET_CURRENT", "OUTPUT VOLTAGE", "OUTPUT CURRENT", "RESISTANCE", "OUTPUT POWER", "CAMERA", "SSL_Check"] ("PARAMETER")
            n743 = Unflatten From String(type=T10 {"EQUIPMENT"=0, "PARAMETER"=0, "LSL"=0.0, "USL"=0.0, "RESULT"="", "UNIT"="", "Delay"=FALSE, "Delay time"=0.0} ("READ_DATA"), binary string=w2314, error in (no error)=w2318) -> (value=w2316:T10, error out=w2317:errorcluster)  [unwired: 2 in, 1 out]
            n744 = Unbundle By Name(w2316) -> ("USL"=w2321:dbl, "EQUIPMENT"=w2326:T11, "LSL"=w2319:dbl, "RESULT"=w2320:string, "UNIT"=w2313:string, "PARAMETER"=w2311:T12)
            n745 = case shown="3" w2326 {
              tunnel: w2317 -> [w2346 w2373]
              tunnel: [w2345 w2372] -> w2327
              tunnel: w2325 -> [w2353 w2377]
              tunnel: [w2352 w2376] -> w2324
              tunnel: w2314 -> [_ _]
              tunnel: w2323 -> [w2351 w2375]
              tunnel: w2322 -> [w2350 w2374]
              tunnel: w2321 -> [w2332 _]
              tunnel: w2320 -> [_ _]
              tunnel: w2319 -> [w2334 _]
              tunnel: w2315 -> [w2344 w2371]
              tunnel: w2313 -> [w2338 _]
              tunnel: w2311 -> [_ w2367]
              tunnel: w2310 -> [_ w2366]
              tunnel: w2309 -> [_ w2365]
              tunnel: w2308 -> [_ w2364]
              tunnel: w2307 -> [_ w2363]
              frame 0..2, Default {
                # "PS, DMM, DAQ Read data"
                n746 = Variant To Data(error in=w2346, type="", Variant=w2344) -> (data=w2339:string, error out=w2345:errorcluster)
                n747 = Not Equal To 0?(x=w2332) -> (x != 0?=w2331:bool)
                n748 = call "Unit_value_maps.vi"("UNIT"=w2338, "Actual String"=w2339) -> ("Actual value"=w2335:dbl)  [unwired: 9 in]
                n749 = case shown="False" w2331 {
                  tunnel: w2335 -> [w2356 w2360]
                  tunnel: w2332 -> [_ w2359]
                  tunnel: w2334 -> [w2355 w2358]
                  tunnel: [w2354 w2357] -> w2333
                  frame False {
                    n750 = Greater Or Equal?(x=w2356, y=w2355) -> (x >= y?=w2354:bool)
                  }
                  frame True {
                    n751 = Greater Or Equal?(x=w2360, y=w2358) -> (x >= y?=w2362:bool)
                    n752 = Less Or Equal?(x=w2360, y=w2359) -> (x <= y?=w2361:bool)
                    n753 = And(x=w2362, y=w2361) -> (x .and. y?=w2357:bool)
                  }
                }
                n754 = Number To Fractional String(number=w2335, precision (6)=i16 2) -> (F-format string=w2336:string)  [unwired: 2 in]
                n755 = Number To Fractional String(number=w2332, precision (6)=i16 2) -> (F-format string=w2330:string)  [unwired: 2 in]
                n756 = Number To Fractional String(number=w2334, precision (6)=i16 2) -> (F-format string=w2340:string)  [unwired: 2 in]
                n757 = Select(t=w2330, s=w2331, f="Inf") -> (s? t:f=w2328:string)
                n758 = Select(t="Pass", s=w2333, f="Fail") -> (s? t:f=w2348:string)
                n759 = Bundle By Name(cluster=w2353, "USL"=w2328, "LSL"=w2340, "Scriptname"=w2351, "Stepname"=w2350, "Pass/Fail"=w2348, "Actual"=w2336, "Result"=w2333, "UNIT"=w2338) -> (w2352:T2)
              }
              frame 3 {
                # "Camera"
                n760 = case shown="7, Default" w2367 {
                  tunnel: w2373 -> [w2393 w2426]
                  tunnel: [w2389 w2412] -> w2372
                  tunnel: w2371 -> [w2392 w2424]
                  tunnel: [w2384 w2419] -> w2370
                  tunnel: [w2385 w2402] -> w2369
                  tunnel: [w2381 w2403] -> w2368
                  tunnel: w2366 -> [_ w2410]
                  tunnel: w2365 -> [w2391 _]
                  tunnel: w2364 -> [_ w2411]
                  tunnel: w2363 -> [_ w2409]
                  frame 7, Default {
                    n761 = Variant To Data(error in=w2393, type="", Variant=w2392) -> (data=w2380:string, error out=w2390:errorcluster)
                    n762 = call <vilib>:"Clear Errors.vi"("error in (no error)"=w2390) -> ("error out"=w2382:errorcluster)  [unwired: 5 in, 1 out]
                    n763 = Unbundle By Name(w2391) -> ("RX/RY"=w2379:string)
                    n764 = Not Equal?(x=w2379, y=w2380) -> (x != y?=w2378:bool)
                    n765 = Select(t=w2379, s=w2378, f=w2380) -> (s? t:f=w2381:string)
                    n766 = disable-structure shown="Enabled" {
                      disable-tunnel: w2379 -> [w2399 w2400]
                      disable-tunnel: _ -> [w2398 _]
                      disable-tunnel: [w2397 w2401] -> w2389
                      disable-tunnel: [w2396 w2400] -> w2388
                      disable-tunnel: w2382 -> [w2394 w2401]
                      frame Disabled {
                        n767 = call "SSL_Check.vi"("error in (no error)"=w2394, "Barcode_Can_Read"=w2399, "Section"="ssl_csv", "instrument file path"=w2398) -> ("error out"=w2397:errorcluster, "RX/RY"=w2396:string)  [unwired: 6 in]
                      }
                      frame Enabled {
                      }
                    }
                    n768 = Equal?(x=w2381, y=w2388) -> (x = y?=w2385:bool)
                    n769 = Select(t="Pass", s=w2385, f="Fail") -> (s? t:f=w2384:string)
                  }
                  frame 6 {
                    n770 = Variant To Data(error in=w2426, type=T38 {"Result"=TRUE, "DTU_Inspection_Data"=""}, Variant=w2424) -> (data=w2422:T38, error out=w2425:errorcluster)
                    n771 = call <vilib>:"Clear Errors.vi"("error in (no error)"=w2425) -> ("error out"=w2413:errorcluster)  [unwired: 5 in, 1 out]
                    n772 = disable-structure shown="Enabled" {
                      disable-tunnel: w2422 -> [w2429 _]
                      disable-tunnel: [w2428 TRUE] -> w2418
                      disable-tunnel: [w2427 "" ("Inspection Failed Segments")] -> w2414
                      frame Enabled {
                        n773 = Unbundle By Name(w2429) -> ("Result"=w2428:bool, "DTU_Inspection_Data"=w2427:string)
                      }
                      frame Disabled {
                      }
                    }
                    n774 = call "CAM_file_swap.vi"("error in"=w2413, "DUT"=w2411, "Barcode"=w2410) -> ("error out"=w2412:errorcluster, "Ref_img_path"=w2406:path, "DTU_Conf"=w2407:string, "image path"=w2408:path)  [unwired: 5 in]
                    n775 = call "Image_processor.vi"("DUT"=w2409, "Ref Folder"=w2406, "DUT_Conf"=w2407, "Image Path"=w2408) -> ("Fail_Strings"=w2404:string, "PASS/FAIL"=w2402:bool)  [unwired: 6 in]
                    n776 = Or(x=w2418, y=w2402) -> ()  [unwired: 1 out]
                    n777 = Select(t=T31."Disabled and Grayed Out" ("Disabled"), s=w2402, f=T31."Enabled" ("Disabled")) -> (s? t:f=w2416:T31)
                    n778 = property on="DTU Inspection Data" class="Str"("DisabledEnum"=w2416) -> ()  [unwired: 2 in, 2 out]
                    n779 = Select(t="Pass", s=w2402, f="Fail") -> (s? t:f=w2419:string)
                    n780 = Concatenate Strings(w2414, "_" ("string"), w2404) -> (w2403:string)
                    "DTU Inspection Data" <- w2403
                  }
                }
                n781 = Bundle By Name(cluster=w2377, "Scriptname"=w2375, "Stepname"=w2374, "Pass/Fail"=w2370, "Actual"=w2368, "Result"=w2369) -> (w2376:T2)
              }
            }
          }
        }
        n782 = Flush Queue(queue=w1630, error in (no error)=w1637) -> (queue out=w1629:refnum<queue>, error out=w1631:errorcluster)  [unwired: 1 out]
        n783 = call "Test_Enque_Message_FGV.vi"("Priority"=TRUE, "error in (no error)"=w1631, "Message"="BuildTable", "queue in"=w1629) -> ("error out"=w1636:errorcluster)  [unwired: 7 in]
      }
      frame "StepFeedback" {
        (unwired) string[] ["MCU_Flashing", "Noeway_Flashing"]
        (unwired) T11 0 items=["POWER SUPPLY", "DMM", "DAQ", "CAMERA"] ("EQUIPMENT")
        (unwired) string[] ["<Select>", "MP711134-14V", "MP711134-12V", "Keysight34461a", "DMM6500", "PCAN", "Relay_Module", "GNSS", "Bluetooth", "Noeway_Flashing", "MCU_Flashing"] ("Strings []")
        (unwired) StepType."RELAY_CHANNEL_WRITE" ("Type")
        # "Feedback from the step"
        n784 = Unbundle By Name(w2437) -> ("EQUP LIST"=w2432:string[], "Array_N"=w2439:refnum<notifier>[], "UI Data.ScriptDetails.Steps"=w2442:T5[], "Stepno."=w2441:u64)
        n785 = Index Array(array=w2442, index=w2441) -> (element=w2434:T5)
        n786 = Unbundle By Name(w2434) -> ("Type"=w2438:T6)
        n787 = Unbundle By Name(w2434) -> ("StepDetails"=w2433:string)
        n788 = case shown="\"Camera\"" w2438 {
          tunnel: w2443 -> [w2449 w2500 w2542 w2584 w2626 w2668 w2709 w2750 w2787 w2797 w2838]
          tunnel: [w2459 w2497 w2539 w2581 w2623 w2665 w2706 w2747 w2786 w2794 w2847] -> w2440
          tunnel: w2439 -> [w2466 w2501 w2543 w2585 w2621 w2663 w2704 w2751 _ w2798 w2851]
          tunnel: w2437 -> [w2457 w2499 w2541 w2583 w2625 w2667 w2708 w2749 w2789 w2796 w2846]
          tunnel: [w2456 w2498 w2540 w2582 w2624 w2666 w2707 w2748 w2789 w2795 w2845] -> w2436
          tunnel: w2435 -> [w2455 w2496 w2538 w2580 w2622 w2664 w2705 w2746 w2785 w2793 w2840]
          tunnel: w2433 -> [w2447 _ _ _ _ _ _ _ _ _ w2837]
          tunnel: w2432 -> [w2451 w2495 w2536 w2578 _ _ _ w2744 _ w2792 w2833]
          frame "PS_WRITE", Default {
            n789 = Unflatten From String(type=T7 {"Set_parameter"=0, "VOLTAGE"="", "CURRENT"="", "OUTPUT"=FALSE, "Delay"=FALSE, "Delay time"=0.0} ("PS_Write"), binary string=w2447, error in (no error)=w2449) -> (value=w2446:T7, error out=w2448:errorcluster)  [unwired: 2 in, 1 out]
            n790 = Unbundle By Name(w2446) -> ("VOLTAGE"=w2445:string)
            n791 = Concatenate Strings("MP711134-", w2445, "V") -> (w2452:string)
            n792 = Search 1D Array(1D array=w2451, element=w2452) -> (index of element=w2444:i32)  [unwired: 1 in]
            n793 = Index Array(array=w2466, index=w2444) -> (element=w2465:refnum<notifier>)
            n794 = Wait on Notification(notifier=w2465, timeout in ms (-1)=500, error in (no error)=w2448) -> (notifier out=w2461:refnum<notifier>, notification=w2463:T25, error out=w2460:errorcluster)  [unwired: 1 in, 1 out]
            n795 = Unbundle By Name(w2463) -> ("Message"=w2462:string, "Message Data"=w2458:variant)
            n796 = case shown="\"Read\", Default" w2462 {
              tunnel: w2461 -> [w2472 _ _ w2491]
              tunnel: w2460 -> [w2473 w2477 w2482 w2492]
              tunnel: [w2469 w2476 w2481 w2485] -> w2459
              tunnel: w2458 -> [_ _ _ w2489]
              tunnel: w2457 -> [w2468 w2475 w2480 w2490]
              tunnel: [w2468 w2475 w2480 w2488] -> w2456
              tunnel: w2455 -> [w2467 w2474 w2479 w2484]
              frame "Step_Done" {
                n797 = Cancel Notification(0:w2472, 3:w2473) -> (11:w2470:errorcluster)  [unwired: 2 out]
                n798 = call "Test_Enque_Message_FGV.vi"("error in (no error)"=w2470, "Message"="GetData", "queue in"=w2467) -> ("error out"=w2469:errorcluster)  [unwired: 8 in]
              }
              frame "Error" {
                n799 = call "Test_Enque_Message_FGV.vi"("error in (no error)"=w2477, "Message"="Error", "queue in"=w2474) -> ("error out"=w2476:errorcluster)  [unwired: 8 in]
              }
              frame "" {
                n800 = call "Test_Enque_Message_FGV.vi"("error in (no error)"=w2482, "Message"="StepFeedback", "queue in"=w2479) -> ("error out"=w2481:errorcluster)  [unwired: 8 in]
              }
              frame "Read", Default {
                n801 = Cancel Notification(0:w2491, 3:w2492) -> (11:w2486:errorcluster)  [unwired: 2 out]
                n802 = Bundle By Name(cluster=w2490, "Message Data"=w2489) -> (w2488:T2)
                n803 = call "Test_Enque_Message_FGV.vi"("error in (no error)"=w2486, "Message"="GetData", "queue in"=w2484) -> ("error out"=w2485:errorcluster)  [unwired: 8 in]
              }
            }
          }
          frame "DMM_CONFIG" {
            n804 = Search 1D Array(1D array=w2495, element="Keysight34461a") -> (index of element=w2493:i32)  [unwired: 1 in]
            n805 = Index Array(array=w2501, index=w2493) -> (element=w2508:refnum<notifier>)
            n806 = Wait on Notification(notifier=w2508, timeout in ms (-1)=500, error in (no error)=w2500) -> (notifier out=w2504:refnum<notifier>, notification=w2506:T25, error out=w2503:errorcluster)  [unwired: 1 in, 1 out]
            n807 = Unbundle By Name(w2506) -> ("Message"=w2505:string, "Message Data"=w2502:variant)
            n808 = case shown="\"Step_Done\"" w2505 {
              tunnel: w2504 -> [w2514 _ _ w2533]
              tunnel: w2503 -> [w2515 w2519 w2524 w2534]
              tunnel: [w2511 w2518 w2523 w2527] -> w2497
              tunnel: w2502 -> [_ _ _ w2531]
              tunnel: w2499 -> [w2510 w2517 w2522 w2532]
              tunnel: [w2510 w2517 w2522 w2530] -> w2498
              tunnel: w2496 -> [w2509 w2516 w2521 w2526]
              frame "Step_Done" {
                n809 = Cancel Notification(0:w2514, 3:w2515) -> (11:w2512:errorcluster)  [unwired: 2 out]
                n810 = call "Test_Enque_Message_FGV.vi"("error in (no error)"=w2512, "Message"="GetData", "queue in"=w2509) -> ("error out"=w2511:errorcluster)  [unwired: 8 in]
              }
              frame "Error" {
                n811 = call "Test_Enque_Message_FGV.vi"("error in (no error)"=w2519, "Message"="Error", "queue in"=w2516) -> ("error out"=w2518:errorcluster)  [unwired: 8 in]
              }
              frame "" {
                n812 = call "Test_Enque_Message_FGV.vi"("error in (no error)"=w2524, "Message"="StepFeedback", "queue in"=w2521) -> ("error out"=w2523:errorcluster)  [unwired: 8 in]
              }
              frame "Read", Default {
                n813 = Cancel Notification(0:w2533, 3:w2534) -> (11:w2528:errorcluster)  [unwired: 2 out]
                n814 = Bundle By Name(cluster=w2532, "Message Data"=w2531) -> (w2530:T2)
                n815 = call "Test_Enque_Message_FGV.vi"("error in (no error)"=w2528, "Message"="GetData", "queue in"=w2526) -> ("error out"=w2527:errorcluster)  [unwired: 8 in]
              }
            }
          }
          frame "PCAN_Read" {
            n816 = Search 1D Array(1D array=w2536, element="PCAN") -> (index of element=w2535:i32)  [unwired: 1 in]
            n817 = Index Array(array=w2543, index=w2535) -> (element=w2550:refnum<notifier>)
            n818 = Wait on Notification(notifier=w2550, timeout in ms (-1)=500, error in (no error)=w2542) -> (notifier out=w2546:refnum<notifier>, notification=w2548:T25, error out=w2545:errorcluster)  [unwired: 1 in, 1 out]
            n819 = Unbundle By Name(w2548) -> ("Message"=w2547:string, "Message Data"=w2544:variant)
            n820 = case shown="\"Read\", Default" w2547 {
              tunnel: w2546 -> [w2556 _ _ w2575]
              tunnel: w2545 -> [w2557 w2561 w2566 w2576]
              tunnel: [w2553 w2560 w2565 w2569] -> w2539
              tunnel: w2544 -> [_ _ _ w2573]
              tunnel: w2541 -> [w2552 w2559 w2564 w2574]
              tunnel: [w2552 w2559 w2564 w2572] -> w2540
              tunnel: w2538 -> [w2551 w2558 w2563 w2568]
              frame "Step_Done" {
                n821 = Cancel Notification(0:w2556, 3:w2557) -> (11:w2554:errorcluster)  [unwired: 2 out]
                n822 = call "Test_Enque_Message_FGV.vi"("error in (no error)"=w2554, "Message"="GetData", "queue in"=w2551) -> ("error out"=w2553:errorcluster)  [unwired: 8 in]
              }
              frame "Error" {
                n823 = call "Test_Enque_Message_FGV.vi"("error in (no error)"=w2561, "Message"="Error", "queue in"=w2558) -> ("error out"=w2560:errorcluster)  [unwired: 8 in]
              }
              frame "" {
                n824 = call "Test_Enque_Message_FGV.vi"("error in (no error)"=w2566, "Message"="StepFeedback", "queue in"=w2563) -> ("error out"=w2565:errorcluster)  [unwired: 8 in]
              }
              frame "Read", Default {
                n825 = Cancel Notification(0:w2575, 3:w2576) -> (11:w2570:errorcluster)  [unwired: 2 out]
                n826 = Bundle By Name(cluster=w2574, "Message Data"=w2573) -> (w2572:T2)
                n827 = call "Test_Enque_Message_FGV.vi"("error in (no error)"=w2570, "Message"="GetData", "queue in"=w2568) -> ("error out"=w2569:errorcluster)  [unwired: 8 in]
              }
            }
          }
          frame "PCAN_Write" {
            n828 = Search 1D Array(1D array=w2578, element="PCAN") -> (index of element=w2577:i32)  [unwired: 1 in]
            n829 = Index Array(array=w2585, index=w2577) -> (element=w2592:refnum<notifier>)
            n830 = Wait on Notification(notifier=w2592, timeout in ms (-1)=500, error in (no error)=w2584) -> (notifier out=w2588:refnum<notifier>, notification=w2590:T25, error out=w2587:errorcluster)  [unwired: 1 in, 1 out]
            n831 = Unbundle By Name(w2590) -> ("Message"=w2589:string, "Message Data"=w2586:variant)
            n832 = case shown="\"Read\", Default" w2589 {
              tunnel: w2588 -> [w2598 _ _ w2617]
              tunnel: w2587 -> [w2599 w2603 w2608 w2618]
              tunnel: [w2595 w2602 w2607 w2611] -> w2581
              tunnel: w2586 -> [_ _ _ w2615]
              tunnel: w2583 -> [w2594 w2601 w2606 w2616]
              tunnel: [w2594 w2601 w2606 w2614] -> w2582
              tunnel: w2580 -> [w2593 w2600 w2605 w2610]
              frame "Step_Done" {
                n833 = Cancel Notification(0:w2598, 3:w2599) -> (11:w2596:errorcluster)  [unwired: 2 out]
                n834 = call "Test_Enque_Message_FGV.vi"("error in (no error)"=w2596, "Message"="GetData", "queue in"=w2593) -> ("error out"=w2595:errorcluster)  [unwired: 8 in]
              }
              frame "Error" {
                n835 = call "Test_Enque_Message_FGV.vi"("error in (no error)"=w2603, "Message"="Error", "queue in"=w2600) -> ("error out"=w2602:errorcluster)  [unwired: 8 in]
              }
              frame "" {
                n836 = call "Test_Enque_Message_FGV.vi"("error in (no error)"=w2608, "Message"="StepFeedback", "queue in"=w2605) -> ("error out"=w2607:errorcluster)  [unwired: 8 in]
              }
              frame "Read", Default {
                n837 = Cancel Notification(0:w2617, 3:w2618) -> (11:w2612:errorcluster)  [unwired: 2 out]
                n838 = Bundle By Name(cluster=w2616, "Message Data"=w2615) -> (w2614:T2)
                n839 = call "Test_Enque_Message_FGV.vi"("error in (no error)"=w2612, "Message"="GetData", "queue in"=w2610) -> ("error out"=w2611:errorcluster)  [unwired: 8 in]
              }
            }
          }
          frame "Camera" {
            (unwired) "Keyence_VS150"
            n840 = Array Size(array=w2621) -> (size(s)=w2620:i32)
            n841 = Decrement(x=w2620) -> (x-1=w2619:i32)
            n842 = Index Array(array=w2621, index=w2619) -> (element=w2633:refnum<notifier>)
            n843 = Wait on Notification(notifier=w2633, timeout in ms (-1)=500, error in (no error)=w2626) -> (notifier out=w2629:refnum<notifier>, notification=w2631:T25, error out=w2628:errorcluster)  [unwired: 1 in, 1 out]
            n844 = Unbundle By Name(w2631) -> ("Message"=w2630:string, "Message Data"=w2627:variant)
            n845 = case shown="\"Step_Done\"" w2630 {
              tunnel: w2629 -> [w2639 _ _ w2658]
              tunnel: w2628 -> [w2640 w2644 w2649 w2659]
              tunnel: [w2636 w2643 w2648 w2652] -> w2623
              tunnel: w2627 -> [_ _ _ w2656]
              tunnel: w2625 -> [w2635 w2642 w2647 w2657]
              tunnel: [w2635 w2642 w2647 w2655] -> w2624
              tunnel: w2622 -> [w2634 w2641 w2646 w2651]
              frame "Step_Done" {
                n846 = Cancel Notification(0:w2639, 3:w2640) -> (11:w2637:errorcluster)  [unwired: 2 out]
                n847 = call "Test_Enque_Message_FGV.vi"("error in (no error)"=w2637, "Message"="GetData", "queue in"=w2634) -> ("error out"=w2636:errorcluster)  [unwired: 8 in]
              }
              frame "Error" {
                n848 = call "Test_Enque_Message_FGV.vi"("error in (no error)"=w2644, "Message"="Error", "queue in"=w2641) -> ("error out"=w2643:errorcluster)  [unwired: 8 in]
              }
              frame "" {
                n849 = call "Test_Enque_Message_FGV.vi"("error in (no error)"=w2649, "Message"="StepFeedback", "queue in"=w2646) -> ("error out"=w2648:errorcluster)  [unwired: 8 in]
              }
              frame "Read", Default {
                n850 = Cancel Notification(0:w2658, 3:w2659) -> (11:w2653:errorcluster)  [unwired: 2 out]
                n851 = Bundle By Name(cluster=w2657, "Message Data"=w2656) -> (w2655:T2)
                n852 = call "Test_Enque_Message_FGV.vi"("error in (no error)"=w2653, "Message"="GetData", "queue in"=w2651) -> ("error out"=w2652:errorcluster)  [unwired: 8 in]
              }
            }
          }
          frame "MCU_Flashing" {
            n853 = Array Size(array=w2663) -> (size(s)=w2661:i32)
            n854 = Subtract(x=w2661, y=2) -> (x-y=w2662:i32)
            n855 = Index Array(array=w2663, index=w2662) -> (element=w2675:refnum<notifier>)
            n856 = Wait on Notification(notifier=w2675, timeout in ms (-1)=500, error in (no error)=w2668) -> (notifier out=w2671:refnum<notifier>, notification=w2673:T25, error out=w2670:errorcluster)  [unwired: 1 in, 1 out]
            n857 = Unbundle By Name(w2673) -> ("Message"=w2672:string, "Message Data"=w2669:variant)
            n858 = case shown="\"Read\", Default" w2672 {
              tunnel: w2671 -> [w2681 _ _ w2700]
              tunnel: w2670 -> [w2682 w2686 w2691 w2701]
              tunnel: [w2678 w2685 w2690 w2694] -> w2665
              tunnel: w2669 -> [_ _ _ w2698]
              tunnel: w2667 -> [w2677 w2684 w2689 w2699]
              tunnel: [w2677 w2684 w2689 w2697] -> w2666
              tunnel: w2664 -> [w2676 w2683 w2688 w2693]
              frame "Step_Done" {
                n859 = Cancel Notification(0:w2681, 3:w2682) -> (11:w2679:errorcluster)  [unwired: 2 out]
                n860 = call "Test_Enque_Message_FGV.vi"("error in (no error)"=w2679, "Message"="GetData", "queue in"=w2676) -> ("error out"=w2678:errorcluster)  [unwired: 8 in]
              }
              frame "Error" {
                n861 = call "Test_Enque_Message_FGV.vi"("error in (no error)"=w2686, "Message"="Error", "queue in"=w2683) -> ("error out"=w2685:errorcluster)  [unwired: 8 in]
              }
              frame "" {
                n862 = call "Test_Enque_Message_FGV.vi"("error in (no error)"=w2691, "Message"="StepFeedback", "queue in"=w2688) -> ("error out"=w2690:errorcluster)  [unwired: 8 in]
              }
              frame "Read", Default {
                n863 = Cancel Notification(0:w2700, 3:w2701) -> (11:w2695:errorcluster)  [unwired: 2 out]
                n864 = Bundle By Name(cluster=w2699, "Message Data"=w2698) -> (w2697:T2)
                n865 = call "Test_Enque_Message_FGV.vi"("error in (no error)"=w2695, "Message"="GetData", "queue in"=w2693) -> ("error out"=w2694:errorcluster)  [unwired: 8 in]
              }
            }
          }
          frame "Noeway_Flashing" {
            n866 = Array Size(array=w2704) -> (size(s)=w2703:i32)
            n867 = Decrement(x=w2703) -> (x-1=w2702:i32)
            n868 = Index Array(array=w2704, index=w2702) -> (element=w2716:refnum<notifier>)
            n869 = Wait on Notification(notifier=w2716, timeout in ms (-1)=500, error in (no error)=w2709) -> (notifier out=w2712:refnum<notifier>, notification=w2714:T25, error out=w2711:errorcluster)  [unwired: 1 in, 1 out]
            n870 = Unbundle By Name(w2714) -> ("Message"=w2713:string, "Message Data"=w2710:variant)
            n871 = case shown="\"Read\", Default" w2713 {
              tunnel: w2712 -> [w2722 _ _ w2741]
              tunnel: w2711 -> [w2723 w2727 w2732 w2742]
              tunnel: [w2719 w2726 w2731 w2735] -> w2706
              tunnel: w2710 -> [_ _ _ w2739]
              tunnel: w2708 -> [w2718 w2725 w2730 w2740]
              tunnel: [w2718 w2725 w2730 w2738] -> w2707
              tunnel: w2705 -> [w2717 w2724 w2729 w2734]
              frame "Step_Done" {
                n872 = Cancel Notification(0:w2722, 3:w2723) -> (11:w2720:errorcluster)  [unwired: 2 out]
                n873 = call "Test_Enque_Message_FGV.vi"("error in (no error)"=w2720, "Message"="GetData", "queue in"=w2717) -> ("error out"=w2719:errorcluster)  [unwired: 8 in]
              }
              frame "Error" {
                n874 = call "Test_Enque_Message_FGV.vi"("error in (no error)"=w2727, "Message"="Error", "queue in"=w2724) -> ("error out"=w2726:errorcluster)  [unwired: 8 in]
              }
              frame "" {
                n875 = call "Test_Enque_Message_FGV.vi"("error in (no error)"=w2732, "Message"="StepFeedback", "queue in"=w2729) -> ("error out"=w2731:errorcluster)  [unwired: 8 in]
              }
              frame "Read", Default {
                n876 = Cancel Notification(0:w2741, 3:w2742) -> (11:w2736:errorcluster)  [unwired: 2 out]
                n877 = Bundle By Name(cluster=w2740, "Message Data"=w2739) -> (w2738:T2)
                n878 = call "Test_Enque_Message_FGV.vi"("error in (no error)"=w2736, "Message"="GetData", "queue in"=w2734) -> ("error out"=w2735:errorcluster)  [unwired: 8 in]
              }
            }
          }
          frame "DAQ_CONFIG" {
            n879 = Search 1D Array(1D array=w2744, element="DMM6500") -> (index of element=w2743:i32)  [unwired: 1 in]
            n880 = Index Array(array=w2751, index=w2743) -> (element=w2758:refnum<notifier>)
            n881 = Wait on Notification(notifier=w2758, timeout in ms (-1)=500, error in (no error)=w2750) -> (notifier out=w2754:refnum<notifier>, notification=w2756:T25, error out=w2753:errorcluster)  [unwired: 1 in, 1 out]
            n882 = Unbundle By Name(w2756) -> ("Message"=w2755:string, "Message Data"=w2752:variant)
            n883 = case shown="\"Read\", Default" w2755 {
              tunnel: w2754 -> [w2764 _ _ w2783]
              tunnel: w2753 -> [w2765 w2769 w2774 w2784]
              tunnel: [w2761 w2768 w2773 w2777] -> w2747
              tunnel: w2752 -> [_ _ _ w2781]
              tunnel: w2749 -> [w2760 w2767 w2772 w2782]
              tunnel: [w2760 w2767 w2772 w2780] -> w2748
              tunnel: w2746 -> [w2759 w2766 w2771 w2776]
              frame "Step_Done" {
                n884 = Cancel Notification(0:w2764, 3:w2765) -> (11:w2762:errorcluster)  [unwired: 2 out]
                n885 = call "Test_Enque_Message_FGV.vi"("error in (no error)"=w2762, "Message"="GetData", "queue in"=w2759) -> ("error out"=w2761:errorcluster)  [unwired: 8 in]
              }
              frame "Error" {
                n886 = call "Test_Enque_Message_FGV.vi"("error in (no error)"=w2769, "Message"="Error", "queue in"=w2766) -> ("error out"=w2768:errorcluster)  [unwired: 8 in]
              }
              frame "" {
                n887 = call "Test_Enque_Message_FGV.vi"("error in (no error)"=w2774, "Message"="StepFeedback", "queue in"=w2771) -> ("error out"=w2773:errorcluster)  [unwired: 8 in]
              }
              frame "Read", Default {
                n888 = Cancel Notification(0:w2783, 3:w2784) -> (11:w2778:errorcluster)  [unwired: 2 out]
                n889 = Bundle By Name(cluster=w2782, "Message Data"=w2781) -> (w2780:T2)
                n890 = call "Test_Enque_Message_FGV.vi"("error in (no error)"=w2778, "Message"="GetData", "queue in"=w2776) -> ("error out"=w2777:errorcluster)  [unwired: 8 in]
              }
            }
          }
          frame "SSL_Certification" {
            n891 = call "Test_Enque_Message_FGV.vi"("error in (no error)"=w2787, "Message"="GetData", "queue in"=w2785) -> ("error out"=w2786:errorcluster)  [unwired: 8 in]
          }
          frame "RELAY_CHANNEL_WRITE" {
            n892 = Search 1D Array(1D array=w2792, element="Relay_Module") -> (index of element=w2790:i32)  [unwired: 1 in]
            n893 = Index Array(array=w2798, index=w2790) -> (element=w2805:refnum<notifier>)
            n894 = Wait on Notification(notifier=w2805, timeout in ms (-1)=500, error in (no error)=w2797) -> (notifier out=w2801:refnum<notifier>, notification=w2803:T25, error out=w2800:errorcluster)  [unwired: 1 in, 1 out]
            n895 = Unbundle By Name(w2803) -> ("Message"=w2802:string, "Message Data"=w2799:variant)
            n896 = case shown="\"Read\", Default" w2802 {
              tunnel: w2801 -> [w2811 _ _ w2830]
              tunnel: w2800 -> [w2812 w2816 w2821 w2831]
              tunnel: [w2808 w2815 w2820 w2824] -> w2794
              tunnel: w2799 -> [_ _ _ w2828]
              tunnel: w2796 -> [w2807 w2814 w2819 w2829]
              tunnel: [w2807 w2814 w2819 w2827] -> w2795
              tunnel: w2793 -> [w2806 w2813 w2818 w2823]
              frame "Step_Done" {
                n897 = Cancel Notification(0:w2811, 3:w2812) -> (11:w2809:errorcluster)  [unwired: 2 out]
                n898 = call "Test_Enque_Message_FGV.vi"("error in (no error)"=w2809, "Message"="GetData", "queue in"=w2806) -> ("error out"=w2808:errorcluster)  [unwired: 8 in]
              }
              frame "Error" {
                n899 = call "Test_Enque_Message_FGV.vi"("error in (no error)"=w2816, "Message"="Error", "queue in"=w2813) -> ("error out"=w2815:errorcluster)  [unwired: 8 in]
              }
              frame "" {
                n900 = call "Test_Enque_Message_FGV.vi"("error in (no error)"=w2821, "Message"="StepFeedback", "queue in"=w2818) -> ("error out"=w2820:errorcluster)  [unwired: 8 in]
              }
              frame "Read", Default {
                n901 = Cancel Notification(0:w2830, 3:w2831) -> (11:w2825:errorcluster)  [unwired: 2 out]
                n902 = Bundle By Name(cluster=w2829, "Message Data"=w2828) -> (w2827:T2)
                n903 = call "Test_Enque_Message_FGV.vi"("error in (no error)"=w2825, "Message"="GetData", "queue in"=w2823) -> ("error out"=w2824:errorcluster)  [unwired: 8 in]
              }
            }
          }
          frame "READ_DATA" {
            n904 = Unflatten From String(type=T10 {"EQUIPMENT"=0, "PARAMETER"=0, "LSL"=0.0, "USL"=0.0, "RESULT"="", "UNIT"="", "Delay"=FALSE, "Delay time"=0.0} ("READ_DATAS"), binary string=w2837, error in (no error)=w2838) -> (value=w2836:T10, error out=w2834:errorcluster)  [unwired: 2 in, 1 out]
            n905 = Unbundle By Name(w2836) -> ("EQUIPMENT"=w2835:T11, "RESULT"=w2832:string)
            n906 = case shown="3" w2835 {
              tunnel: w2851 -> [w2859 w2864 w2869 w2872]
              tunnel: [w2858 w2863 w2868 w2873] -> w2850
              tunnel: w2833 -> [w2852 w2861 w2866 _]
              tunnel: w2832 -> [w2854 _ _ _]
              frame 0, Default {
                # "PS"
                n907 = Concatenate Strings("MP711134-", w2854, "V") -> (w2855:string)
                n908 = Search 1D Array(1D array=w2852, element=w2855) -> (index of element=w2853:i32)  [unwired: 1 in]
                n909 = Index Array(array=w2859, index=w2853) -> (element=w2858:refnum<notifier>)
              }
              frame 1 {
                # "DMM"
                n910 = Search 1D Array(1D array=w2861, element="Keysight34461a") -> (index of element=w2860:i32)  [unwired: 1 in]
                n911 = Index Array(array=w2864, index=w2860) -> (element=w2863:refnum<notifier>)
              }
              frame 2 {
                # "DAQ"
                n912 = Search 1D Array(1D array=w2866, element="DMM6500") -> (index of element=w2865:i32)  [unwired: 1 in]
                n913 = Index Array(array=w2869, index=w2865) -> (element=w2868:refnum<notifier>)
              }
              frame 3 {
                (unwired) "Keyence_VS150"
                # "CAMERA"
                n914 = Array Size(array=w2872) -> (size(s)=w2871:i32)
                n915 = Decrement(x=w2871) -> (x-1=w2870:i32)
                n916 = Index Array(array=w2872, index=w2870) -> (element=w2873:refnum<notifier>)
              }
            }
            n917 = Wait on Notification(notifier=w2850, timeout in ms (-1)=1000, error in (no error)=w2834) -> (notifier out=w2843:refnum<notifier>, notification=w2844:T25, error out=w2848:errorcluster)  [unwired: 1 in, 1 out]
            n918 = Unbundle(w2844) -> ("Message"=w2842:string, "Message Data"=w2841:variant)
            n919 = case shown="\"\"" w2842 {
              tunnel: w2843 -> [w2879 _ _ w2898]
              tunnel: w2848 -> [w2880 w2884 w2889 w2899]
              tunnel: [w2876 w2883 w2888 w2892] -> w2847
              tunnel: w2841 -> [_ _ _ w2896]
              tunnel: w2846 -> [w2875 w2882 w2887 w2897]
              tunnel: [w2875 w2882 w2887 w2895] -> w2845
              tunnel: w2840 -> [w2874 w2881 w2886 w2891]
              frame "Step_Done" {
                n920 = Cancel Notification(0:w2879, 3:w2880) -> (11:w2877:errorcluster)  [unwired: 2 out]
                n921 = call "Test_Enque_Message_FGV.vi"("error in (no error)"=w2877, "Message"="GetData", "queue in"=w2874) -> ("error out"=w2876:errorcluster)  [unwired: 8 in]
              }
              frame "Error" {
                n922 = call "Test_Enque_Message_FGV.vi"("error in (no error)"=w2884, "Message"="Error", "queue in"=w2881) -> ("error out"=w2883:errorcluster)  [unwired: 8 in]
              }
              frame "" {
                n923 = call "Test_Enque_Message_FGV.vi"("error in (no error)"=w2889, "Message"="StepFeedback", "queue in"=w2886) -> ("error out"=w2888:errorcluster)  [unwired: 8 in]
              }
              frame "Read", Default {
                n924 = Cancel Notification(0:w2898, 3:w2899) -> (11:w2893:errorcluster)  [unwired: 2 out]
                n925 = Bundle By Name(cluster=w2897, "Message Data"=w2896) -> (w2895:T2)
                n926 = call "Test_Enque_Message_FGV.vi"("error in (no error)"=w2893, "Message"="GetData", "queue in"=w2891) -> ("error out"=w2892:errorcluster)  [unwired: 8 in]
              }
            }
          }
        }
      }
      frame "BuildTable" {
        n927 = Unbundle By Name(w2931) -> ("Table"=w2930:string[][], "Scriptname"=w2929:string, "Stepname"=w2917:string, "LSL"=w2928:string, "Actual"=w2910:string, "USL"=w2909:string, "Pass/Fail"=w2908:string, "UNIT"=w2919:string, "Stepno."=w2920:u64)
        n928 = Match Pattern(string=w2917, regular expression="Read") -> (offset past match=w2915:i32)  [unwired: 1 in, 3 out]
        n929 = Build Array(w2929, w2917, w2928, w2910, w2909, w2908, w2919) -> (w2927:string[])
        n930 = case shown="0, Default" w2915 {
          tunnel: w2930 -> [w2955 w2958]
          tunnel: w2927 -> [w2954 w2957]
          tunnel: [w2953 w2956] -> w2918
          frame 0, Default {
            n931 = Build Array (concatenate)(w2955, w2954) -> (w2953:string[][])
          }
          frame -1 {
            n932 = Build Array (concatenate)(w2958, w2957) -> (w2956:string[][])
          }
        }
        n933 = Increment(x=w2920) -> (x+1=w2922:u64)
        n934 = Bundle By Name(cluster=w2931, "Table"=w2918, "Stepno."=w2922, "LaunchStep"=FALSE, "Delay"=FALSE) -> (w2926:T2)
        n935 = Equal?(x=w2908, y="Pass") -> (x = y?=w2913:bool)
        n936 = Not Equal?(x=w2908, y="Fail" ("f")) -> (x != y?=w2906:bool)
        n937 = Select(t=string[] ["Update Display", "Waittime", "IndexStep"] ("f"), s=w2906, f=string[] ["StopTest", "Update Display", "Pass/Fail", "Product_CNT", "Save", "Print"] ("Message Array")) -> (s? t:f=w2900:string[])
        n938 = case shown="0, Default" w2915 {
          tunnel: w2918 -> [w2951 _]
          tunnel: w2913 -> [w2944 _]
          frame 0, Default {
            n939 = Array Size(array=w2951) -> (size(s)=w2950:i32[])
            n940 = Index Array(array=w2950) -> (element=w2947:i32)  [unwired: 1 in]
            n941 = Decrement(x=w2947) -> (x-1=w2939:i32)
            n942 = Bundle By Name(cluster=T30 {"Row"=0, "Column"=0} ("Active Cell:Active Cell"), "Row"=w2939, "Column"=5) -> (w2948:T30)
            n943 = control-ref of="Table"() -> (w2952:refnum<vi>)
            n944 = property class="Tbl (strict)"(reference=w2952, "Active Cell"=w2948) -> (reference out=w2945:refnum<vi>)  [unwired: 1 in, 1 out]
            n945 = Select(t=u32 6618880 ("Active Cell:Cell Background Color"), s=w2944, f=u32 16748288 ("Active Cell:Cell Background Color")) -> (s? t:f=w2942:u32)
            n946 = property class="Tbl (strict)"(reference=w2945, "Cell BG Color"=w2942, "CellFontBold"=TRUE ("Active Cell:Cell Font:Bold")) -> ()  [unwired: 1 in, 2 out]
          }
          frame -1 {
          }
        }
        n947 = global read "Global 1.vi" "ENG_Mode"() -> (w2902:bool)
        n948 = disable-structure shown="Enabled" {
          disable-tunnel: w2932 -> [w2936 w2938]
          disable-tunnel: [w2935 w2938] -> w2925
          disable-tunnel: [w2933 w2937] -> w2923
          disable-tunnel: w2911 -> [_ w2937]
          frame Disabled {
            n949 = call "Test_Queue_Comm_FGV.vi"("error in (no error)"=w2936, "Enum"=Test_FGV_Queue_Control."Get") -> ("error Out"=w2935:errorcluster, "queue Out"=w2933:refnum<queue>)  [unwired: 8 in]
          }
          frame Enabled {
          }
        }
        n950 = Select(t=string[] ["Update Display", "Waittime", "IndexStep"] ("f"), s=w2902, f=w2900) -> (s? t:f=w2903:string[])
        n951 = call "Test_Enqueue Message (Array).vi"("error in (no error)"=w2925, "Message Array"=w2903, "Message Queue"=w2923) -> ("error out"=w2924:errorcluster)  [unwired: 7 in, 1 out]
      }
      frame "StopTest" {
        w2974 = FALSE ("Test Started?")
        n952 = flat-sequence {
          tunnel: w2977 -> [w2989]
          tunnel: [w2989] -> w2975
          tunnel: [w2988] -> _
          tunnel: [w2988] -> w2965
          frame #0 {
            n953 = global write "Global 1.vi" "Write_Exit 2"(TRUE ("Write_Exit")) -> ()
            n954 = local read "EOL/FCT"() -> (w2988:bool)
          }
        }
        n955 = Unbundle By Name(w2973) -> ("Seconds"=w2964:u32, "Table"=w2980:string[][], "EQUP LIST"=w2971:string[], "Array_Q"=w2969:refnum<queue>[])
        n956 = Tick Count (ms)() -> (millisecond timer value=w2963:u32)
        n957 = Subtract(x=w2963, y=w2964) -> (x-y=w2962:u32)
        n958 = property on="Start Button" class="Bool"(error in=w2975, "DisabledEnum"=T31."Enabled" ("Disabled")) -> (error out=w2967:errorcluster)  [unwired: 1 in, 1 out]
        n959 = Divide(x=w2962, y=u32 1000) -> (x/y=w2960:dbl)
        n960 = To Long Integer(number=w2960) -> (32bit integer=→"Total Time(s)":i32)
        n961 = Search 1D Array(1D array=w2971, element="PCAN") -> (index of element=w2970:i32)  [unwired: 1 in]
        n962 = Index Array(array=w2969, index=w2970) -> (element=w2968:refnum<queue>)
        n963 = case shown="True" w2965 {
          tunnel: w2968 -> [_ w2985]
          tunnel: w2967 -> [w2982 w2984]
          tunnel: [w2982 w2983] -> w2966
          frame False {
          }
          frame True {
            n964 = call "Enque_Message_FGV.vi"("Priority"=TRUE, "error in (no error)"=w2984, "Message"="Uninit_PCAN", "queue IN"=w2985) -> ("error out"=w2983:errorcluster)  [unwired: 7 in]
          }
        }
        n965 = local write "Test Started?"(w2974) -> ()
        n966 = Bundle By Name(cluster=w2973, "Test Started?"=w2974, "Table"=w2980) -> (w2981:T2)
        n967 = property on="Abort" class="Bool"(error in=w2966, "DisabledEnum"=T31."Disabled and Grayed Out" ("Disabled")) -> (error out=w2979:errorcluster)  [unwired: 1 in, 1 out]
      }
      frame "Pass/Fail" {
        # "Pass / Fail logic"
        n968 = Unbundle By Name(w3014) -> ("Part Count"=w3000:T1, "Table"=w3013:string[][], "DUT"=w2991:i32)
        n969 = Index Array(array=w3013, index (col)=5 ("disabled index (col)")) -> (element=w3011:string[])  [unwired: 1 in]
        n970 = Search 1D Array(1D array=w3011, element="Fail" ("f")) -> (index of element=w3009:i32)  [unwired: 1 in]
        n971 = Greater Or Equal To 0?(x=w3009) -> (x >= 0?=w2992:bool)
        n972 = Unbundle By Name(w3000) -> ("Total Run"=w2998:i32, "Pass"=w2997:i32, "Fail"=w2996:i32)
        n973 = Select(t=cluster{u32, u32}[] [{16748288, 16748288}] ("Colors [4]"), s=w2992, f=cluster{u32, u32}[] [{8453977, 1572626}] ("Colors [4]")) -> (s? t:f=w3005:cluster{u32, u32}[])
        n974 = Select(t="Fail" ("f"), s=w2992, f="Pass") -> (s? t:f=w3002:string)
        n975 = control-ref of="STATUS"() -> (w3008:refnum<vi>)
        n976 = property class="Bool (strict)"(reference=w3008, "Colors [4]"=w3005, "BoolText.Text"=w3002, "BoolText.FontBold"=TRUE ("Boolean Text.Font:Bold")) -> ()  [unwired: 1 in, 2 out]
        n977 = local read "EOL/FCT"() -> (w2995:bool)
        n978 = case shown="2, Default" w2991 {
          tunnel: w2995 -> [_ w3020]
          tunnel: w2994 -> [w3015 w3019]
          tunnel: [w3015 w3018] -> w2993
          tunnel: w2992 -> [_ w3016]
          frame 2, Default {
          }
          frame 1 {
            n979 = local read "Relay"() -> (w3017:refnum<queue>)
            n980 = case shown="True" w3020 {
              tunnel: w3020 -> [w3027 w3036]
              tunnel: w3019 -> [w3028 w3035]
              tunnel: [w3028 w3035] -> w3018
              tunnel: w3017 -> [w3026 w3034]
              tunnel: w3016 -> [w3025 w3031]
              frame False {
                w3024 = T28[] [enum."Tower Green"] items=["CONN_SUPPLY_%d_FCT", "HB_CONN_%d_FCT", "L_IND_CONN_%d_FCT", "R_IND_CONN_%d_FCT", "SW1_%d_FCT", "SW2_%d_FCT", "CAN_H_%d_FCT", "CAN_L_%d_FCT", "CYLINDER_ON/OFF_%d_FCT", "SPARE_1_%d_FCT", "SPARE_2_%d_FCT", "Tower Red", "Tower Amber", "Tower Green", "Tower Buzzer", "SLIMRELAY_DUT_%d_FCT", "GND_DMM_%d_EOL", "CAN_H_RES_%d_EOL", "CAN_L_RES_%d_EOL", "L_IND_RES_%d_EOL", "R_IND_RES_%d_EOL", "HB_CONN_DMM_%d_EOL", "14V_RES_%d_EOL", "CAN_L_(DMM-)_%d_EOL", "CAN_H_%d_EOL", "CAN_L_%d_EOL", "14V_%d_EOL", "GND_%d_EOL", "HB_CONN_%d_EOL", "L_IND_%d_EOL", "R_IND_%d_EOL", "CYLINDER_DUT_%d_EOL", "CYL_PB_1_%d_EOL", "CYL_PB_2_%d_EOL", "DUT_PASS_%d_EOL", "DUT_FAIL_%d_EOL", "SPARE1_%d_EOL", "Tower Red_EOL", "Tower Amber_EOL", "Tower Green_EOL", "Tower Buzzer_EOL"] ("Relay_Channel_OUT")
                w3023 = T28[] [enum."Tower Red"] items=["CONN_SUPPLY_%d_FCT", "HB_CONN_%d_FCT", "L_IND_CONN_%d_FCT", "R_IND_CONN_%d_FCT", "SW1_%d_FCT", "SW2_%d_FCT", "CAN_H_%d_FCT", "CAN_L_%d_FCT", "CYLINDER_ON/OFF_%d_FCT", "SPARE_1_%d_FCT", "SPARE_2_%d_FCT", "Tower Red", "Tower Amber", "Tower Green", "Tower Buzzer", "SLIMRELAY_DUT_%d_FCT", "GND_DMM_%d_EOL", "CAN_H_RES_%d_EOL", "CAN_L_RES_%d_EOL", "L_IND_RES_%d_EOL", "R_IND_RES_%d_EOL", "HB_CONN_DMM_%d_EOL", "14V_RES_%d_EOL", "CAN_L_(DMM-)_%d_EOL", "CAN_H_%d_EOL", "CAN_L_%d_EOL", "14V_%d_EOL", "GND_%d_EOL", "HB_CONN_%d_EOL", "L_IND_%d_EOL", "R_IND_%d_EOL", "CYLINDER_DUT_%d_EOL", "CYL_PB_1_%d_EOL", "CYL_PB_2_%d_EOL", "DUT_PASS_%d_EOL", "DUT_FAIL_%d_EOL", "SPARE1_%d_EOL", "Tower Red_EOL", "Tower Amber_EOL", "Tower Green_EOL", "Tower Buzzer_EOL"] ("Relay_Channel_OUT")
                n981 = Select(t=w3023, s=w3025, f=w3024) -> (s? t:f=w3022:T28[])
                n982 = call "Tower_lamp.vi"("FCT/EOL"=w3027, "queue IN"=w3026, "DOs"=bool[] [TRUE], "Relay_Channel_OUT"=w3022) -> ()  [unwired: 8 in]
              }
              frame True {
                w3030 = T28[] [enum."Tower Green_EOL"] items=["CONN_SUPPLY_%d_FCT", "HB_CONN_%d_FCT", "L_IND_CONN_%d_FCT", "R_IND_CONN_%d_FCT", "SW1_%d_FCT", "SW2_%d_FCT", "CAN_H_%d_FCT", "CAN_L_%d_FCT", "CYLINDER_ON/OFF_%d_FCT", "SPARE_1_%d_FCT", "SPARE_2_%d_FCT", "Tower Red", "Tower Amber", "Tower Green", "Tower Buzzer", "SLIMRELAY_DUT_%d_FCT", "GND_DMM_%d_EOL", "CAN_H_RES_%d_EOL", "CAN_L_RES_%d_EOL", "L_IND_RES_%d_EOL", "R_IND_RES_%d_EOL", "HB_CONN_DMM_%d_EOL", "14V_RES_%d_EOL", "CAN_L_(DMM-)_%d_EOL", "CAN_H_%d_EOL", "CAN_L_%d_EOL", "14V_%d_EOL", "GND_%d_EOL", "HB_CONN_%d_EOL", "L_IND_%d_EOL", "R_IND_%d_EOL", "CYLINDER_DUT_%d_EOL", "CYL_PB_1_%d_EOL", "CYL_PB_2_%d_EOL", "DUT_PASS_%d_EOL", "DUT_FAIL_%d_EOL", "SPARE1_%d_EOL", "Tower Red_EOL", "Tower Amber_EOL", "Tower Green_EOL", "Tower Buzzer_EOL"] ("Relay_Channel_OUT")
                w3032 = T28[] [enum."Tower Red_EOL"] items=["CONN_SUPPLY_%d_FCT", "HB_CONN_%d_FCT", "L_IND_CONN_%d_FCT", "R_IND_CONN_%d_FCT", "SW1_%d_FCT", "SW2_%d_FCT", "CAN_H_%d_FCT", "CAN_L_%d_FCT", "CYLINDER_ON/OFF_%d_FCT", "SPARE_1_%d_FCT", "SPARE_2_%d_FCT", "Tower Red", "Tower Amber", "Tower Green", "Tower Buzzer", "SLIMRELAY_DUT_%d_FCT", "GND_DMM_%d_EOL", "CAN_H_RES_%d_EOL", "CAN_L_RES_%d_EOL", "L_IND_RES_%d_EOL", "R_IND_RES_%d_EOL", "HB_CONN_DMM_%d_EOL", "14V_RES_%d_EOL", "CAN_L_(DMM-)_%d_EOL", "CAN_H_%d_EOL", "CAN_L_%d_EOL", "14V_%d_EOL", "GND_%d_EOL", "HB_CONN_%d_EOL", "L_IND_%d_EOL", "R_IND_%d_EOL", "CYLINDER_DUT_%d_EOL", "CYL_PB_1_%d_EOL", "CYL_PB_2_%d_EOL", "DUT_PASS_%d_EOL", "DUT_FAIL_%d_EOL", "SPARE1_%d_EOL", "Tower Red_EOL", "Tower Amber_EOL", "Tower Green_EOL", "Tower Buzzer_EOL"] ("Relay_Channel_OUT")
                n983 = Select(t=w3032, s=w3031, f=w3030) -> (s? t:f=w3029:T28[])
                n984 = call "Tower_lamp.vi"("FCT/EOL"=w3036, "queue IN"=w3034, "DOs"=bool[] [TRUE], "Relay_Channel_OUT"=w3029) -> ()  [unwired: 8 in]
              }
            }
          }
        }
        n985 = case shown="False" w2992 {
          tunnel: w3014 -> [w3044 w3052]
          tunnel: [w3043 w3051] -> w2999
          tunnel: w2998 -> [w3042 w3050]
          tunnel: w2997 -> [w3040 w3049]
          tunnel: w2996 -> [w3041 w3048]
          frame False {
            n986 = Increment(x=w3042) -> (x+1=w3039:i32)
            n987 = Increment(x=w3040) -> (x+1=w3038:i32)
            n988 = Bundle By Name(cluster=w3044, "Part Count.Total Run"=w3039, "Part Count.Pass"=w3038, "Part Count.Fail"=w3041, "ResultS"="Pass") -> (w3043:T2)
          }
          frame True {
            n989 = Increment(x=w3050) -> (x+1=w3047:i32)
            n990 = Increment(x=w3048) -> (x+1=w3046:i32)
            n991 = Bundle By Name(cluster=w3052, "Part Count.Total Run"=w3047, "Part Count.Pass"=w3049, "Part Count.Fail"=w3046, "ResultS"="Fail") -> (w3051:T2)
          }
        }
      }
      frame "Save" {
        w3080 = T28[] [enum."CONN_SUPPLY_%d_FCT", enum."HB_CONN_%d_FCT", enum."L_IND_CONN_%d_FCT", enum."R_IND_CONN_%d_FCT", enum."SW1_%d_FCT", enum."SW2_%d_FCT", enum."CAN_H_%d_FCT", enum."CAN_L_%d_FCT", enum."CYLINDER_ON/OFF_%d_FCT", enum."SPARE_1_%d_FCT", enum."SPARE_2_%d_FCT", enum."SLIMRELAY_DUT_%d_FCT"] items=["CONN_SUPPLY_%d_FCT", "HB_CONN_%d_FCT", "L_IND_CONN_%d_FCT", "R_IND_CONN_%d_FCT", "SW1_%d_FCT", "SW2_%d_FCT", "CAN_H_%d_FCT", "CAN_L_%d_FCT", "CYLINDER_ON/OFF_%d_FCT", "SPARE_1_%d_FCT", "SPARE_2_%d_FCT", "Tower Red", "Tower Amber", "Tower Green", "Tower Buzzer", "SLIMRELAY_DUT_%d_FCT", "GND_DMM_%d_EOL", "CAN_H_RES_%d_EOL", "CAN_L_RES_%d_EOL", "L_IND_RES_%d_EOL", "R_IND_RES_%d_EOL", "HB_CONN_DMM_%d_EOL", "14V_RES_%d_EOL", "CAN_L_(DMM-)_%d_EOL", "CAN_H_%d_EOL", "CAN_L_%d_EOL", "14V_%d_EOL", "GND_%d_EOL", "HB_CONN_%d_EOL", "L_IND_%d_EOL", "R_IND_%d_EOL", "CYLINDER_DUT_%d_EOL", "CYL_PB_1_%d_EOL", "CYL_PB_2_%d_EOL", "DUT_PASS_%d_EOL", "DUT_FAIL_%d_EOL", "SPARE1_%d_EOL", "Tower Red_EOL", "Tower Amber_EOL", "Tower Green_EOL", "Tower Buzzer_EOL"] ("Relay_Channel_Out")
        w3079 = T28[] [enum."GND_DMM_%d_EOL", enum."CAN_H_RES_%d_EOL", enum."CAN_L_RES_%d_EOL", enum."L_IND_RES_%d_EOL", enum."R_IND_RES_%d_EOL", enum."HB_CONN_DMM_%d_EOL", enum."14V_RES_%d_EOL", enum."CAN_L_(DMM-)_%d_EOL", enum."CAN_H_%d_EOL", enum."CAN_L_%d_EOL", enum."14V_%d_EOL", enum."GND_%d_EOL", enum."HB_CONN_%d_EOL", enum."L_IND_%d_EOL", enum."R_IND_%d_EOL", enum."CYLINDER_DUT_%d_EOL", enum."CYL_PB_1_%d_EOL", enum."CYL_PB_2_%d_EOL"] items=["CONN_SUPPLY_%d_FCT", "HB_CONN_%d_FCT", "L_IND_CONN_%d_FCT", "R_IND_CONN_%d_FCT", "SW1_%d_FCT", "SW2_%d_FCT", "CAN_H_%d_FCT", "CAN_L_%d_FCT", "CYLINDER_ON/OFF_%d_FCT", "SPARE_1_%d_FCT", "SPARE_2_%d_FCT", "Tower Red", "Tower Amber", "Tower Green", "Tower Buzzer", "SLIMRELAY_DUT_%d_FCT", "GND_DMM_%d_EOL", "CAN_H_RES_%d_EOL", "CAN_L_RES_%d_EOL", "L_IND_RES_%d_EOL", "R_IND_RES_%d_EOL", "HB_CONN_DMM_%d_EOL", "14V_RES_%d_EOL", "CAN_L_(DMM-)_%d_EOL", "CAN_H_%d_EOL", "CAN_L_%d_EOL", "14V_%d_EOL", "GND_%d_EOL", "HB_CONN_%d_EOL", "L_IND_%d_EOL", "R_IND_%d_EOL", "CYLINDER_DUT_%d_EOL", "CYL_PB_1_%d_EOL", "CYL_PB_2_%d_EOL", "DUT_PASS_%d_EOL", "DUT_FAIL_%d_EOL", "SPARE1_%d_EOL", "Tower Red_EOL", "Tower Amber_EOL", "Tower Green_EOL", "Tower Buzzer_EOL"] ("Relay_Channel_Out")
        w3130 = "_" ("string")
        n992 = Get Date/Time In Seconds() -> (seconds since 1Jan1904=w3134:timestamp)
        n993 = Unbundle By Name(w3071) -> ("Seconds"=w3060:u32, "PMC path"=w3084:path, "Barcode"=w3094:string, "Operator"=w3091:string, "ResultS"=w3090:string, "Configuration path"=w3066:path, "Header data"=w3136:string[], "Table"=w3135:string[][], "Data Path"=w3108:path, "Filename"=w3123:string, "DUT"=w3129:i32)
        n994 = Get Date/Time String(seconds (now)=w3134, want seconds? (F)=TRUE) -> (date string=w3105:string, time string=w3133:string)  [unwired: 1 in]
        n995 = Number To Decimal String(number=w3129) -> (decimal integer string=w3120:string)  [unwired: 1 in]
        n996 = Build Path(base path=w3066, name or relative path="PMC.ini") -> (appended path=w3069:path)
        n997 = Concatenate Strings("DUT" ("string"), w3120) -> (w3092:string)
        n998 = Tick Count (ms)() -> (millisecond timer value=w3061:u32)
        n999 = local read "Config"() -> (w3054:string)
        n1000 = call "INI_driver.vi"("create file if necessary (T)"=TRUE, "Enum"=T29."All_values", "instrument file path"=w3069, "Section"="Doc_ver") -> ("Values out"=w3063:string[])  [unwired: 4 in, 3 out]
        n1001 = Subtract(x=w3061, y=w3060) -> (x-y=w3059:u32)
        n1002 = call "Save2.vi"("Save Path"=w3108, "Main folder"=w3105, "DUT"=w3092, "Pass/fail"=w3090, "error in (no error)"=w3126, "Config"=w3054) -> ("Fileout"=w3106:path, "error out"=w3107:errorcluster)  [unwired: 12 in]
        n1003 = Divide(x=w3059, y=u32 1000) -> (x/y=w3057:dbl)
        n1004 = Index Array(array=w3063) -> (element=w3062:string)  [unwired: 1 in]
        n1005 = Number To Fractional String(number=w3057, precision (6)=i16 2) -> (F-format string=w3055:string)  [unwired: 2 in]
        n1006 = Search and Replace String(replace all?=TRUE ("replace all? (F)"), input string=w3133, search string=":", replace string="-" ("replace string (\"\")")) -> (result string=w3121:string)  [unwired: 4 in, 3 out]
        n1007 = Concatenate Strings(w3105, "_" ("string"), w3121) -> (w3070:string)
        n1008 = Build Array (concatenate)(w3136, w3135) -> (w3127:string[][])
        n1009 = Get Date/Time In Seconds() -> (seconds since 1Jan1904=w3102:timestamp)
        n1010 = Build Array(w3094, w3123, w3062, w3070, w3091, w3120, w3055, w3090) -> (w3119:string[])
        n1011 = Get Date/Time String(seconds (now)=w3102, want seconds? (F)=TRUE) -> (date string=w3101:string, time string=w3100:string)  [unwired: 1 in]
        n1012 = Build Path(base path=w3066, name or relative path="Report_Template.csv") -> (appended path=w3124:path)
        n1013 = Concatenate Strings(w3094, w3130, w3105, w3130, w3121) -> (w3093:string)
        n1014 = Concatenate Strings(w3093, ".csv" ("string")) -> (w3115:string)
        n1015 = Search and Replace String(replace all?=TRUE ("replace all? (F)"), input string=w3100, search string=":", replace string="-" ("replace string (\"\")")) -> (result string=w3097:string)  [unwired: 4 in, 3 out]
        n1016 = Concatenate Strings(w3101, "-" ("string"), w3097) -> (w3095:string)
        n1017 = call "SaveCSV.vi"("Data"=w3127, "Save path"=w3106, "error in (no error)"=w3107, "Tempelate path"=w3124, "Summary Details"=w3119, "Filename"=w3115) -> ("error out"=w3117:errorcluster, "all rows"=w3109:string[][])  [unwired: 3 in, 1 out]
        n1018 = call "SavePMC2.vi"("PMC path"=w3084, "Filename"=w3093, "instrument file path"=w3066, "Pass/Fail"=w3090, "Operator ID"=w3091, "error in"=w3107, "Serial no."=w3094, "Datetime"=w3095) -> ("error out"=w3088:errorcluster)  [unwired: 11 in]
        n1019 = Merge Errors(w3088, w3117) -> (w3089:errorcluster)
        n1020 = call <vilib>:"Clear Errors.vi"("error in (no error)"=w3089) -> ("error out"=w3085:errorcluster)  [unwired: 5 in, 1 out]
        n1021 = call "Specify_Path.vi"("Path_Enum"=enum16{"Find_Path", "Get_Path"}."Get_Path", "error in (no error)"=w3085) -> ("stripped path"=w3110:path, "error out"=w3116:errorcluster)  [unwired: 6 in, 6 out]
        n1022 = List Folder(path=w3110, pattern="*.py") -> (filenames=w3111:string[])  [unwired: 2 in, 3 out]
        n1023 = Empty Array?(array=w3111) -> (empty?=w3112:bool)
        n1024 = case shown="True" w3112 {
          tunnel: [w3145 w3146] -> w3073
          tunnel: w3116 -> [w3144 w3146]
          tunnel: w3106 -> [w3143 _]
          tunnel: w3093 -> [w3142 _]
          tunnel: w3111 -> [w3141 _]
          tunnel: w3110 -> [w3140 _]
          tunnel: w3109 -> [w3137 _]
          frame False {
            n1025 = Index Array(array=w3141) -> (element=w3139:string)  [unwired: 1 in]
            n1026 = Build Path(base path=w3140, name or relative path=w3139) -> (appended path=w3138:path)
            n1027 = call "PDF_Generator.vi"("all rows"=w3137, "error in (no error)"=w3144, "PDF folder Path"=w3143, "Filename"=w3142, "module path"=w3138) -> ("error out"=w3145:errorcluster)  [unwired: 6 in]
          }
          frame True {
            n1028 = One Button Dialog(message="Python File not \nfound!!!!!", button name ("OK")="OK") -> ()  [unwired: 1 out]
          }
        }
        n1029 = call <vilib>:"Clear Errors.vi"("error in (no error)"=w3073) -> ("error out"=w3072:errorcluster)  [unwired: 5 in, 1 out]
        n1030 = Unbundle By Name(w3071) -> ("DUT"=w3083:i32)
        n1031 = To Unsigned Byte Integer(number=w3083) -> (unsigned 8bit integer=w3082:u8)
        n1032 = local read "EOL/FCT"() -> (w3078:bool)
        n1033 = local read "Relay"() -> (w3081:refnum<queue>)
        n1034 = Select(t=w3079, s=w3078, f=w3080) -> (s? t:f=w3075:T28[])
        n1035 = Array Size(array=w3075) -> (size(s)=w3076:i32)
        n1036 = Initialize Array(FALSE, w3076) -> (w3074:bool[])
        n1037 = call "Relay_CYL.vi"("DUT"=w3082, "EOL/FCT"=w3078, "error out"=w3072, "DOs"=w3074, "Relay_Channel_Out"=w3075, "Relay"=w3081) -> ("error out 2"=w3053:errorcluster)  [unwired: 5 in]
      }
      frame "Print" {
        n1038 = Unbundle By Name(w3154) -> ("Barcode"=w3149:string, "ResultS"=w3153:string)
        n1039 = local read "Barcode"() -> (w3151:string)
        n1040 = Empty String/Path?(string/path=w3149) -> (empty?=w3152:bool)
        n1041 = Equal?(x=w3153, y="Pass" ("ResultS")) -> (x = y?=w3157:bool)
        n1042 = Select(t=w3151, s=w3152, f=w3149) -> (s? t:f=w3150:string)
        n1043 = case shown="True" w3157 {
          tunnel: w3156 -> [w3160 w3163]
          tunnel: [w3160 w3162] -> w3158
          tunnel: w3150 -> [_ w3161]
          frame False {
          }
          frame True {
            n1044 = call "Printer_Driver.vi"("error in"=w3163, "Serial Number"=w3161) -> ("error out"=w3162:errorcluster)  [unwired: 6 in, 3 out]
          }
        }
        n1045 = call <vilib>:"Clear Errors.vi"("error in (no error)"=w3158) -> ("error out"=w3155:errorcluster)  [unwired: 5 in, 1 out]
      }
      frame "Reset" {
        w3172 = string[][] [] ("Value")
        w3165 = "" ("Barcode")
        # "Tower Amber\nTower Red\nTower Green\nTower Buzzer"
        n1046 = Unbundle By Name(w3167) -> ("DUT"=w3166:i32)
        n1047 = flat-sequence {
          tunnel: w3169 -> [w3187]
          tunnel: [w3187] -> w3168
          tunnel: w3166 -> [w3180]
          frame #0 {
            w3182 = T28[] [enum."Tower Amber", enum."Tower Red", enum."Tower Green", enum."Tower Buzzer"] items=["CONN_SUPPLY_%d_FCT", "HB_CONN_%d_FCT", "L_IND_CONN_%d_FCT", "R_IND_CONN_%d_FCT", "SW1_%d_FCT", "SW2_%d_FCT", "CAN_H_%d_FCT", "CAN_L_%d_FCT", "CYLINDER_ON/OFF_%d_FCT", "SPARE_1_%d_FCT", "SPARE_2_%d_FCT", "Tower Red", "Tower Amber", "Tower Green", "Tower Buzzer", "SLIMRELAY_DUT_%d_FCT", "GND_DMM_%d_EOL", "CAN_H_RES_%d_EOL", "CAN_L_RES_%d_EOL", "L_IND_RES_%d_EOL", "R_IND_RES_%d_EOL", "HB_CONN_DMM_%d_EOL", "14V_RES_%d_EOL", "CAN_L_(DMM-)_%d_EOL", "CAN_H_%d_EOL", "CAN_L_%d_EOL", "14V_%d_EOL", "GND_%d_EOL", "HB_CONN_%d_EOL", "L_IND_%d_EOL", "R_IND_%d_EOL", "CYLINDER_DUT_%d_EOL", "CYL_PB_1_%d_EOL", "CYL_PB_2_%d_EOL", "DUT_PASS_%d_EOL", "DUT_FAIL_%d_EOL", "SPARE1_%d_EOL", "Tower Red_EOL", "Tower Amber_EOL", "Tower Green_EOL", "Tower Buzzer_EOL"] ("f")
            w3183 = T28[] [enum."Tower Amber_EOL", enum."Tower Red_EOL", enum."Tower Green_EOL", enum."Tower Buzzer_EOL"] items=["CONN_SUPPLY_%d_FCT", "HB_CONN_%d_FCT", "L_IND_CONN_%d_FCT", "R_IND_CONN_%d_FCT", "SW1_%d_FCT", "SW2_%d_FCT", "CAN_H_%d_FCT", "CAN_L_%d_FCT", "CYLINDER_ON/OFF_%d_FCT", "SPARE_1_%d_FCT", "SPARE_2_%d_FCT", "Tower Red", "Tower Amber", "Tower Green", "Tower Buzzer", "SLIMRELAY_DUT_%d_FCT", "GND_DMM_%d_EOL", "CAN_H_RES_%d_EOL", "CAN_L_RES_%d_EOL", "L_IND_RES_%d_EOL", "R_IND_RES_%d_EOL", "HB_CONN_DMM_%d_EOL", "14V_RES_%d_EOL", "CAN_L_(DMM-)_%d_EOL", "CAN_H_%d_EOL", "CAN_L_%d_EOL", "14V_%d_EOL", "GND_%d_EOL", "HB_CONN_%d_EOL", "L_IND_%d_EOL", "R_IND_%d_EOL", "CYLINDER_DUT_%d_EOL", "CYL_PB_1_%d_EOL", "CYL_PB_2_%d_EOL", "DUT_PASS_%d_EOL", "DUT_FAIL_%d_EOL", "SPARE1_%d_EOL", "Tower Red_EOL", "Tower Amber_EOL", "Tower Green_EOL", "Tower Buzzer_EOL"] ("Relay_Channel_OUT")
            n1048 = local read "EOL/FCT"() -> (w3181:bool)
            n1049 = Select(t=w3183, s=w3181, f=w3182) -> (s? t:f=w3184:T28[])
            n1050 = local read "Relay"() -> (w3185:refnum<queue>)
            n1051 = call "Relay_CYL.vi"("DUT"=w3180, "EOL/FCT"=w3181, "DOs"=bool[] [TRUE, FALSE, FALSE, FALSE], "Relay_Channel_Out"=w3184, "Relay"=w3185) -> ()  [unwired: 6 in, 1 out]
          }
        }
        n1052 = control-ref of="STATUS"() -> (w3178:refnum<vi>)
        n1053 = property class="Bool (strict)"(reference=w3178, "Colors [4]"=cluster{u32, u32}[] [{13816530, 13816530}], "BoolText.Text"="IDLE.." ("Boolean Text.Text")) -> ()  [unwired: 1 in, 2 out]
        n1054 = local write "Total Time(s)"(0 ("Total Time(s)")) -> ()
        n1055 = control-ref of="Table"() -> (w3174:refnum<vi>)
        n1056 = local write "DTU Inspection Data"(w3165) -> ()
        n1057 = property on="Barcode" class="Str"("Value"=w3165) -> ()  [unwired: 2 in, 2 out]
        n1058 = property class="Tbl (strict)"(reference=w3174, "Value"=w3172) -> ()  [unwired: 1 in, 2 out]
        n1059 = Bundle By Name(cluster=w3167, "Barcode Scanned?"=FALSE, "Barcode"=w3165, "Table"=w3172) -> (w3173:T2)
        n1060 = call "Test_Enque_Message_FGV.vi"("error in (no error)"=w3168, "Message"="Update Display", "queue in"=w3176) -> ("error out"=w3175:errorcluster)  [unwired: 8 in]
      }
      frame "EmergencyReset" {
        (unwired) "Aborted" ("Filename")
        (unwired) "Fail" ("ResultS")
        w3195 = T28[] [enum."CONN_SUPPLY_%d_FCT", enum."HB_CONN_%d_FCT", enum."L_IND_CONN_%d_FCT", enum."R_IND_CONN_%d_FCT", enum."SW1_%d_FCT", enum."SW2_%d_FCT", enum."CAN_H_%d_FCT", enum."CAN_L_%d_FCT", enum."CYLINDER_ON/OFF_%d_FCT", enum."SPARE_1_%d_FCT", enum."SPARE_2_%d_FCT", enum."SLIMRELAY_DUT_%d_FCT"] items=["CONN_SUPPLY_%d_FCT", "HB_CONN_%d_FCT", "L_IND_CONN_%d_FCT", "R_IND_CONN_%d_FCT", "SW1_%d_FCT", "SW2_%d_FCT", "CAN_H_%d_FCT", "CAN_L_%d_FCT", "CYLINDER_ON/OFF_%d_FCT", "SPARE_1_%d_FCT", "SPARE_2_%d_FCT", "Tower Red", "Tower Amber", "Tower Green", "Tower Buzzer", "SLIMRELAY_DUT_%d_FCT", "GND_DMM_%d_EOL", "CAN_H_RES_%d_EOL", "CAN_L_RES_%d_EOL", "L_IND_RES_%d_EOL", "R_IND_RES_%d_EOL", "HB_CONN_DMM_%d_EOL", "14V_RES_%d_EOL", "CAN_L_(DMM-)_%d_EOL", "CAN_H_%d_EOL", "CAN_L_%d_EOL", "14V_%d_EOL", "GND_%d_EOL", "HB_CONN_%d_EOL", "L_IND_%d_EOL", "R_IND_%d_EOL", "CYLINDER_DUT_%d_EOL", "CYL_PB_1_%d_EOL", "CYL_PB_2_%d_EOL", "DUT_PASS_%d_EOL", "DUT_FAIL_%d_EOL", "SPARE1_%d_EOL", "Tower Red_EOL", "Tower Amber_EOL", "Tower Green_EOL", "Tower Buzzer_EOL"] ("Relay_Channel_Out")
        w3194 = T28[] [enum."GND_DMM_%d_EOL", enum."CAN_H_RES_%d_EOL", enum."CAN_L_RES_%d_EOL", enum."L_IND_RES_%d_EOL", enum."R_IND_RES_%d_EOL", enum."HB_CONN_DMM_%d_EOL", enum."14V_RES_%d_EOL", enum."CAN_L_(DMM-)_%d_EOL", enum."CAN_H_%d_EOL", enum."CAN_L_%d_EOL", enum."14V_%d_EOL", enum."GND_%d_EOL", enum."HB_CONN_%d_EOL", enum."L_IND_%d_EOL", enum."R_IND_%d_EOL", enum."CYLINDER_DUT_%d_EOL", enum."CYL_PB_1_%d_EOL", enum."CYL_PB_2_%d_EOL"] items=["CONN_SUPPLY_%d_FCT", "HB_CONN_%d_FCT", "L_IND_CONN_%d_FCT", "R_IND_CONN_%d_FCT", "SW1_%d_FCT", "SW2_%d_FCT", "CAN_H_%d_FCT", "CAN_L_%d_FCT", "CYLINDER_ON/OFF_%d_FCT", "SPARE_1_%d_FCT", "SPARE_2_%d_FCT", "Tower Red", "Tower Amber", "Tower Green", "Tower Buzzer", "SLIMRELAY_DUT_%d_FCT", "GND_DMM_%d_EOL", "CAN_H_RES_%d_EOL", "CAN_L_RES_%d_EOL", "L_IND_RES_%d_EOL", "R_IND_RES_%d_EOL", "HB_CONN_DMM_%d_EOL", "14V_RES_%d_EOL", "CAN_L_(DMM-)_%d_EOL", "CAN_H_%d_EOL", "CAN_L_%d_EOL", "14V_%d_EOL", "GND_%d_EOL", "HB_CONN_%d_EOL", "L_IND_%d_EOL", "R_IND_%d_EOL", "CYLINDER_DUT_%d_EOL", "CYL_PB_1_%d_EOL", "CYL_PB_2_%d_EOL", "DUT_PASS_%d_EOL", "DUT_FAIL_%d_EOL", "SPARE1_%d_EOL", "Tower Red_EOL", "Tower Amber_EOL", "Tower Green_EOL", "Tower Buzzer_EOL"] ("Relay_Channel_Out")
        # "Emergency Stop or Abort button"
        n1061 = Unbundle By Name(w3202) -> ("Array_Q"=w3201:refnum<queue>[])
        n1062 = property on="Start Button" class="Bool"(error in=w3209, "DisabledEnum"=T31."Enabled" ("Disabled")) -> (error out=w3208:errorcluster)  [unwired: 1 in, 1 out]
        n1063 = flat-sequence {
          tunnel: w3208 -> [w3235]
          tunnel: [w3234] -> w3200
          tunnel: w3204 -> [w3233]
          tunnel: [w3232] -> w3203
          frame #0 {
            n1064 = Flush Queue(queue=w3233, error in (no error)=w3235) -> (queue out=w3232:refnum<queue>, error out=w3234:errorcluster)  [unwired: 1 out]
          }
        }
        n1065 = control-ref of="STATUS"() -> (w3214:refnum<vi>)
        n1066 = for {
          shift-right: [w3224] -> w3199
          shift-left: w3200 -> [w3225]
          tunnel: w3201 -> [w3220] mode=indexing
          n1067 = Bundle(cluster=T25 {"Message"="", "Message Data"=variant} ("element"), "Message"="Reset") -> (w3221:T25)  [unwired: 1 in]
          n1068 = Enqueue Element(queue=w3220, element=w3221, error in (no error)=w3225) -> (error out=w3224:errorcluster)  [unwired: 1 in, 2 out]
        }
        n1069 = property class="Bool (strict)"(reference=w3214, "Colors [4]"=cluster{u32, u32}[] [{16711680, 16711680}], "BoolText.Text"="ABORTED" ("Boolean Text.Text"), "BoolText.FontBold"=TRUE ("Boolean Text.Font:Bold")) -> ()  [unwired: 1 in, 2 out]
        n1070 = Unbundle By Name(w3202) -> ("DUT"=w3198:i32)
        n1071 = To Unsigned Byte Integer(number=w3198) -> (unsigned 8bit integer=w3197:u8)
        n1072 = local read "EOL/FCT"() -> (w3193:bool)
        n1073 = local read "Relay"() -> (w3196:refnum<queue>)
        n1074 = Select(t=w3194, s=w3193, f=w3195) -> (s? t:f=w3190:T28[])
        n1075 = Array Size(array=w3190) -> (size(s)=w3191:i32)
        n1076 = Initialize Array(FALSE, w3191) -> (w3189:bool[])
        n1077 = call "Relay_CYL.vi"("DUT"=w3197, "EOL/FCT"=w3193, "error out"=w3199, "DOs"=w3189, "Relay_Channel_Out"=w3190, "Relay"=w3196) -> ("error out 2"=w3210:errorcluster)  [unwired: 5 in]
        n1078 = local read "Configs"() -> (w3188:string)
        n1079 = disable-structure shown="Enabled" {
          disable-tunnel: [w3229 w3231] -> w3218
          disable-tunnel: [w3227 w3230] -> w3217
          disable-tunnel: w3210 -> [w3226 w3231]
          disable-tunnel: w3203 -> [_ w3230]
          frame Disabled {
            n1080 = call "Test_Queue_Comm_FGV.vi"("error in (no error)"=w3226, "Enum"=Test_FGV_Queue_Control."Get") -> ("error Out"=w3229:errorcluster, "queue Out"=w3227:refnum<queue>)  [unwired: 8 in]
          }
          frame Enabled {
          }
        }
        n1081 = Bundle By Name(cluster=w3202, "ResultS"="Aborted", "Filename"=w3188) -> (w3206:T2)
        n1082 = call "Test_Enqueue Message (Array).vi"("error in (no error)"=w3218, "Message Array"=string[] ["StopTest", "Update Display", "Save"], "Message Queue"=w3217) -> ("error out"=w3216:errorcluster)  [unwired: 7 in, 1 out]
        n1083 = Merge Errors(w3216) -> (w3219:errorcluster)
      }
      frame "Emergency" {
        w3246 = T28[] [enum."CONN_SUPPLY_%d_FCT", enum."HB_CONN_%d_FCT", enum."L_IND_CONN_%d_FCT", enum."R_IND_CONN_%d_FCT", enum."SW1_%d_FCT", enum."SW2_%d_FCT", enum."CAN_H_%d_FCT", enum."CAN_L_%d_FCT", enum."CYLINDER_ON/OFF_%d_FCT", enum."SPARE_1_%d_FCT", enum."SPARE_2_%d_FCT", enum."SLIMRELAY_DUT_%d_FCT"] items=["CONN_SUPPLY_%d_FCT", "HB_CONN_%d_FCT", "L_IND_CONN_%d_FCT", "R_IND_CONN_%d_FCT", "SW1_%d_FCT", "SW2_%d_FCT", "CAN_H_%d_FCT", "CAN_L_%d_FCT", "CYLINDER_ON/OFF_%d_FCT", "SPARE_1_%d_FCT", "SPARE_2_%d_FCT", "Tower Red", "Tower Amber", "Tower Green", "Tower Buzzer", "SLIMRELAY_DUT_%d_FCT", "GND_DMM_%d_EOL", "CAN_H_RES_%d_EOL", "CAN_L_RES_%d_EOL", "L_IND_RES_%d_EOL", "R_IND_RES_%d_EOL", "HB_CONN_DMM_%d_EOL", "14V_RES_%d_EOL", "CAN_L_(DMM-)_%d_EOL", "CAN_H_%d_EOL", "CAN_L_%d_EOL", "14V_%d_EOL", "GND_%d_EOL", "HB_CONN_%d_EOL", "L_IND_%d_EOL", "R_IND_%d_EOL", "CYLINDER_DUT_%d_EOL", "CYL_PB_1_%d_EOL", "CYL_PB_2_%d_EOL", "DUT_PASS_%d_EOL", "DUT_FAIL_%d_EOL", "SPARE1_%d_EOL", "Tower Red_EOL", "Tower Amber_EOL", "Tower Green_EOL", "Tower Buzzer_EOL"] ("Relay_Channel_Out")
        w3245 = T28[] [enum."GND_DMM_%d_EOL", enum."CAN_H_RES_%d_EOL", enum."CAN_L_RES_%d_EOL", enum."L_IND_RES_%d_EOL", enum."R_IND_RES_%d_EOL", enum."HB_CONN_DMM_%d_EOL", enum."14V_RES_%d_EOL", enum."CAN_L_(DMM-)_%d_EOL", enum."CAN_H_%d_EOL", enum."CAN_L_%d_EOL", enum."14V_%d_EOL", enum."GND_%d_EOL", enum."HB_CONN_%d_EOL", enum."L_IND_%d_EOL", enum."R_IND_%d_EOL", enum."CYLINDER_DUT_%d_EOL", enum."CYL_PB_1_%d_EOL", enum."CYL_PB_2_%d_EOL"] items=["CONN_SUPPLY_%d_FCT", "HB_CONN_%d_FCT", "L_IND_CONN_%d_FCT", "R_IND_CONN_%d_FCT", "SW1_%d_FCT", "SW2_%d_FCT", "CAN_H_%d_FCT", "CAN_L_%d_FCT", "CYLINDER_ON/OFF_%d_FCT", "SPARE_1_%d_FCT", "SPARE_2_%d_FCT", "Tower Red", "Tower Amber", "Tower Green", "Tower Buzzer", "SLIMRELAY_DUT_%d_FCT", "GND_DMM_%d_EOL", "CAN_H_RES_%d_EOL", "CAN_L_RES_%d_EOL", "L_IND_RES_%d_EOL", "R_IND_RES_%d_EOL", "HB_CONN_DMM_%d_EOL", "14V_RES_%d_EOL", "CAN_L_(DMM-)_%d_EOL", "CAN_H_%d_EOL", "CAN_L_%d_EOL", "14V_%d_EOL", "GND_%d_EOL", "HB_CONN_%d_EOL", "L_IND_%d_EOL", "R_IND_%d_EOL", "CYLINDER_DUT_%d_EOL", "CYL_PB_1_%d_EOL", "CYL_PB_2_%d_EOL", "DUT_PASS_%d_EOL", "DUT_FAIL_%d_EOL", "SPARE1_%d_EOL", "Tower Red_EOL", "Tower Amber_EOL", "Tower Green_EOL", "Tower Buzzer_EOL"] ("Relay_Channel_Out")
        # "Emergency Button pressed"
        n1084 = property on="Start Button" class="Bool"(error in=w3258, "DisabledEnum"=T31."Enabled" ("Disabled")) -> (error out=w3257:errorcluster)  [unwired: 1 in, 1 out]
        n1085 = Unbundle By Name(w3249) -> ("Array_Q"=w3248:refnum<queue>[])
        n1086 = flat-sequence {
          tunnel: w3257 -> [w3283]
          tunnel: [w3282] -> w3250
          tunnel: w3252 -> [w3281]
          tunnel: [w3280] -> w3251
          frame #0 {
            n1087 = Flush Queue(queue=w3281, error in (no error)=w3283) -> (queue out=w3280:refnum<queue>, error out=w3282:errorcluster)  [unwired: 1 out]
          }
        }
        n1088 = control-ref of="STATUS"() -> (w3262:refnum<vi>)
        n1089 = for {
          shift-right: [w3272] -> w3243
          shift-left: w3250 -> [w3273]
          tunnel: w3248 -> [w3268] mode=indexing
          n1090 = Bundle(cluster=T25 {"Message"="", "Message Data"=variant} ("element"), "Message"="Reset") -> (w3269:T25)  [unwired: 1 in]
          n1091 = Enqueue Element(queue=w3268, element=w3269, error in (no error)=w3273) -> (error out=w3272:errorcluster)  [unwired: 1 in, 2 out]
        }
        n1092 = property class="Bool (strict)"(reference=w3262, "Colors [4]"=cluster{u32, u32}[] [{16711680, 16711680}], "BoolText.Text"="ABORTED" ("Boolean Text.Text"), "BoolText.FontBold"=TRUE ("Boolean Text.Font:Bold")) -> ()  [unwired: 1 in, 2 out]
        n1093 = Unbundle By Name(w3249) -> ("DUT"=w3244:i32)
        n1094 = local read "EOL/FCT"() -> (w3237:bool)
        n1095 = local read "Relay"() -> (w3238:refnum<queue>)
        n1096 = To Unsigned Byte Integer(number=w3244) -> (unsigned 8bit integer=w3247:u8)
        n1097 = Select(t=w3245, s=w3237, f=w3246) -> (s? t:f=w3236:T28[])
        n1098 = Array Size(array=w3236) -> (size(s)=w3240:i32)
        n1099 = Initialize Array(FALSE, w3240) -> (w3239:bool[])
        n1100 = call "Relay_CYL.vi"("DUT"=w3247, "EOL/FCT"=w3237, "error out"=w3243, "DOs"=w3239, "Relay_Channel_Out"=w3236, "Relay"=w3238) -> ("error out 2"=w3242:errorcluster)  [unwired: 5 in]
        n1101 = disable-structure shown="Enabled" {
          disable-tunnel: [w3277 w3279] -> w3266
          disable-tunnel: [w3275 w3278] -> w3265
          disable-tunnel: w3242 -> [w3274 w3279]
          disable-tunnel: w3251 -> [_ w3278]
          frame Disabled {
            n1102 = call "Test_Queue_Comm_FGV.vi"("error in (no error)"=w3274, "Enum"=Test_FGV_Queue_Control."Get") -> ("error Out"=w3277:errorcluster, "queue Out"=w3275:refnum<queue>)  [unwired: 8 in]
          }
          frame Enabled {
          }
        }
        n1103 = Bundle By Name(cluster=w3249, "ResultS"="Fail", "Filename"="Aborted") -> (w3255:T2)
        n1104 = call "Test_Enqueue Message (Array).vi"("error in (no error)"=w3266, "Message Array"=string[] ["StopTest", "Update Display", "Save"], "Message Queue"=w3265) -> ("error out"=w3264:errorcluster)  [unwired: 7 in, 1 out]
        n1105 = Merge Errors(w3264) -> (w3267:errorcluster)
      }
      frame "Update Display" {
        # "Update display"
        n1106 = Unbundle By Name(w3286) -> ("Table"=w3285:string[][], "Barcode"=w3284:string)
        n1107 = property on="Table" class="Tbl (strict)"("Value"=w3285) -> ()  [unwired: 2 in, 2 out]
        n1108 = local write "Barcode"(w3284) -> ()
        n1109 = Merge Errors(w3287) -> (w3288:errorcluster)
      }
      frame "Error" {
        # "Error - Display an error dialog. This message is sent by the \"Error Handler\" VIs at the end of other loops in this application."
        n1110 = Variant To Data(error in=w3305, type=errorcluster {"status"=FALSE, "code"=0, "source"=""} ("error constant"), Variant=w3304) -> (data=w3302:errorcluster, error out=w3301:errorcluster)
        n1111 = call <vilib>:"Simple Error Handler.vi"("error in (no error)"=w3302) -> ()  [unwired: 4 in, 5 out]
        n1112 = call <vilib>:"Clear Errors.vi"("error in (no error)"=w3301) -> ("error out"=w3298:errorcluster)  [unwired: 5 in, 1 out]
        n1113 = Unbundle By Name(w3295) -> ("Stepno."=w3290:u64, "Test2_Q"=w3293:refnum<queue>)
        n1114 = Flush Queue(queue=w3293, error in (no error)=w3298) -> (queue out=w3292:refnum<queue>, error out=w3294:errorcluster)  [unwired: 1 out]
        n1115 = disable-structure shown="Enabled" {
          disable-tunnel: w3290 -> [w3307 w3308]
          disable-tunnel: [w3306 w3308] -> w3289
          frame Disabled {
            n1116 = Increment(x=w3307) -> (x+1=w3306:u64)
          }
          frame Enabled {
          }
        }
        n1117 = Bundle By Name(cluster=w3295, "Stepno."=w3289) -> (w3291:T2)
        n1118 = call "Test_Enque_Message_FGV.vi"("Priority"=TRUE ("Priority Message? (F)"), "error in (no error)"=w3294, "Message"="IndexStep", "queue in"=w3292) -> ("error out"=w3297:errorcluster)  [unwired: 7 in]
        n1119 = Merge Errors(w3297) -> (w3300:errorcluster)
      }
      frame "Confirm Quit" {
        # "Confirm Quit - Message that can confirm whether or not the user wants to exit the application."
        n1120 = Unbundle By Name(w3311) -> ("Array_Q"=w3310:refnum<queue>[], "Relay_Module_Q"=w3309:refnum<queue>)
        n1121 = Bundle(cluster=T25 {"Message"="", "Message Data"=variant} ("element"), "Message"="Exit") -> (w3315:T25)  [unwired: 1 in]
        n1122 = Enqueue Element(queue=w3309, element=w3315, error in (no error)=w3321) -> (error out=w3313:errorcluster)  [unwired: 1 in, 2 out]
        n1123 = for {
          shift-right: [w3328] -> w3312
          shift-left: w3313 -> [w3329]
          tunnel: w3310 -> [w3324] mode=indexing
          n1124 = Bundle(cluster=T25 {"Message"="", "Message Data"=variant} ("element"), "Message"="Confirm Quit") -> (w3325:T25)  [unwired: 1 in]
          n1125 = Enqueue Element(queue=w3324, element=w3325, error in (no error)=w3329) -> (error out=w3328:errorcluster)  [unwired: 1 in, 2 out]
        }
        n1126 = call <vilib>:"Clear Errors.vi"("error in (no error)"=w3312) -> ("error out"=w3317:errorcluster)  [unwired: 5 in, 1 out]
        n1127 = call "Test_Enque_Message_FGV.vi"("Priority"=TRUE ("Priority Message? (F)"), "error in (no error)"=w3317, "Message"="Exit", "queue in"=w3318) -> ("error out"=w3322:errorcluster)  [unwired: 7 in]
        n1128 = Merge Errors(w3322) -> (w3323:errorcluster)
      }
      frame "Exit" {
        (unwired) TRUE ("Priority Message? (F)")
        # "Exit - Exit the application."
        n1129 = Unbundle By Name(w3332) -> ("Array_Q"=w3333:refnum<queue>[])
        n1130 = for {
          shift-right: [w3343] -> w3330
          shift-left: w3334 -> [w3344]
          tunnel: w3333 -> [w3342] mode=indexing
          n1131 = Release Queue(queue=w3342, error in (no error)=w3344) -> (error out=w3343:errorcluster)  [unwired: 1 in, 2 out]
        }
        n1132 = call "Test_Queue_Comm_FGV.vi"("error in (no error)"=w3330, "Enum"=Test_FGV_Queue_Control."Release", "queue in"=w3335) -> ("error Out"=w3338:errorcluster)  [unwired: 7 in, 1 out]
        n1133 = call "Test_Fire User Event - Stop.vi"("User Event - Stop"=w3337) -> ("error out"=w3336:errorcluster)  [unwired: 10 in]
        n1134 = Merge Errors(w3336, w3338) -> (w3340:errorcluster)
        n1135 = call <vilib>:"Clear Errors.vi"("error in (no error)"=w3340) -> ("error out"=w3331:errorcluster)  [unwired: 5 in, 1 out]
      }
      frame Default {
        # "'Default' case only runs if there is a message that isn't defined in any of the other cases.  Output a programming error."
        n1136 = xnode "Error Ring"("parameter 0"=w3345) -> ("error out"=w3346:errorcluster)
      }
    }
    n1137 = call "Test_Error_Handler_MHL_FGV.vi"("error in (no error)"=w449, "queue in"=w446) -> ("error Out"=w448:errorcluster)  [unwired: 9 in]
  }
  n1138 = Tick Count (ms)() -> ()  [unwired: 1 out]
  n1139 = Unregister For Events(event registration refnum=w25, error in=w23) -> (error out=w26:errorcluster)
  n1140 = Merge Errors(w26, w29) -> (w27:errorcluster)
  n1141 = call "Test_Destroy User Event - Stop.vi"("error in (no error)"=w27, "User Event - Stop"=w2) -> ("error out"=→"error in (out)":errorcluster)  [unwired: 9 in]
